vi "MICS Wakeup Calibration Tool.vi"(8 "error in (no error)":errorcluster, 10 "SECONDARY MICS Dongle Address":refnum<visa-resource-name>="COM8", 11 "PRIMARY MICS Dongle Address":refnum<visa-resource-name>="COM8") -> (0 "error out":errorcluster, 2 "Trim Settings":string)   [LabVIEW 2020]
panel:
  in  "Reject Ratio, %":i32=75
  in  "RSSI Gain":enum16{"1", "3", "10", "30"}(ring)
  in  "WakeupMode":bool=TRUE
  in  "DetTrim":bool=TRUE
  in  "Wakeup Signal Transmit":bool
  in  "Samples to Average":u8=5 format="%02d"
  out "Retries":u8 format="%02d"
  out "Loopback Data":u8 format="%02x"
  in  "Loopback Detector":bool
  in  "Update Radio Settings":bool
  in  "Done":bool
  in  "Do RSSI":bool
  out "RSSI Reading":u8(knob) scale=0.0..31.0 scale format="%x"
  in  "Detector Offset Trim":u8(knob)=31 scale=0.0..63.0 scale format="%x"
  in  "Wakeup Signal Power, dBm":dbl(knob)=-32.0 min=-32.25 max=0.0 step=0.25
  in  "RSSI Fine Trim":u8(knob)=16 scale=0.0..31.0 scale format="%x"
  in  "RX Antenna Tune":u8(knob)=7 scale=0.0..15.0 scale format="%x"
  in  "LNA Frequency Trim":u8(knob)=15 scale=0.0..31.0 scale format="%x"
  in  "LNA Gain Trim":u8(knob)=20 scale=0.0..63.0 scale format="%x"
  # "CW RF"
  # "Wakeup Packet"
  # "RF Trim"
  # "Detector Trim"
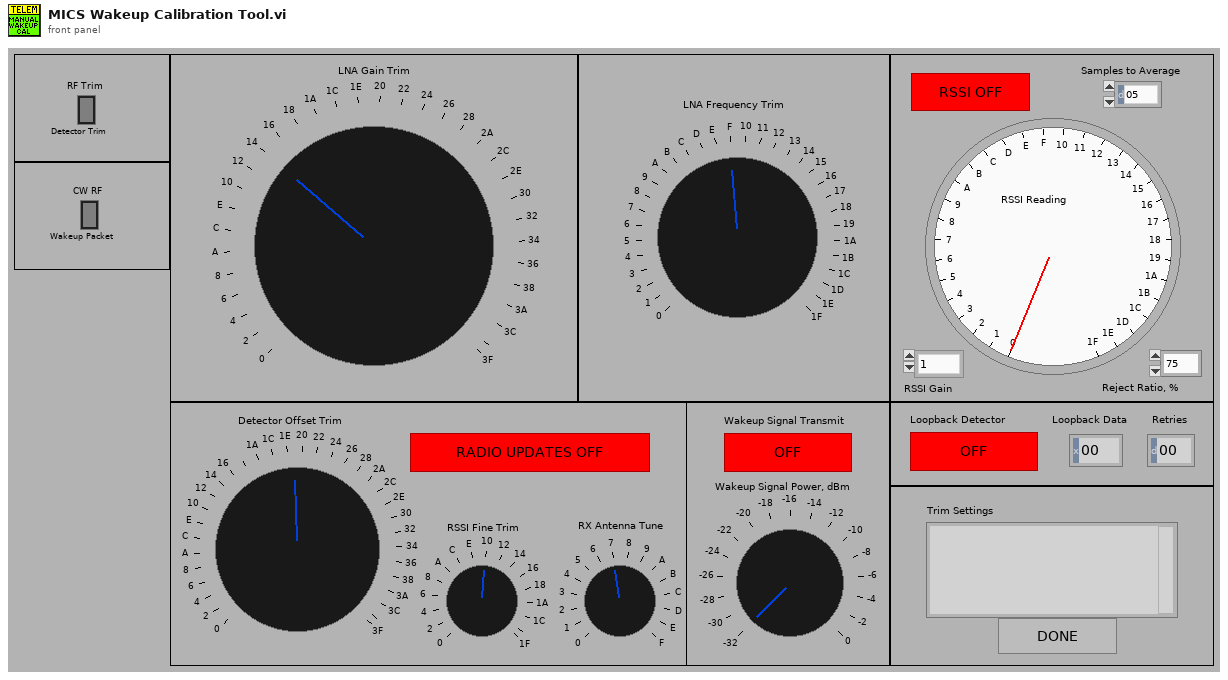
[diagram p1: front panel]
types:
  T1 = cluster{"ConfigFlags":u8, "ImplantID":u32, "CompanyID":u8, "Normal_Comm":cluster{"RF_Channel":u8, "UserData":u8, "TX_Mod":u8, "RX_Mod":u8, "RX_BlockSize":u8, "BlockPerPack":u8, "TX_BlockSize":u8}, "Emerg_Comm":cluster{"RF_Channel":u8, "UserData":u8, "TX_Mod":u8, "RX_Mod":u8, "TX_BlockSize":u8, "BlockPerPack":u8, "RX_BlockSize":u8}, "ImplantRev":u8, "245TX_PowerCal":i8, "245TX_Power":i8, "CCA_RSSI_Thresholds":cluster{"ch0":u16, "ch1":u16, "ch2":u16, "ch3":u16, "ch4":u16, "ch5":u16, "ch6":u16, "ch7":u16, "ch8":u16, "ch9":u16}}
  T2 = enum16{"Start Search", "Continue Search", "End Search"}
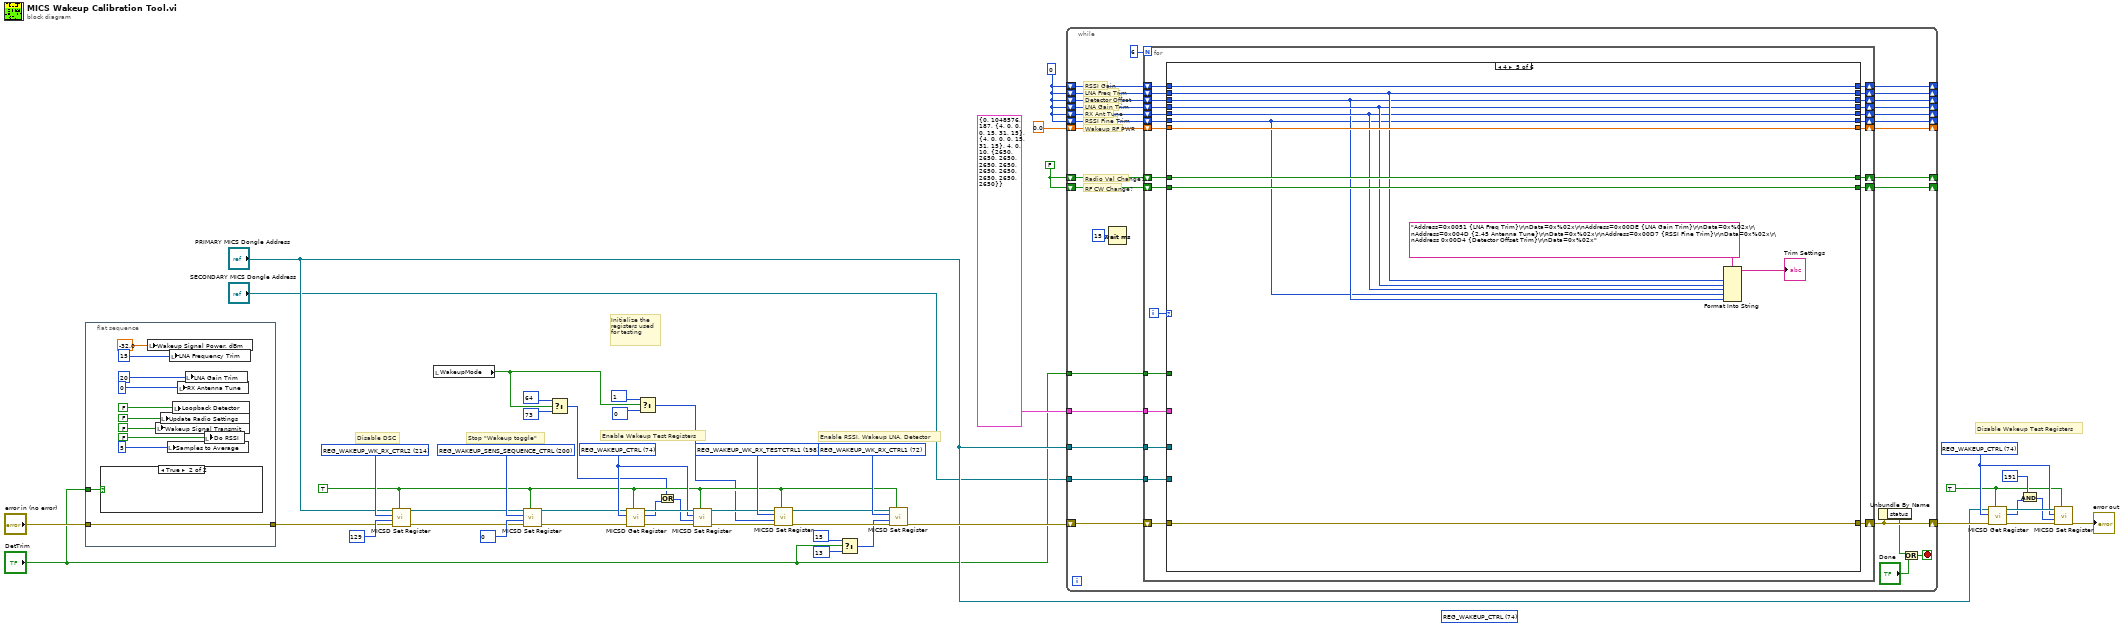
[diagram p0: block diagram]
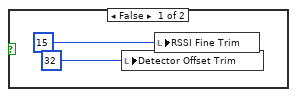
[diagram p2: hidden frame]
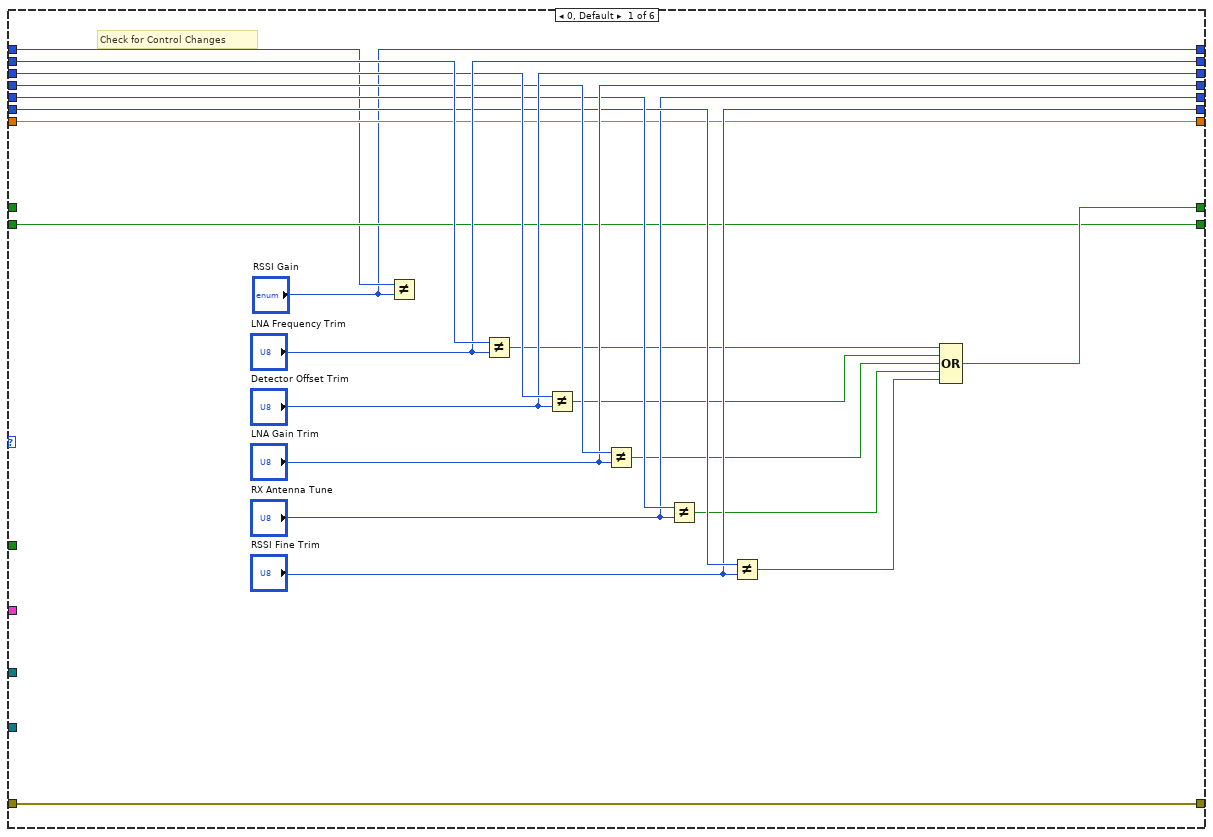
[diagram p3: hidden frame]
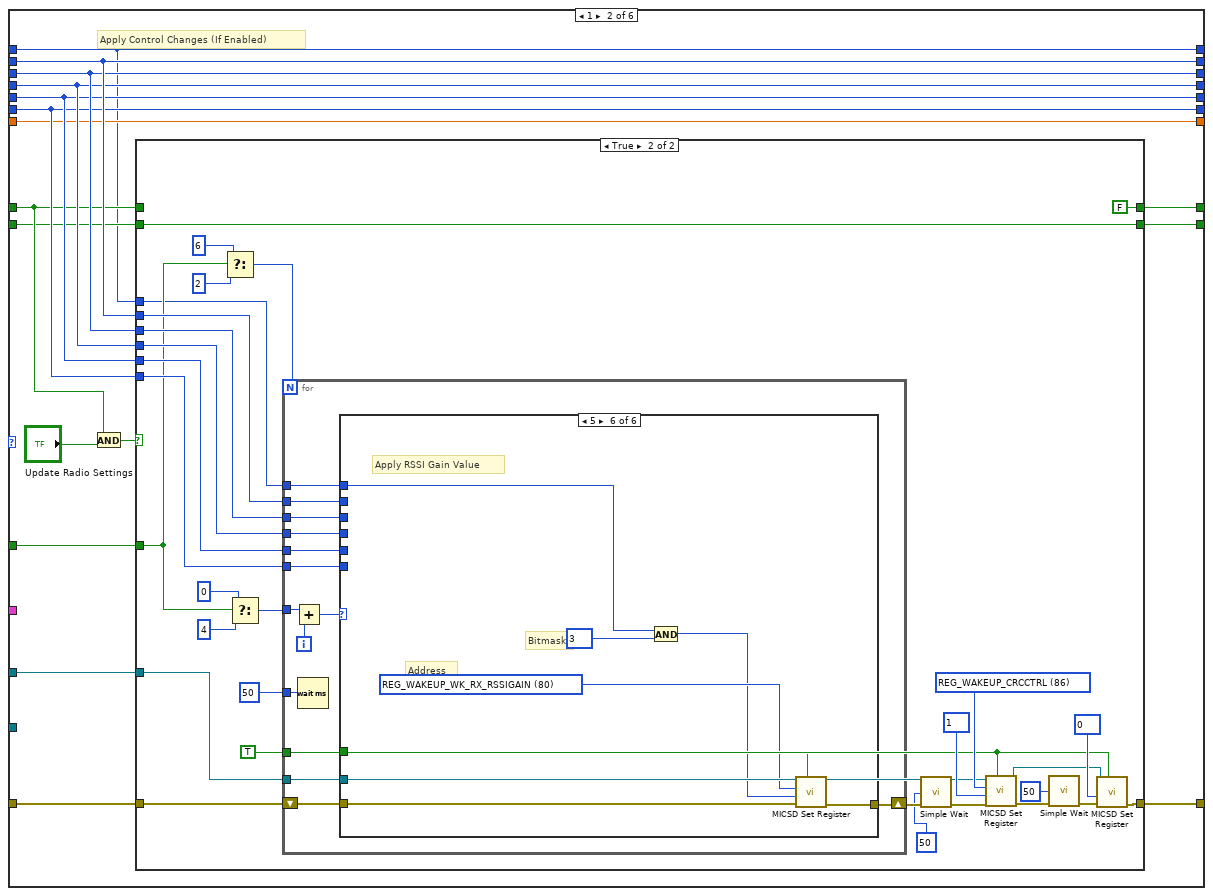
[diagram p4: hidden frame]
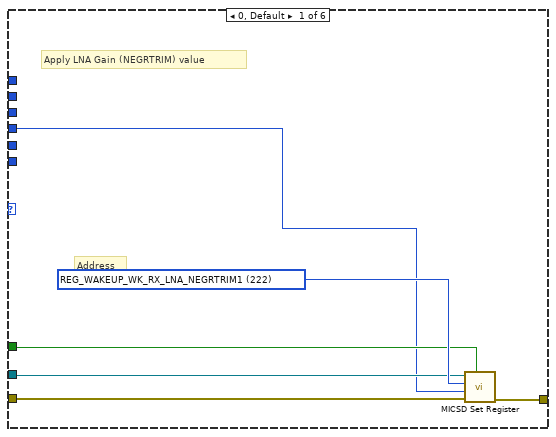
[diagram p6: hidden frame]
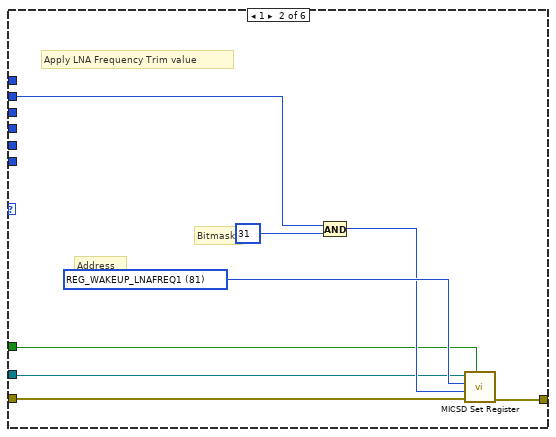
[diagram p7: hidden frame]
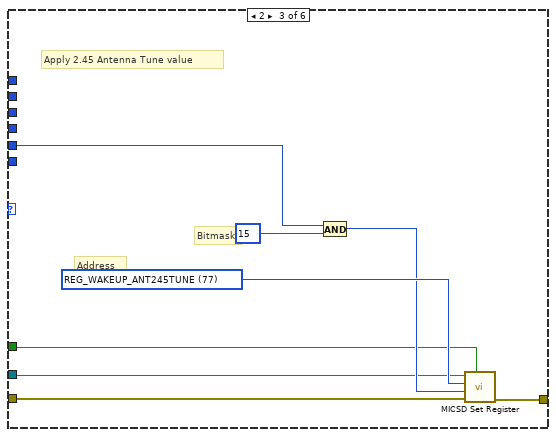
[diagram p8: hidden frame]
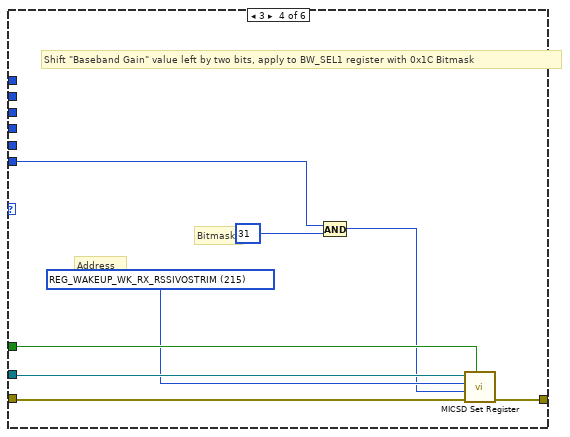
[diagram p9: hidden frame]
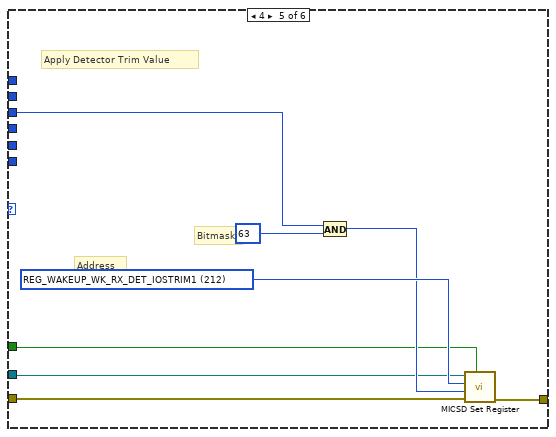
[diagram p10: hidden frame]
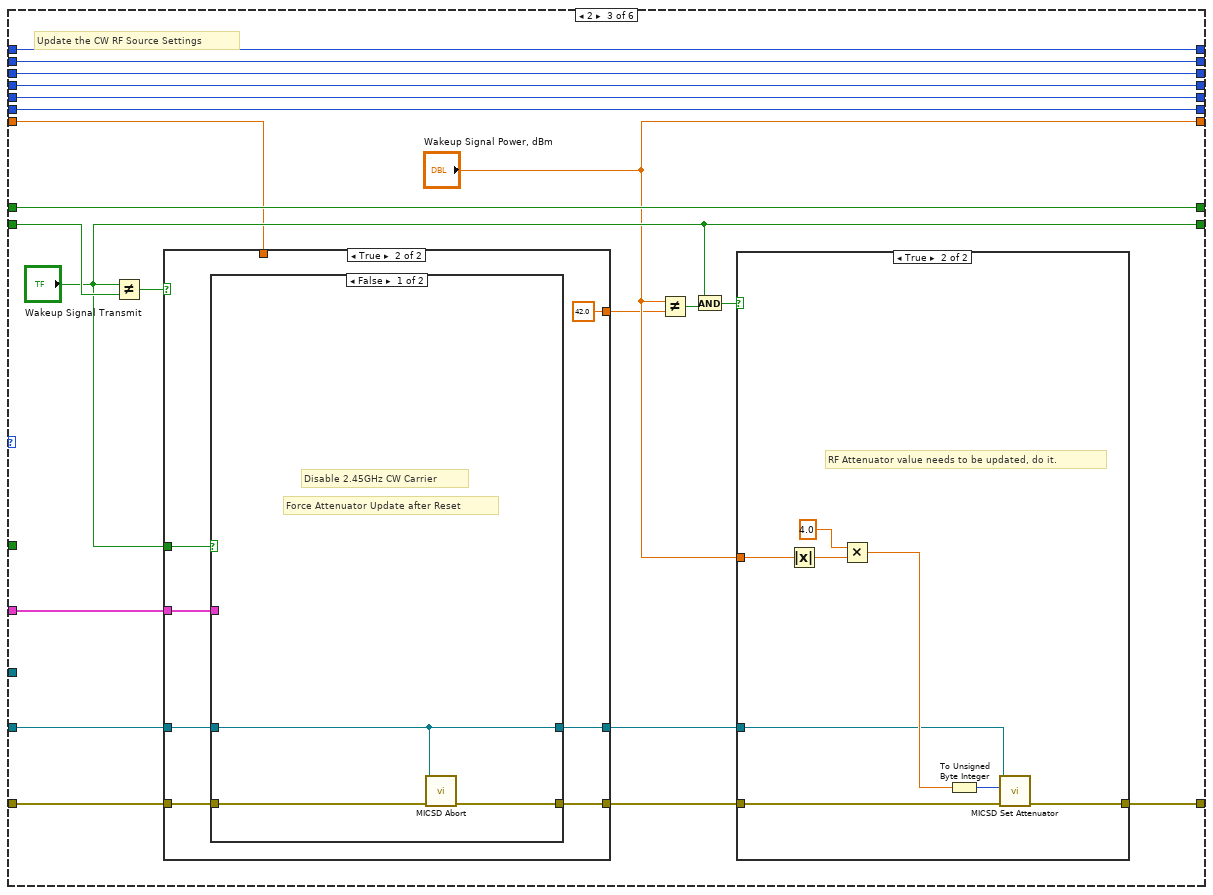
[diagram p11: hidden frame]
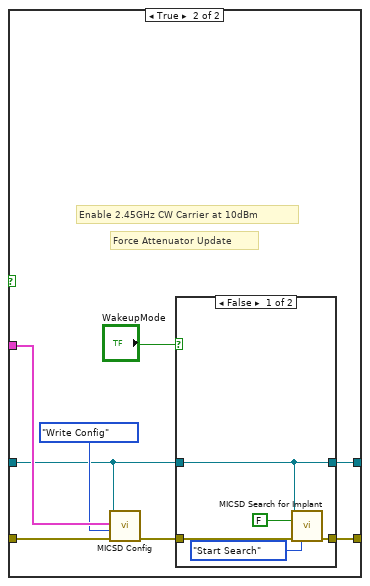
[diagram p14: hidden frame]
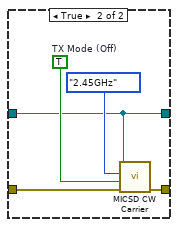
[diagram p15: hidden frame]
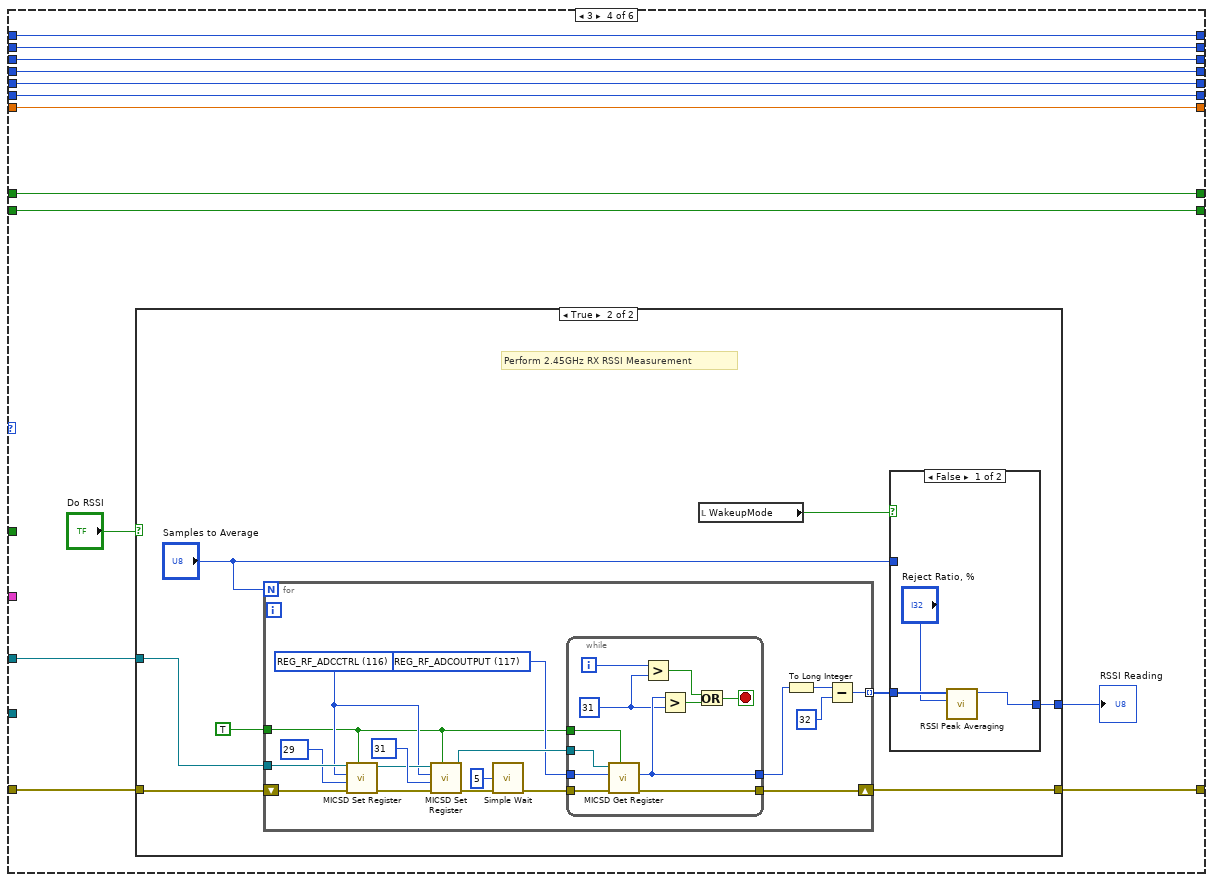
[diagram p16: hidden frame]
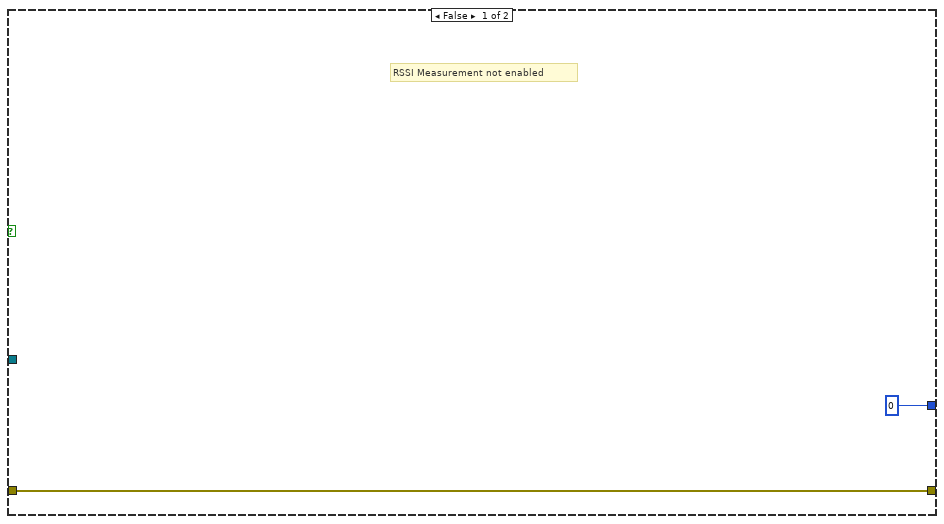
[diagram p17: hidden frame]
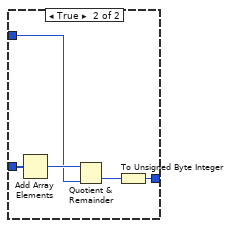
[diagram p18: hidden frame]
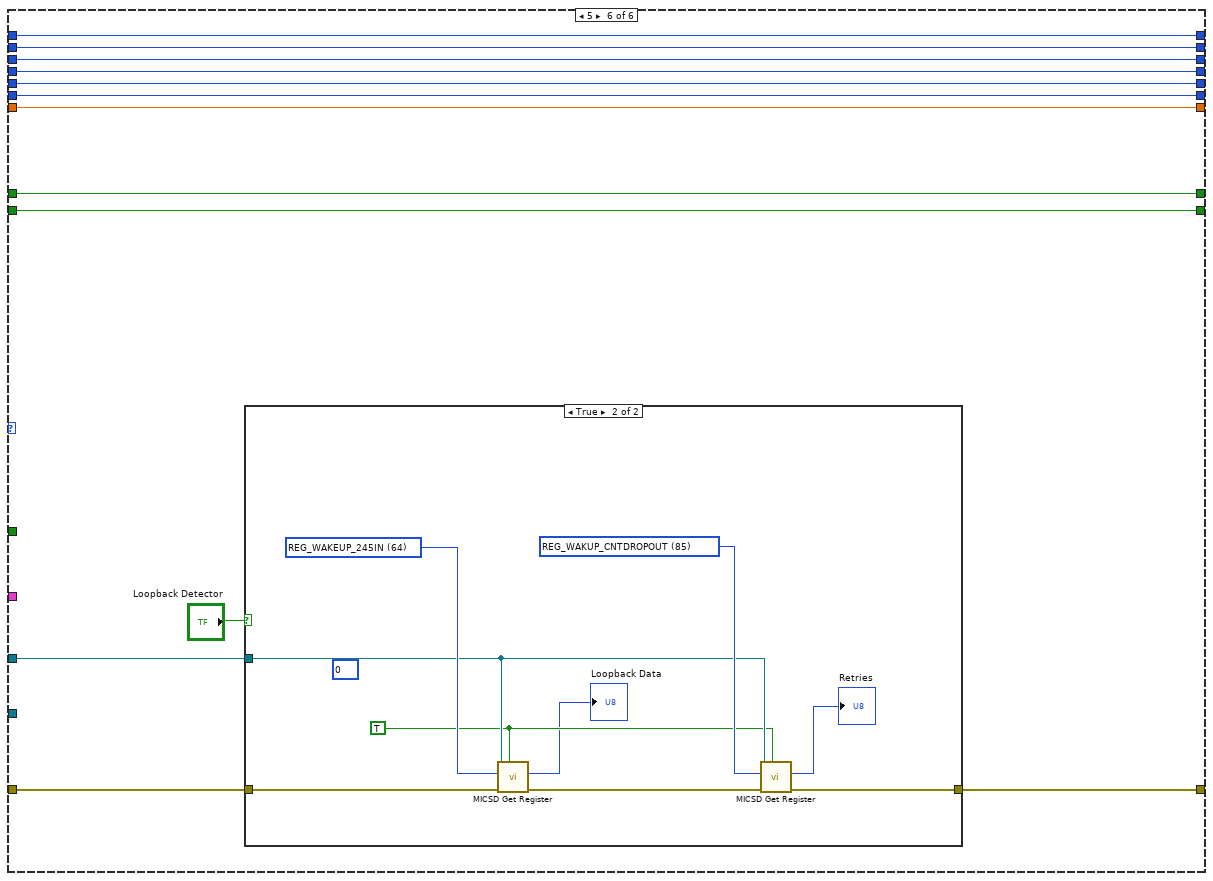
[diagram p19: hidden frame]
diagram:
  (unwired) u16 74 items=["---MANUAL ENTRY---"=1000, "REG_NOREG"=0, "REG_RXBUFF_USED"=1, "REG_RXBUFF_BSIZE"=2, "REG_TXBUFF_USED"=3, "REG_TXBUFF_BSIZE"=4, "REG_TXBUFF_MAXPACKSIZE"=5, "REG_MAC_ERRCLR"=6, "REG_MAC_TRAINNUM"=7, "REG_MAC_SYNCMATCH"=8, "REG_MAC_SYNC1"=9, "REG_MAC_SYNC2"=10, "REG_MAC_SYNC3"=11, "REG_MAC_SYNC4"=12, "REG_MAC_SYNC5"=13, "REG_MAC_MAXBERR"=14, "REG_MAC_ECCORR"=15, "REG_MAC_CRCERR"=16, "REG_MAC_BLKCNT1"=17, "REG_MAC_BLKCNT2"=18, "REG_MAC_IMDTRANSID1"=19, "REG_MAC_IMDTRANSID2"=20, "REG_MAC_IMDTRANSID3"=21, "REG_MAC_COMPANYID"=22, "REG_MAC_MODUSER"=23, "REG_MAC_CHANNEL"=25, "REG_MAC_CLEARWDOG"=26, "REG_MAC_CKCORRTHRESH"=27, "REG_HK_TXADDR"=28, "REG_HK_TXDATA"=29, "REG_HK_TXREPLY"=30, "REG_HK_USERDATA"=31, "REG_HK_USERSTATUS"=32, "REG_HK_LASTADDRESS"=33, "REG_HK_MODE"=34, "REG_MAC_STATUSSEQ"=35, "REG_MAC_MAXRETRIES"=36, "REG_MAC_RESENDTIME"=37, "REG_MAC_POWERSAVETIME"=38, "REG_MAC_HEAD_DET"=39, "REG_MAC_CTRL"=41, "REG_MAC_INITCOM"=42, "REG_INTERFACE_MODE"=43, "REG_TXRXBUFF_BOTH"=44, "REG_TXRXBUFF"=45, "REG_IRQ_RAWSTATUS1"=46, "REG_IRQ_ENABLE1"=47, "REG_IRQ_ENABLESET1"=48, "REG_IRQ_ENABLECLEAR1"=49, "REG_IRQ_RAWSTATUS2"=50, "REG_IRQ_ENABLE2"=51, "REG_IRQ_ENABLESET2"=52, "REG_IRQ_ENABLECLEAR2"=53, "REG_IRQ_STATUS1"=54, "REG_IRQ_STATUS2"=55, "REG_IRQ_AUXSTATUS"=56, "REG_TXBUFF_OVERFLOW"=57, "REG_PO0"=58, "REG_P01"=59, "REG_P02"=60, "REG_P03"=61, "REG_GP0"=62, "REG_GPI"=63, "REG_WAKEUP_245IN"=64, "REG_WAKEUP_COMPANYID"=65, "REG_WAKEUP_IMDTRANSID1"=66, "REG_WAKEUP_IMDTRANSID2"=67, "REG_WAKEUP_IMDTRANSID3"=68, "REG_WAKEUP_CHANNEL"=69, "REG_WAKEUP_MODUSER"=70, "REG_WAKEUP_DEVICEMODE"=71, "REG_WAKEUP_WK_RX_CTRL1"=72, "REG_WAKEUP_STACK_ADDR"=73, "REG_WAKEUP_CTRL"=74, "REG_WAKEUP_STROSCRTRIM"=75, "REG_WAKEUP_BIASTRIM"=76, "REG_WAKEUP_ANT245TUNE"=77, "REG_WAKEUP_WK_RX_RTRIMDET"=78, "REG_WAKEUP_WK_RX_RTRIMDEMOD"=79, "REG_WAKEUP_WK_RX_RSSIGAIN"=80, "REG_WAKEUP_LNAFREQ1"=81, "REG_WAKEUP_STACK"=83, "REG_WAKUP_XOSU"=84, "REG_WAKUP_CNTDROPOUT"=85, "REG_WAKEUP_CRCCTRL"=86, "REG_WAKEUP_CRCWORD1"=87, "REG_WAKEUP_CRCWORD2"=88, "REG_WAKEUP_WK_RX_CTRIM"=89, "REG_WAKEUP_VDDATRIM"=90, "REG_WAKEUP_VDDDTRIM"=91, "REG_WAKEUP_TESTIOBUFEN"=92, "REG_WAKEUP_TESTIOCLAMP"=93, "CORE_RESET_ADDRESS"=94, "CHIP_RESET_ADDRESS"=95, "REG_RF_TXGENCTRL"=96, "REG_RF_TXIFCTRL"=97, "REG_RF_TXRF_SEL_CTRL"=98, "REG_RF_TXRFPWRDEFAULTSET"=99, "REG_RF_RSSITRIM"=100, "REG_RF_TXIFOSCTUNE"=101, "REG_RF_TXIFGAINIMB"=102, "REG_RF_TXIFLOCK"=103, "REG_RF_RXRFLNAGAINTRIM"=104, "REG_RF_RXBIASTR"=105, "REG_RF_RXGENCTRL"=106, "REG_RF_RXIFADCDECLEV"=107, "REG_RF_RXIFDETFILTERTUNE"=108, "REG_RF_RXIFFILTERTUNE"=109, "REG_RF_GENENABLES"=110, "REG_RF_SYNTH_CHANNEL"=111, "REG_TX_RAMP_RTRIM"=112, "REG_TX_RAMP_CTRIM"=113, "REG_RF_XO_TRIM"=114, "REG_RF_SYNTH_SET_TRIM"=115, "REG_RF_ADCCTRL"=116, "REG_RF_ADCOUTPUT"=117, "REG_RF_TXIFAMP"=118, "REG_RF_SYNTH_RTRIM"=119, "REG_RF_SYNTH_CTRIM"=120, "REG_RF_SYNTH_CT"=121, "REG_RF_TXMIXER_IOSTRIM_HIGH_IP"=122, "REG_RF_TXMIXER_IOSTRIM_HIGH_IN"=123, "REG_RF_TXMIXER_IOSTRIM_HIGH_QP"=124, "REG_RF_TXMIXER_IOSTRIM_HIGH_QN"=125, "REG_HX_WUADDR"=126, "REG_REVISION"=127, "REG_NOREG_TEST"=128, "REG_DTEST_RXBUFF"=129, "REG_RXBUFF_NEXT_BLOCK"=130, "REG_RXBUFF_FIRST_IN_PACK"=131, "REG_RXBUFF_FIRST_EMPTY"=132, "REG_MAC_BYPASS"=133, "REG_DTEST_TXBUFF"=134, "REG_TXBUFF_NEXT_BLOCK"=135, "REG_TXBUFF_FIRST_IN_PACK"=136, "REG_TXBUFF_FIRST_EMPTY"=137, "REG_DTEST_SEQ"=138, "REG_DTEST_CKCORR"=139, "REG_MAC_TOPSTATE"=140, "REG_DTEST_INTERFACE"=141, "REG_IFACE_TXRX_BYPASS"=142, "REG_MAC_TXRXWAIT"=143, "REG_MAC_TXRFRAMP"=144, "REG_MAC_TRAINWORD"=145, "REG_MAC_TRAINWORD2"=146, "REG_MAC_SETTINGS"=147, "REG_MAC_CALSELECT1"=148, "REG_MAC_CALSELECT2"=149, "REG_MAC_ANTMATCHSEL"=150, "REG_MAC_ANTTUNESEL1"=151, "REG_MAC_ANTTUNESEL2"=152, "REG_MAC_ANTTUNESEL3"=153, "REG_MAC_ANTTUNESTEP"=154, "REG_MAC_WUMODEBURST"=156, "REG_MAC_WUOFFSHORT"=157, "REG_MAC_WUOFFLONG"=158, "REG_MAC_CLKRECCTRL"=159, "REG_HK_MODE_P2"=162, "REG_MAC_ANTTUNERES1"=164, "REG_MAC_ANTTUNERES2"=165, "REG_INTERFACE_MODE_TEST"=171, "REG_TXRXBUFF_BOTH_P2"=172, "REG_TXRXBUFF_P2"=173, "REG_IRQ_RAWSTATUS1_P2"=174, "REG_MAC_TXIFSTATUS1"=176, "REG_MAC_TXIFSTATUS2"=177, "REG_IRQ_RAWSTATUS2_P2"=178, "REG_MAC_TXIFRAMPDELAY"=179, "REG_MAC_TXIFRAMPSLOPE"=180, "REG_MAX_TXIFRAMP"=181, "REG_IRQ_STATUS1_P2"=182, "REG_IRQ_STATUS2_P2"=183, "REG_IRQ_AUXSTATUS_P2"=184, "REG_MAC_UNLOCK"=188, "REG_MAC_TXIFFREQ"=190, "REG_WAKEUP_TESTCTRL1"=192, "REG_WAKEUP_RX_EN_CNT"=193, "REG_WAKEUP_TESTENABLES"=194, "REG_WAKEUP_DTBI_CTRL"=195, "REG_WAKEUP_DTBO_CTRL"=196, "REG_WAKEUP_TESTIOBUFTEST"=197, "REG_WAKEUP_WK_RX_TESTCTRL1"=198, "REG_WAKEUP_WK_RX_TESTCTRL2"=199, "REG_WAKEUP_SENS_SEQUENCE_CTRL"=200, "REG_WAKEUP_LNABIAS"=201, "REG_WAKEUP_DET_TH_TRIM1"=202, "REG_WAKEUP_LNABIAS_NOM1"=203, "REG_WAKEUP_RX_TSHORT_TRIM1"=204, "REG_WAKEUP_LNABIAS_NOM2"=205, "REG_WAKEUP_RX_TLONG_TRIM1"=206, "REG_WAKEUP_LNA_NEGRTRIM_NOM1"=207, "REG_WAKEUP_RX_TBURST_TRIM1"=208, "REG_WAKEUP_RX_LNA_NEGRTRIM_NOM2"=209, "REG_WAKEUP_RX_BB_G_BW_SEL1"=210, "REG_WAKEUP_WK_RX_DET_IOSTRIM1"=212, "REG_WAKEUP_WK_RX_CTRL2"=214, "REG_WAKEUP_WK_RX_RSSIVOSTRIM"=215, "REG_WAKEUP_LNANEGR_EFF"=216, "REG_WAKEUP_XOSU_FAST"=217, "REG_WAKEUP_STROSCPWIDTH1"=218, "REG_WAKEUP_STROSCPERIOD1"=220, "REG_WAKEUP_STROSCPERIOD2"=221, "REG_WAKEUP_WK_RX_LNA_NEGRTRIM1"=222, "REG_RF_TXTESTENABLE"=224, "REG_RF_TXIFTESTMODE"=225, "REG_RF_RXTESTENABLE"=226, "REG_RF_RXIFTESTCTRL1"=227, "REG_RF_RXIFTESTCTRL2"=228, "REG_RF_RXIFTESTCTRL3"=229, "REG_RF_SYNTH_TESTCTRL1"=230, "REG_RF_SYNTH_TESTCTRL2"=231, "REG_RF_SYNTH_TESTCTRL3"=232, "REG_RF_ADCTEST1"=237, "REG_RF_ADCTEST2"=238, "REG_RF_TXMIXER_IOSTRIM_LOW_IP"=240, "REG_RF_TXMIXER_IOSTRIM_LOW_IN"=241, "REG_RF_TXMIXER_ISOTRIM_LOW_QP"=242, "REG_RF_TXMIXER_IOSTRIM_LOW_QN"=243, "REG_RF_SYNTH_KPD"=244, "REG_RF_SYNTH_LOLEV"=245, "REG_RF_TXRFPWRTUNEANTSET"=246, "REG_RF_TXPD_GAIN_CTRL"=247, "REG_RF_SYNTH_STARTUP"=248, "REG_RF_TXRFANTTUNE_TXMODE"=249, "REG_RF_TXRFANTTUNE_RXMODE"=250, "REG_RF_RXRFANTTUNE_TXMODE"=251, "REG_RF_RXRFANTTUNE_RXMODE"=252, "REG_ANTMATCH1"=253, "REG_ANTMATCH2"=254, "REG_REVISION_P2"=255] ("Register")
  w21 = u16 200 items=["---MANUAL ENTRY---"=1000, "REG_NOREG"=0, "REG_RXBUFF_USED"=1, "REG_RXBUFF_BSIZE"=2, "REG_TXBUFF_USED"=3, "REG_TXBUFF_BSIZE"=4, "REG_TXBUFF_MAXPACKSIZE"=5, "REG_MAC_ERRCLR"=6, "REG_MAC_TRAINNUM"=7, "REG_MAC_SYNCMATCH"=8, "REG_MAC_SYNC1"=9, "REG_MAC_SYNC2"=10, "REG_MAC_SYNC3"=11, "REG_MAC_SYNC4"=12, "REG_MAC_SYNC5"=13, "REG_MAC_MAXBERR"=14, "REG_MAC_ECCORR"=15, "REG_MAC_CRCERR"=16, "REG_MAC_BLKCNT1"=17, "REG_MAC_BLKCNT2"=18, "REG_MAC_IMDTRANSID1"=19, "REG_MAC_IMDTRANSID2"=20, "REG_MAC_IMDTRANSID3"=21, "REG_MAC_COMPANYID"=22, "REG_MAC_MODUSER"=23, "REG_MAC_CHANNEL"=25, "REG_MAC_CLEARWDOG"=26, "REG_MAC_CKCORRTHRESH"=27, "REG_HK_TXADDR"=28, "REG_HK_TXDATA"=29, "REG_HK_TXREPLY"=30, "REG_HK_USERDATA"=31, "REG_HK_USERSTATUS"=32, "REG_HK_LASTADDRESS"=33, "REG_HK_MODE"=34, "REG_MAC_STATUSSEQ"=35, "REG_MAC_MAXRETRIES"=36, "REG_MAC_RESENDTIME"=37, "REG_MAC_POWERSAVETIME"=38, "REG_MAC_HEAD_DET"=39, "REG_MAC_CTRL"=41, "REG_MAC_INITCOM"=42, "REG_INTERFACE_MODE"=43, "REG_TXRXBUFF_BOTH"=44, "REG_TXRXBUFF"=45, "REG_IRQ_RAWSTATUS1"=46, "REG_IRQ_ENABLE1"=47, "REG_IRQ_ENABLESET1"=48, "REG_IRQ_ENABLECLEAR1"=49, "REG_IRQ_RAWSTATUS2"=50, "REG_IRQ_ENABLE2"=51, "REG_IRQ_ENABLESET2"=52, "REG_IRQ_ENABLECLEAR2"=53, "REG_IRQ_STATUS1"=54, "REG_IRQ_STATUS2"=55, "REG_IRQ_AUXSTATUS"=56, "REG_TXBUFF_OVERFLOW"=57, "REG_PO0"=58, "REG_P01"=59, "REG_P02"=60, "REG_P03"=61, "REG_GP0"=62, "REG_GPI"=63, "REG_WAKEUP_245IN"=64, "REG_WAKEUP_COMPANYID"=65, "REG_WAKEUP_IMDTRANSID1"=66, "REG_WAKEUP_IMDTRANSID2"=67, "REG_WAKEUP_IMDTRANSID3"=68, "REG_WAKEUP_CHANNEL"=69, "REG_WAKEUP_MODUSER"=70, "REG_WAKEUP_DEVICEMODE"=71, "REG_WAKEUP_WK_RX_CTRL1"=72, "REG_WAKEUP_STACK_ADDR"=73, "REG_WAKEUP_CTRL"=74, "REG_WAKEUP_STROSCRTRIM"=75, "REG_WAKEUP_BIASTRIM"=76, "REG_WAKEUP_ANT245TUNE"=77, "REG_WAKEUP_WK_RX_RTRIMDET"=78, "REG_WAKEUP_WK_RX_RTRIMDEMOD"=79, "REG_WAKEUP_WK_RX_RSSIGAIN"=80, "REG_WAKEUP_LNAFREQ1"=81, "REG_WAKEUP_STACK"=83, "REG_WAKUP_XOSU"=84, "REG_WAKUP_CNTDROPOUT"=85, "REG_WAKEUP_CRCCTRL"=86, "REG_WAKEUP_CRCWORD1"=87, "REG_WAKEUP_CRCWORD2"=88, "REG_WAKEUP_WK_RX_CTRIM"=89, "REG_WAKEUP_VDDATRIM"=90, "REG_WAKEUP_VDDDTRIM"=91, "REG_WAKEUP_TESTIOBUFEN"=92, "REG_WAKEUP_TESTIOCLAMP"=93, "CORE_RESET_ADDRESS"=94, "CHIP_RESET_ADDRESS"=95, "REG_RF_TXGENCTRL"=96, "REG_RF_TXIFCTRL"=97, "REG_RF_TXRF_SEL_CTRL"=98, "REG_RF_TXRFPWRDEFAULTSET"=99, "REG_RF_RSSITRIM"=100, "REG_RF_TXIFOSCTUNE"=101, "REG_RF_TXIFGAINIMB"=102, "REG_RF_TXIFLOCK"=103, "REG_RF_RXRFLNAGAINTRIM"=104, "REG_RF_RXBIASTR"=105, "REG_RF_RXGENCTRL"=106, "REG_RF_RXIFADCDECLEV"=107, "REG_RF_RXIFDETFILTERTUNE"=108, "REG_RF_RXIFFILTERTUNE"=109, "REG_RF_GENENABLES"=110, "REG_RF_SYNTH_CHANNEL"=111, "REG_TX_RAMP_RTRIM"=112, "REG_TX_RAMP_CTRIM"=113, "REG_RF_XO_TRIM"=114, "REG_RF_SYNTH_SET_TRIM"=115, "REG_RF_ADCCTRL"=116, "REG_RF_ADCOUTPUT"=117, "REG_RF_TXIFAMP"=118, "REG_RF_SYNTH_RTRIM"=119, "REG_RF_SYNTH_CTRIM"=120, "REG_RF_SYNTH_CT"=121, "REG_RF_TXMIXER_IOSTRIM_HIGH_IP"=122, "REG_RF_TXMIXER_IOSTRIM_HIGH_IN"=123, "REG_RF_TXMIXER_IOSTRIM_HIGH_QP"=124, "REG_RF_TXMIXER_IOSTRIM_HIGH_QN"=125, "REG_HX_WUADDR"=126, "REG_REVISION"=127, "REG_NOREG_TEST"=128, "REG_DTEST_RXBUFF"=129, "REG_RXBUFF_NEXT_BLOCK"=130, "REG_RXBUFF_FIRST_IN_PACK"=131, "REG_RXBUFF_FIRST_EMPTY"=132, "REG_MAC_BYPASS"=133, "REG_DTEST_TXBUFF"=134, "REG_TXBUFF_NEXT_BLOCK"=135, "REG_TXBUFF_FIRST_IN_PACK"=136, "REG_TXBUFF_FIRST_EMPTY"=137, "REG_DTEST_SEQ"=138, "REG_DTEST_CKCORR"=139, "REG_MAC_TOPSTATE"=140, "REG_DTEST_INTERFACE"=141, "REG_IFACE_TXRX_BYPASS"=142, "REG_MAC_TXRXWAIT"=143, "REG_MAC_TXRFRAMP"=144, "REG_MAC_TRAINWORD"=145, "REG_MAC_TRAINWORD2"=146, "REG_MAC_SETTINGS"=147, "REG_MAC_CALSELECT1"=148, "REG_MAC_CALSELECT2"=149, "REG_MAC_ANTMATCHSEL"=150, "REG_MAC_ANTTUNESEL1"=151, "REG_MAC_ANTTUNESEL2"=152, "REG_MAC_ANTTUNESEL3"=153, "REG_MAC_ANTTUNESTEP"=154, "REG_MAC_WUMODEBURST"=156, "REG_MAC_WUOFFSHORT"=157, "REG_MAC_WUOFFLONG"=158, "REG_MAC_CLKRECCTRL"=159, "REG_HK_MODE_P2"=162, "REG_MAC_ANTTUNERES1"=164, "REG_MAC_ANTTUNERES2"=165, "REG_INTERFACE_MODE_TEST"=171, "REG_TXRXBUFF_BOTH_P2"=172, "REG_TXRXBUFF_P2"=173, "REG_IRQ_RAWSTATUS1_P2"=174, "REG_MAC_TXIFSTATUS1"=176, "REG_MAC_TXIFSTATUS2"=177, "REG_IRQ_RAWSTATUS2_P2"=178, "REG_MAC_TXIFRAMPDELAY"=179, "REG_MAC_TXIFRAMPSLOPE"=180, "REG_MAX_TXIFRAMP"=181, "REG_IRQ_STATUS1_P2"=182, "REG_IRQ_STATUS2_P2"=183, "REG_IRQ_AUXSTATUS_P2"=184, "REG_MAC_UNLOCK"=188, "REG_MAC_TXIFFREQ"=190, "REG_WAKEUP_TESTCTRL1"=192, "REG_WAKEUP_RX_EN_CNT"=193, "REG_WAKEUP_TESTENABLES"=194, "REG_WAKEUP_DTBI_CTRL"=195, "REG_WAKEUP_DTBO_CTRL"=196, "REG_WAKEUP_TESTIOBUFTEST"=197, "REG_WAKEUP_WK_RX_TESTCTRL1"=198, "REG_WAKEUP_WK_RX_TESTCTRL2"=199, "REG_WAKEUP_SENS_SEQUENCE_CTRL"=200, "REG_WAKEUP_LNABIAS"=201, "REG_WAKEUP_DET_TH_TRIM1"=202, "REG_WAKEUP_LNABIAS_NOM1"=203, "REG_WAKEUP_RX_TSHORT_TRIM1"=204, "REG_WAKEUP_LNABIAS_NOM2"=205, "REG_WAKEUP_RX_TLONG_TRIM1"=206, "REG_WAKEUP_LNA_NEGRTRIM_NOM1"=207, "REG_WAKEUP_RX_TBURST_TRIM1"=208, "REG_WAKEUP_RX_LNA_NEGRTRIM_NOM2"=209, "REG_WAKEUP_RX_BB_G_BW_SEL1"=210, "REG_WAKEUP_WK_RX_DET_IOSTRIM1"=212, "REG_WAKEUP_WK_RX_CTRL2"=214, "REG_WAKEUP_WK_RX_RSSIVOSTRIM"=215, "REG_WAKEUP_LNANEGR_EFF"=216, "REG_WAKEUP_XOSU_FAST"=217, "REG_WAKEUP_STROSCPWIDTH1"=218, "REG_WAKEUP_STROSCPERIOD1"=220, "REG_WAKEUP_STROSCPERIOD2"=221, "REG_WAKEUP_WK_RX_LNA_NEGRTRIM1"=222, "REG_RF_TXTESTENABLE"=224, "REG_RF_TXIFTESTMODE"=225, "REG_RF_RXTESTENABLE"=226, "REG_RF_RXIFTESTCTRL1"=227, "REG_RF_RXIFTESTCTRL2"=228, "REG_RF_RXIFTESTCTRL3"=229, "REG_RF_SYNTH_TESTCTRL1"=230, "REG_RF_SYNTH_TESTCTRL2"=231, "REG_RF_SYNTH_TESTCTRL3"=232, "REG_RF_ADCTEST1"=237, "REG_RF_ADCTEST2"=238, "REG_RF_TXMIXER_IOSTRIM_LOW_IP"=240, "REG_RF_TXMIXER_IOSTRIM_LOW_IN"=241, "REG_RF_TXMIXER_ISOTRIM_LOW_QP"=242, "REG_RF_TXMIXER_IOSTRIM_LOW_QN"=243, "REG_RF_SYNTH_KPD"=244, "REG_RF_SYNTH_LOLEV"=245, "REG_RF_TXRFPWRTUNEANTSET"=246, "REG_RF_TXPD_GAIN_CTRL"=247, "REG_RF_SYNTH_STARTUP"=248, "REG_RF_TXRFANTTUNE_TXMODE"=249, "REG_RF_TXRFANTTUNE_RXMODE"=250, "REG_RF_RXRFANTTUNE_TXMODE"=251, "REG_RF_RXRFANTTUNE_RXMODE"=252, "REG_ANTMATCH1"=253, "REG_ANTMATCH2"=254, "REG_REVISION_P2"=255] ("Register")
  w25 = u16 214 items=["---MANUAL ENTRY---"=1000, "REG_NOREG"=0, "REG_RXBUFF_USED"=1, "REG_RXBUFF_BSIZE"=2, "REG_TXBUFF_USED"=3, "REG_TXBUFF_BSIZE"=4, "REG_TXBUFF_MAXPACKSIZE"=5, "REG_MAC_ERRCLR"=6, "REG_MAC_TRAINNUM"=7, "REG_MAC_SYNCMATCH"=8, "REG_MAC_SYNC1"=9, "REG_MAC_SYNC2"=10, "REG_MAC_SYNC3"=11, "REG_MAC_SYNC4"=12, "REG_MAC_SYNC5"=13, "REG_MAC_MAXBERR"=14, "REG_MAC_ECCORR"=15, "REG_MAC_CRCERR"=16, "REG_MAC_BLKCNT1"=17, "REG_MAC_BLKCNT2"=18, "REG_MAC_IMDTRANSID1"=19, "REG_MAC_IMDTRANSID2"=20, "REG_MAC_IMDTRANSID3"=21, "REG_MAC_COMPANYID"=22, "REG_MAC_MODUSER"=23, "REG_MAC_CHANNEL"=25, "REG_MAC_CLEARWDOG"=26, "REG_MAC_CKCORRTHRESH"=27, "REG_HK_TXADDR"=28, "REG_HK_TXDATA"=29, "REG_HK_TXREPLY"=30, "REG_HK_USERDATA"=31, "REG_HK_USERSTATUS"=32, "REG_HK_LASTADDRESS"=33, "REG_HK_MODE"=34, "REG_MAC_STATUSSEQ"=35, "REG_MAC_MAXRETRIES"=36, "REG_MAC_RESENDTIME"=37, "REG_MAC_POWERSAVETIME"=38, "REG_MAC_HEAD_DET"=39, "REG_MAC_CTRL"=41, "REG_MAC_INITCOM"=42, "REG_INTERFACE_MODE"=43, "REG_TXRXBUFF_BOTH"=44, "REG_TXRXBUFF"=45, "REG_IRQ_RAWSTATUS1"=46, "REG_IRQ_ENABLE1"=47, "REG_IRQ_ENABLESET1"=48, "REG_IRQ_ENABLECLEAR1"=49, "REG_IRQ_RAWSTATUS2"=50, "REG_IRQ_ENABLE2"=51, "REG_IRQ_ENABLESET2"=52, "REG_IRQ_ENABLECLEAR2"=53, "REG_IRQ_STATUS1"=54, "REG_IRQ_STATUS2"=55, "REG_IRQ_AUXSTATUS"=56, "REG_TXBUFF_OVERFLOW"=57, "REG_PO0"=58, "REG_P01"=59, "REG_P02"=60, "REG_P03"=61, "REG_GP0"=62, "REG_GPI"=63, "REG_WAKEUP_245IN"=64, "REG_WAKEUP_COMPANYID"=65, "REG_WAKEUP_IMDTRANSID1"=66, "REG_WAKEUP_IMDTRANSID2"=67, "REG_WAKEUP_IMDTRANSID3"=68, "REG_WAKEUP_CHANNEL"=69, "REG_WAKEUP_MODUSER"=70, "REG_WAKEUP_DEVICEMODE"=71, "REG_WAKEUP_WK_RX_CTRL1"=72, "REG_WAKEUP_STACK_ADDR"=73, "REG_WAKEUP_CTRL"=74, "REG_WAKEUP_STROSCRTRIM"=75, "REG_WAKEUP_BIASTRIM"=76, "REG_WAKEUP_ANT245TUNE"=77, "REG_WAKEUP_WK_RX_RTRIMDET"=78, "REG_WAKEUP_WK_RX_RTRIMDEMOD"=79, "REG_WAKEUP_WK_RX_RSSIGAIN"=80, "REG_WAKEUP_LNAFREQ1"=81, "REG_WAKEUP_STACK"=83, "REG_WAKUP_XOSU"=84, "REG_WAKUP_CNTDROPOUT"=85, "REG_WAKEUP_CRCCTRL"=86, "REG_WAKEUP_CRCWORD1"=87, "REG_WAKEUP_CRCWORD2"=88, "REG_WAKEUP_WK_RX_CTRIM"=89, "REG_WAKEUP_VDDATRIM"=90, "REG_WAKEUP_VDDDTRIM"=91, "REG_WAKEUP_TESTIOBUFEN"=92, "REG_WAKEUP_TESTIOCLAMP"=93, "CORE_RESET_ADDRESS"=94, "CHIP_RESET_ADDRESS"=95, "REG_RF_TXGENCTRL"=96, "REG_RF_TXIFCTRL"=97, "REG_RF_TXRF_SEL_CTRL"=98, "REG_RF_TXRFPWRDEFAULTSET"=99, "REG_RF_RSSITRIM"=100, "REG_RF_TXIFOSCTUNE"=101, "REG_RF_TXIFGAINIMB"=102, "REG_RF_TXIFLOCK"=103, "REG_RF_RXRFLNAGAINTRIM"=104, "REG_RF_RXBIASTR"=105, "REG_RF_RXGENCTRL"=106, "REG_RF_RXIFADCDECLEV"=107, "REG_RF_RXIFDETFILTERTUNE"=108, "REG_RF_RXIFFILTERTUNE"=109, "REG_RF_GENENABLES"=110, "REG_RF_SYNTH_CHANNEL"=111, "REG_TX_RAMP_RTRIM"=112, "REG_TX_RAMP_CTRIM"=113, "REG_RF_XO_TRIM"=114, "REG_RF_SYNTH_SET_TRIM"=115, "REG_RF_ADCCTRL"=116, "REG_RF_ADCOUTPUT"=117, "REG_RF_TXIFAMP"=118, "REG_RF_SYNTH_RTRIM"=119, "REG_RF_SYNTH_CTRIM"=120, "REG_RF_SYNTH_CT"=121, "REG_RF_TXMIXER_IOSTRIM_HIGH_IP"=122, "REG_RF_TXMIXER_IOSTRIM_HIGH_IN"=123, "REG_RF_TXMIXER_IOSTRIM_HIGH_QP"=124, "REG_RF_TXMIXER_IOSTRIM_HIGH_QN"=125, "REG_HX_WUADDR"=126, "REG_REVISION"=127, "REG_NOREG_TEST"=128, "REG_DTEST_RXBUFF"=129, "REG_RXBUFF_NEXT_BLOCK"=130, "REG_RXBUFF_FIRST_IN_PACK"=131, "REG_RXBUFF_FIRST_EMPTY"=132, "REG_MAC_BYPASS"=133, "REG_DTEST_TXBUFF"=134, "REG_TXBUFF_NEXT_BLOCK"=135, "REG_TXBUFF_FIRST_IN_PACK"=136, "REG_TXBUFF_FIRST_EMPTY"=137, "REG_DTEST_SEQ"=138, "REG_DTEST_CKCORR"=139, "REG_MAC_TOPSTATE"=140, "REG_DTEST_INTERFACE"=141, "REG_IFACE_TXRX_BYPASS"=142, "REG_MAC_TXRXWAIT"=143, "REG_MAC_TXRFRAMP"=144, "REG_MAC_TRAINWORD"=145, "REG_MAC_TRAINWORD2"=146, "REG_MAC_SETTINGS"=147, "REG_MAC_CALSELECT1"=148, "REG_MAC_CALSELECT2"=149, "REG_MAC_ANTMATCHSEL"=150, "REG_MAC_ANTTUNESEL1"=151, "REG_MAC_ANTTUNESEL2"=152, "REG_MAC_ANTTUNESEL3"=153, "REG_MAC_ANTTUNESTEP"=154, "REG_MAC_WUMODEBURST"=156, "REG_MAC_WUOFFSHORT"=157, "REG_MAC_WUOFFLONG"=158, "REG_MAC_CLKRECCTRL"=159, "REG_HK_MODE_P2"=162, "REG_MAC_ANTTUNERES1"=164, "REG_MAC_ANTTUNERES2"=165, "REG_INTERFACE_MODE_TEST"=171, "REG_TXRXBUFF_BOTH_P2"=172, "REG_TXRXBUFF_P2"=173, "REG_IRQ_RAWSTATUS1_P2"=174, "REG_MAC_TXIFSTATUS1"=176, "REG_MAC_TXIFSTATUS2"=177, "REG_IRQ_RAWSTATUS2_P2"=178, "REG_MAC_TXIFRAMPDELAY"=179, "REG_MAC_TXIFRAMPSLOPE"=180, "REG_MAX_TXIFRAMP"=181, "REG_IRQ_STATUS1_P2"=182, "REG_IRQ_STATUS2_P2"=183, "REG_IRQ_AUXSTATUS_P2"=184, "REG_MAC_UNLOCK"=188, "REG_MAC_TXIFFREQ"=190, "REG_WAKEUP_TESTCTRL1"=192, "REG_WAKEUP_RX_EN_CNT"=193, "REG_WAKEUP_TESTENABLES"=194, "REG_WAKEUP_DTBI_CTRL"=195, "REG_WAKEUP_DTBO_CTRL"=196, "REG_WAKEUP_TESTIOBUFTEST"=197, "REG_WAKEUP_WK_RX_TESTCTRL1"=198, "REG_WAKEUP_WK_RX_TESTCTRL2"=199, "REG_WAKEUP_SENS_SEQUENCE_CTRL"=200, "REG_WAKEUP_LNABIAS"=201, "REG_WAKEUP_DET_TH_TRIM1"=202, "REG_WAKEUP_LNABIAS_NOM1"=203, "REG_WAKEUP_RX_TSHORT_TRIM1"=204, "REG_WAKEUP_LNABIAS_NOM2"=205, "REG_WAKEUP_RX_TLONG_TRIM1"=206, "REG_WAKEUP_LNA_NEGRTRIM_NOM1"=207, "REG_WAKEUP_RX_TBURST_TRIM1"=208, "REG_WAKEUP_RX_LNA_NEGRTRIM_NOM2"=209, "REG_WAKEUP_RX_BB_G_BW_SEL1"=210, "REG_WAKEUP_WK_RX_DET_IOSTRIM1"=212, "REG_WAKEUP_WK_RX_CTRL2"=214, "REG_WAKEUP_WK_RX_RSSIVOSTRIM"=215, "REG_WAKEUP_LNANEGR_EFF"=216, "REG_WAKEUP_XOSU_FAST"=217, "REG_WAKEUP_STROSCPWIDTH1"=218, "REG_WAKEUP_STROSCPERIOD1"=220, "REG_WAKEUP_STROSCPERIOD2"=221, "REG_WAKEUP_WK_RX_LNA_NEGRTRIM1"=222, "REG_RF_TXTESTENABLE"=224, "REG_RF_TXIFTESTMODE"=225, "REG_RF_RXTESTENABLE"=226, "REG_RF_RXIFTESTCTRL1"=227, "REG_RF_RXIFTESTCTRL2"=228, "REG_RF_RXIFTESTCTRL3"=229, "REG_RF_SYNTH_TESTCTRL1"=230, "REG_RF_SYNTH_TESTCTRL2"=231, "REG_RF_SYNTH_TESTCTRL3"=232, "REG_RF_ADCTEST1"=237, "REG_RF_ADCTEST2"=238, "REG_RF_TXMIXER_IOSTRIM_LOW_IP"=240, "REG_RF_TXMIXER_IOSTRIM_LOW_IN"=241, "REG_RF_TXMIXER_ISOTRIM_LOW_QP"=242, "REG_RF_TXMIXER_IOSTRIM_LOW_QN"=243, "REG_RF_SYNTH_KPD"=244, "REG_RF_SYNTH_LOLEV"=245, "REG_RF_TXRFPWRTUNEANTSET"=246, "REG_RF_TXPD_GAIN_CTRL"=247, "REG_RF_SYNTH_STARTUP"=248, "REG_RF_TXRFANTTUNE_TXMODE"=249, "REG_RF_TXRFANTTUNE_RXMODE"=250, "REG_RF_RXRFANTTUNE_TXMODE"=251, "REG_RF_RXRFANTTUNE_RXMODE"=252, "REG_ANTMATCH1"=253, "REG_ANTMATCH2"=254, "REG_REVISION_P2"=255] ("Register")
  w27 = TRUE
  w29 = u16 74 items=["---MANUAL ENTRY---"=1000, "REG_NOREG"=0, "REG_RXBUFF_USED"=1, "REG_RXBUFF_BSIZE"=2, "REG_TXBUFF_USED"=3, "REG_TXBUFF_BSIZE"=4, "REG_TXBUFF_MAXPACKSIZE"=5, "REG_MAC_ERRCLR"=6, "REG_MAC_TRAINNUM"=7, "REG_MAC_SYNCMATCH"=8, "REG_MAC_SYNC1"=9, "REG_MAC_SYNC2"=10, "REG_MAC_SYNC3"=11, "REG_MAC_SYNC4"=12, "REG_MAC_SYNC5"=13, "REG_MAC_MAXBERR"=14, "REG_MAC_ECCORR"=15, "REG_MAC_CRCERR"=16, "REG_MAC_BLKCNT1"=17, "REG_MAC_BLKCNT2"=18, "REG_MAC_IMDTRANSID1"=19, "REG_MAC_IMDTRANSID2"=20, "REG_MAC_IMDTRANSID3"=21, "REG_MAC_COMPANYID"=22, "REG_MAC_MODUSER"=23, "REG_MAC_CHANNEL"=25, "REG_MAC_CLEARWDOG"=26, "REG_MAC_CKCORRTHRESH"=27, "REG_HK_TXADDR"=28, "REG_HK_TXDATA"=29, "REG_HK_TXREPLY"=30, "REG_HK_USERDATA"=31, "REG_HK_USERSTATUS"=32, "REG_HK_LASTADDRESS"=33, "REG_HK_MODE"=34, "REG_MAC_STATUSSEQ"=35, "REG_MAC_MAXRETRIES"=36, "REG_MAC_RESENDTIME"=37, "REG_MAC_POWERSAVETIME"=38, "REG_MAC_HEAD_DET"=39, "REG_MAC_CTRL"=41, "REG_MAC_INITCOM"=42, "REG_INTERFACE_MODE"=43, "REG_TXRXBUFF_BOTH"=44, "REG_TXRXBUFF"=45, "REG_IRQ_RAWSTATUS1"=46, "REG_IRQ_ENABLE1"=47, "REG_IRQ_ENABLESET1"=48, "REG_IRQ_ENABLECLEAR1"=49, "REG_IRQ_RAWSTATUS2"=50, "REG_IRQ_ENABLE2"=51, "REG_IRQ_ENABLESET2"=52, "REG_IRQ_ENABLECLEAR2"=53, "REG_IRQ_STATUS1"=54, "REG_IRQ_STATUS2"=55, "REG_IRQ_AUXSTATUS"=56, "REG_TXBUFF_OVERFLOW"=57, "REG_PO0"=58, "REG_P01"=59, "REG_P02"=60, "REG_P03"=61, "REG_GP0"=62, "REG_GPI"=63, "REG_WAKEUP_245IN"=64, "REG_WAKEUP_COMPANYID"=65, "REG_WAKEUP_IMDTRANSID1"=66, "REG_WAKEUP_IMDTRANSID2"=67, "REG_WAKEUP_IMDTRANSID3"=68, "REG_WAKEUP_CHANNEL"=69, "REG_WAKEUP_MODUSER"=70, "REG_WAKEUP_DEVICEMODE"=71, "REG_WAKEUP_WK_RX_CTRL1"=72, "REG_WAKEUP_STACK_ADDR"=73, "REG_WAKEUP_CTRL"=74, "REG_WAKEUP_STROSCRTRIM"=75, "REG_WAKEUP_BIASTRIM"=76, "REG_WAKEUP_ANT245TUNE"=77, "REG_WAKEUP_WK_RX_RTRIMDET"=78, "REG_WAKEUP_WK_RX_RTRIMDEMOD"=79, "REG_WAKEUP_WK_RX_RSSIGAIN"=80, "REG_WAKEUP_LNAFREQ1"=81, "REG_WAKEUP_STACK"=83, "REG_WAKUP_XOSU"=84, "REG_WAKUP_CNTDROPOUT"=85, "REG_WAKEUP_CRCCTRL"=86, "REG_WAKEUP_CRCWORD1"=87, "REG_WAKEUP_CRCWORD2"=88, "REG_WAKEUP_WK_RX_CTRIM"=89, "REG_WAKEUP_VDDATRIM"=90, "REG_WAKEUP_VDDDTRIM"=91, "REG_WAKEUP_TESTIOBUFEN"=92, "REG_WAKEUP_TESTIOCLAMP"=93, "CORE_RESET_ADDRESS"=94, "CHIP_RESET_ADDRESS"=95, "REG_RF_TXGENCTRL"=96, "REG_RF_TXIFCTRL"=97, "REG_RF_TXRF_SEL_CTRL"=98, "REG_RF_TXRFPWRDEFAULTSET"=99, "REG_RF_RSSITRIM"=100, "REG_RF_TXIFOSCTUNE"=101, "REG_RF_TXIFGAINIMB"=102, "REG_RF_TXIFLOCK"=103, "REG_RF_RXRFLNAGAINTRIM"=104, "REG_RF_RXBIASTR"=105, "REG_RF_RXGENCTRL"=106, "REG_RF_RXIFADCDECLEV"=107, "REG_RF_RXIFDETFILTERTUNE"=108, "REG_RF_RXIFFILTERTUNE"=109, "REG_RF_GENENABLES"=110, "REG_RF_SYNTH_CHANNEL"=111, "REG_TX_RAMP_RTRIM"=112, "REG_TX_RAMP_CTRIM"=113, "REG_RF_XO_TRIM"=114, "REG_RF_SYNTH_SET_TRIM"=115, "REG_RF_ADCCTRL"=116, "REG_RF_ADCOUTPUT"=117, "REG_RF_TXIFAMP"=118, "REG_RF_SYNTH_RTRIM"=119, "REG_RF_SYNTH_CTRIM"=120, "REG_RF_SYNTH_CT"=121, "REG_RF_TXMIXER_IOSTRIM_HIGH_IP"=122, "REG_RF_TXMIXER_IOSTRIM_HIGH_IN"=123, "REG_RF_TXMIXER_IOSTRIM_HIGH_QP"=124, "REG_RF_TXMIXER_IOSTRIM_HIGH_QN"=125, "REG_HX_WUADDR"=126, "REG_REVISION"=127, "REG_NOREG_TEST"=128, "REG_DTEST_RXBUFF"=129, "REG_RXBUFF_NEXT_BLOCK"=130, "REG_RXBUFF_FIRST_IN_PACK"=131, "REG_RXBUFF_FIRST_EMPTY"=132, "REG_MAC_BYPASS"=133, "REG_DTEST_TXBUFF"=134, "REG_TXBUFF_NEXT_BLOCK"=135, "REG_TXBUFF_FIRST_IN_PACK"=136, "REG_TXBUFF_FIRST_EMPTY"=137, "REG_DTEST_SEQ"=138, "REG_DTEST_CKCORR"=139, "REG_MAC_TOPSTATE"=140, "REG_DTEST_INTERFACE"=141, "REG_IFACE_TXRX_BYPASS"=142, "REG_MAC_TXRXWAIT"=143, "REG_MAC_TXRFRAMP"=144, "REG_MAC_TRAINWORD"=145, "REG_MAC_TRAINWORD2"=146, "REG_MAC_SETTINGS"=147, "REG_MAC_CALSELECT1"=148, "REG_MAC_CALSELECT2"=149, "REG_MAC_ANTMATCHSEL"=150, "REG_MAC_ANTTUNESEL1"=151, "REG_MAC_ANTTUNESEL2"=152, "REG_MAC_ANTTUNESEL3"=153, "REG_MAC_ANTTUNESTEP"=154, "REG_MAC_WUMODEBURST"=156, "REG_MAC_WUOFFSHORT"=157, "REG_MAC_WUOFFLONG"=158, "REG_MAC_CLKRECCTRL"=159, "REG_HK_MODE_P2"=162, "REG_MAC_ANTTUNERES1"=164, "REG_MAC_ANTTUNERES2"=165, "REG_INTERFACE_MODE_TEST"=171, "REG_TXRXBUFF_BOTH_P2"=172, "REG_TXRXBUFF_P2"=173, "REG_IRQ_RAWSTATUS1_P2"=174, "REG_MAC_TXIFSTATUS1"=176, "REG_MAC_TXIFSTATUS2"=177, "REG_IRQ_RAWSTATUS2_P2"=178, "REG_MAC_TXIFRAMPDELAY"=179, "REG_MAC_TXIFRAMPSLOPE"=180, "REG_MAX_TXIFRAMP"=181, "REG_IRQ_STATUS1_P2"=182, "REG_IRQ_STATUS2_P2"=183, "REG_IRQ_AUXSTATUS_P2"=184, "REG_MAC_UNLOCK"=188, "REG_MAC_TXIFFREQ"=190, "REG_WAKEUP_TESTCTRL1"=192, "REG_WAKEUP_RX_EN_CNT"=193, "REG_WAKEUP_TESTENABLES"=194, "REG_WAKEUP_DTBI_CTRL"=195, "REG_WAKEUP_DTBO_CTRL"=196, "REG_WAKEUP_TESTIOBUFTEST"=197, "REG_WAKEUP_WK_RX_TESTCTRL1"=198, "REG_WAKEUP_WK_RX_TESTCTRL2"=199, "REG_WAKEUP_SENS_SEQUENCE_CTRL"=200, "REG_WAKEUP_LNABIAS"=201, "REG_WAKEUP_DET_TH_TRIM1"=202, "REG_WAKEUP_LNABIAS_NOM1"=203, "REG_WAKEUP_RX_TSHORT_TRIM1"=204, "REG_WAKEUP_LNABIAS_NOM2"=205, "REG_WAKEUP_RX_TLONG_TRIM1"=206, "REG_WAKEUP_LNA_NEGRTRIM_NOM1"=207, "REG_WAKEUP_RX_TBURST_TRIM1"=208, "REG_WAKEUP_RX_LNA_NEGRTRIM_NOM2"=209, "REG_WAKEUP_RX_BB_G_BW_SEL1"=210, "REG_WAKEUP_WK_RX_DET_IOSTRIM1"=212, "REG_WAKEUP_WK_RX_CTRL2"=214, "REG_WAKEUP_WK_RX_RSSIVOSTRIM"=215, "REG_WAKEUP_LNANEGR_EFF"=216, "REG_WAKEUP_XOSU_FAST"=217, "REG_WAKEUP_STROSCPWIDTH1"=218, "REG_WAKEUP_STROSCPERIOD1"=220, "REG_WAKEUP_STROSCPERIOD2"=221, "REG_WAKEUP_WK_RX_LNA_NEGRTRIM1"=222, "REG_RF_TXTESTENABLE"=224, "REG_RF_TXIFTESTMODE"=225, "REG_RF_RXTESTENABLE"=226, "REG_RF_RXIFTESTCTRL1"=227, "REG_RF_RXIFTESTCTRL2"=228, "REG_RF_RXIFTESTCTRL3"=229, "REG_RF_SYNTH_TESTCTRL1"=230, "REG_RF_SYNTH_TESTCTRL2"=231, "REG_RF_SYNTH_TESTCTRL3"=232, "REG_RF_ADCTEST1"=237, "REG_RF_ADCTEST2"=238, "REG_RF_TXMIXER_IOSTRIM_LOW_IP"=240, "REG_RF_TXMIXER_IOSTRIM_LOW_IN"=241, "REG_RF_TXMIXER_ISOTRIM_LOW_QP"=242, "REG_RF_TXMIXER_IOSTRIM_LOW_QN"=243, "REG_RF_SYNTH_KPD"=244, "REG_RF_SYNTH_LOLEV"=245, "REG_RF_TXRFPWRTUNEANTSET"=246, "REG_RF_TXPD_GAIN_CTRL"=247, "REG_RF_SYNTH_STARTUP"=248, "REG_RF_TXRFANTTUNE_TXMODE"=249, "REG_RF_TXRFANTTUNE_RXMODE"=250, "REG_RF_RXRFANTTUNE_TXMODE"=251, "REG_RF_RXRFANTTUNE_RXMODE"=252, "REG_ANTMATCH1"=253, "REG_ANTMATCH2"=254, "REG_REVISION_P2"=255] ("Register")
  w19 = TRUE
  w38 = u16 74 items=["---MANUAL ENTRY---"=1000, "REG_NOREG"=0, "REG_RXBUFF_USED"=1, "REG_RXBUFF_BSIZE"=2, "REG_TXBUFF_USED"=3, "REG_TXBUFF_BSIZE"=4, "REG_TXBUFF_MAXPACKSIZE"=5, "REG_MAC_ERRCLR"=6, "REG_MAC_TRAINNUM"=7, "REG_MAC_SYNCMATCH"=8, "REG_MAC_SYNC1"=9, "REG_MAC_SYNC2"=10, "REG_MAC_SYNC3"=11, "REG_MAC_SYNC4"=12, "REG_MAC_SYNC5"=13, "REG_MAC_MAXBERR"=14, "REG_MAC_ECCORR"=15, "REG_MAC_CRCERR"=16, "REG_MAC_BLKCNT1"=17, "REG_MAC_BLKCNT2"=18, "REG_MAC_IMDTRANSID1"=19, "REG_MAC_IMDTRANSID2"=20, "REG_MAC_IMDTRANSID3"=21, "REG_MAC_COMPANYID"=22, "REG_MAC_MODUSER"=23, "REG_MAC_CHANNEL"=25, "REG_MAC_CLEARWDOG"=26, "REG_MAC_CKCORRTHRESH"=27, "REG_HK_TXADDR"=28, "REG_HK_TXDATA"=29, "REG_HK_TXREPLY"=30, "REG_HK_USERDATA"=31, "REG_HK_USERSTATUS"=32, "REG_HK_LASTADDRESS"=33, "REG_HK_MODE"=34, "REG_MAC_STATUSSEQ"=35, "REG_MAC_MAXRETRIES"=36, "REG_MAC_RESENDTIME"=37, "REG_MAC_POWERSAVETIME"=38, "REG_MAC_HEAD_DET"=39, "REG_MAC_CTRL"=41, "REG_MAC_INITCOM"=42, "REG_INTERFACE_MODE"=43, "REG_TXRXBUFF_BOTH"=44, "REG_TXRXBUFF"=45, "REG_IRQ_RAWSTATUS1"=46, "REG_IRQ_ENABLE1"=47, "REG_IRQ_ENABLESET1"=48, "REG_IRQ_ENABLECLEAR1"=49, "REG_IRQ_RAWSTATUS2"=50, "REG_IRQ_ENABLE2"=51, "REG_IRQ_ENABLESET2"=52, "REG_IRQ_ENABLECLEAR2"=53, "REG_IRQ_STATUS1"=54, "REG_IRQ_STATUS2"=55, "REG_IRQ_AUXSTATUS"=56, "REG_TXBUFF_OVERFLOW"=57, "REG_PO0"=58, "REG_P01"=59, "REG_P02"=60, "REG_P03"=61, "REG_GP0"=62, "REG_GPI"=63, "REG_WAKEUP_245IN"=64, "REG_WAKEUP_COMPANYID"=65, "REG_WAKEUP_IMDTRANSID1"=66, "REG_WAKEUP_IMDTRANSID2"=67, "REG_WAKEUP_IMDTRANSID3"=68, "REG_WAKEUP_CHANNEL"=69, "REG_WAKEUP_MODUSER"=70, "REG_WAKEUP_DEVICEMODE"=71, "REG_WAKEUP_WK_RX_CTRL1"=72, "REG_WAKEUP_STACK_ADDR"=73, "REG_WAKEUP_CTRL"=74, "REG_WAKEUP_STROSCRTRIM"=75, "REG_WAKEUP_BIASTRIM"=76, "REG_WAKEUP_ANT245TUNE"=77, "REG_WAKEUP_WK_RX_RTRIMDET"=78, "REG_WAKEUP_WK_RX_RTRIMDEMOD"=79, "REG_WAKEUP_WK_RX_RSSIGAIN"=80, "REG_WAKEUP_LNAFREQ1"=81, "REG_WAKEUP_STACK"=83, "REG_WAKUP_XOSU"=84, "REG_WAKUP_CNTDROPOUT"=85, "REG_WAKEUP_CRCCTRL"=86, "REG_WAKEUP_CRCWORD1"=87, "REG_WAKEUP_CRCWORD2"=88, "REG_WAKEUP_WK_RX_CTRIM"=89, "REG_WAKEUP_VDDATRIM"=90, "REG_WAKEUP_VDDDTRIM"=91, "REG_WAKEUP_TESTIOBUFEN"=92, "REG_WAKEUP_TESTIOCLAMP"=93, "CORE_RESET_ADDRESS"=94, "CHIP_RESET_ADDRESS"=95, "REG_RF_TXGENCTRL"=96, "REG_RF_TXIFCTRL"=97, "REG_RF_TXRF_SEL_CTRL"=98, "REG_RF_TXRFPWRDEFAULTSET"=99, "REG_RF_RSSITRIM"=100, "REG_RF_TXIFOSCTUNE"=101, "REG_RF_TXIFGAINIMB"=102, "REG_RF_TXIFLOCK"=103, "REG_RF_RXRFLNAGAINTRIM"=104, "REG_RF_RXBIASTR"=105, "REG_RF_RXGENCTRL"=106, "REG_RF_RXIFADCDECLEV"=107, "REG_RF_RXIFDETFILTERTUNE"=108, "REG_RF_RXIFFILTERTUNE"=109, "REG_RF_GENENABLES"=110, "REG_RF_SYNTH_CHANNEL"=111, "REG_TX_RAMP_RTRIM"=112, "REG_TX_RAMP_CTRIM"=113, "REG_RF_XO_TRIM"=114, "REG_RF_SYNTH_SET_TRIM"=115, "REG_RF_ADCCTRL"=116, "REG_RF_ADCOUTPUT"=117, "REG_RF_TXIFAMP"=118, "REG_RF_SYNTH_RTRIM"=119, "REG_RF_SYNTH_CTRIM"=120, "REG_RF_SYNTH_CT"=121, "REG_RF_TXMIXER_IOSTRIM_HIGH_IP"=122, "REG_RF_TXMIXER_IOSTRIM_HIGH_IN"=123, "REG_RF_TXMIXER_IOSTRIM_HIGH_QP"=124, "REG_RF_TXMIXER_IOSTRIM_HIGH_QN"=125, "REG_HX_WUADDR"=126, "REG_REVISION"=127, "REG_NOREG_TEST"=128, "REG_DTEST_RXBUFF"=129, "REG_RXBUFF_NEXT_BLOCK"=130, "REG_RXBUFF_FIRST_IN_PACK"=131, "REG_RXBUFF_FIRST_EMPTY"=132, "REG_MAC_BYPASS"=133, "REG_DTEST_TXBUFF"=134, "REG_TXBUFF_NEXT_BLOCK"=135, "REG_TXBUFF_FIRST_IN_PACK"=136, "REG_TXBUFF_FIRST_EMPTY"=137, "REG_DTEST_SEQ"=138, "REG_DTEST_CKCORR"=139, "REG_MAC_TOPSTATE"=140, "REG_DTEST_INTERFACE"=141, "REG_IFACE_TXRX_BYPASS"=142, "REG_MAC_TXRXWAIT"=143, "REG_MAC_TXRFRAMP"=144, "REG_MAC_TRAINWORD"=145, "REG_MAC_TRAINWORD2"=146, "REG_MAC_SETTINGS"=147, "REG_MAC_CALSELECT1"=148, "REG_MAC_CALSELECT2"=149, "REG_MAC_ANTMATCHSEL"=150, "REG_MAC_ANTTUNESEL1"=151, "REG_MAC_ANTTUNESEL2"=152, "REG_MAC_ANTTUNESEL3"=153, "REG_MAC_ANTTUNESTEP"=154, "REG_MAC_WUMODEBURST"=156, "REG_MAC_WUOFFSHORT"=157, "REG_MAC_WUOFFLONG"=158, "REG_MAC_CLKRECCTRL"=159, "REG_HK_MODE_P2"=162, "REG_MAC_ANTTUNERES1"=164, "REG_MAC_ANTTUNERES2"=165, "REG_INTERFACE_MODE_TEST"=171, "REG_TXRXBUFF_BOTH_P2"=172, "REG_TXRXBUFF_P2"=173, "REG_IRQ_RAWSTATUS1_P2"=174, "REG_MAC_TXIFSTATUS1"=176, "REG_MAC_TXIFSTATUS2"=177, "REG_IRQ_RAWSTATUS2_P2"=178, "REG_MAC_TXIFRAMPDELAY"=179, "REG_MAC_TXIFRAMPSLOPE"=180, "REG_MAX_TXIFRAMP"=181, "REG_IRQ_STATUS1_P2"=182, "REG_IRQ_STATUS2_P2"=183, "REG_IRQ_AUXSTATUS_P2"=184, "REG_MAC_UNLOCK"=188, "REG_MAC_TXIFFREQ"=190, "REG_WAKEUP_TESTCTRL1"=192, "REG_WAKEUP_RX_EN_CNT"=193, "REG_WAKEUP_TESTENABLES"=194, "REG_WAKEUP_DTBI_CTRL"=195, "REG_WAKEUP_DTBO_CTRL"=196, "REG_WAKEUP_TESTIOBUFTEST"=197, "REG_WAKEUP_WK_RX_TESTCTRL1"=198, "REG_WAKEUP_WK_RX_TESTCTRL2"=199, "REG_WAKEUP_SENS_SEQUENCE_CTRL"=200, "REG_WAKEUP_LNABIAS"=201, "REG_WAKEUP_DET_TH_TRIM1"=202, "REG_WAKEUP_LNABIAS_NOM1"=203, "REG_WAKEUP_RX_TSHORT_TRIM1"=204, "REG_WAKEUP_LNABIAS_NOM2"=205, "REG_WAKEUP_RX_TLONG_TRIM1"=206, "REG_WAKEUP_LNA_NEGRTRIM_NOM1"=207, "REG_WAKEUP_RX_TBURST_TRIM1"=208, "REG_WAKEUP_RX_LNA_NEGRTRIM_NOM2"=209, "REG_WAKEUP_RX_BB_G_BW_SEL1"=210, "REG_WAKEUP_WK_RX_DET_IOSTRIM1"=212, "REG_WAKEUP_WK_RX_CTRL2"=214, "REG_WAKEUP_WK_RX_RSSIVOSTRIM"=215, "REG_WAKEUP_LNANEGR_EFF"=216, "REG_WAKEUP_XOSU_FAST"=217, "REG_WAKEUP_STROSCPWIDTH1"=218, "REG_WAKEUP_STROSCPERIOD1"=220, "REG_WAKEUP_STROSCPERIOD2"=221, "REG_WAKEUP_WK_RX_LNA_NEGRTRIM1"=222, "REG_RF_TXTESTENABLE"=224, "REG_RF_TXIFTESTMODE"=225, "REG_RF_RXTESTENABLE"=226, "REG_RF_RXIFTESTCTRL1"=227, "REG_RF_RXIFTESTCTRL2"=228, "REG_RF_RXIFTESTCTRL3"=229, "REG_RF_SYNTH_TESTCTRL1"=230, "REG_RF_SYNTH_TESTCTRL2"=231, "REG_RF_SYNTH_TESTCTRL3"=232, "REG_RF_ADCTEST1"=237, "REG_RF_ADCTEST2"=238, "REG_RF_TXMIXER_IOSTRIM_LOW_IP"=240, "REG_RF_TXMIXER_IOSTRIM_LOW_IN"=241, "REG_RF_TXMIXER_ISOTRIM_LOW_QP"=242, "REG_RF_TXMIXER_IOSTRIM_LOW_QN"=243, "REG_RF_SYNTH_KPD"=244, "REG_RF_SYNTH_LOLEV"=245, "REG_RF_TXRFPWRTUNEANTSET"=246, "REG_RF_TXPD_GAIN_CTRL"=247, "REG_RF_SYNTH_STARTUP"=248, "REG_RF_TXRFANTTUNE_TXMODE"=249, "REG_RF_TXRFANTTUNE_RXMODE"=250, "REG_RF_RXRFANTTUNE_TXMODE"=251, "REG_RF_RXRFANTTUNE_RXMODE"=252, "REG_ANTMATCH1"=253, "REG_ANTMATCH2"=254, "REG_REVISION_P2"=255] ("Register")
  w47 = u16 72 items=["---MANUAL ENTRY---"=1000, "REG_NOREG"=0, "REG_RXBUFF_USED"=1, "REG_RXBUFF_BSIZE"=2, "REG_TXBUFF_USED"=3, "REG_TXBUFF_BSIZE"=4, "REG_TXBUFF_MAXPACKSIZE"=5, "REG_MAC_ERRCLR"=6, "REG_MAC_TRAINNUM"=7, "REG_MAC_SYNCMATCH"=8, "REG_MAC_SYNC1"=9, "REG_MAC_SYNC2"=10, "REG_MAC_SYNC3"=11, "REG_MAC_SYNC4"=12, "REG_MAC_SYNC5"=13, "REG_MAC_MAXBERR"=14, "REG_MAC_ECCORR"=15, "REG_MAC_CRCERR"=16, "REG_MAC_BLKCNT1"=17, "REG_MAC_BLKCNT2"=18, "REG_MAC_IMDTRANSID1"=19, "REG_MAC_IMDTRANSID2"=20, "REG_MAC_IMDTRANSID3"=21, "REG_MAC_COMPANYID"=22, "REG_MAC_MODUSER"=23, "REG_MAC_CHANNEL"=25, "REG_MAC_CLEARWDOG"=26, "REG_MAC_CKCORRTHRESH"=27, "REG_HK_TXADDR"=28, "REG_HK_TXDATA"=29, "REG_HK_TXREPLY"=30, "REG_HK_USERDATA"=31, "REG_HK_USERSTATUS"=32, "REG_HK_LASTADDRESS"=33, "REG_HK_MODE"=34, "REG_MAC_STATUSSEQ"=35, "REG_MAC_MAXRETRIES"=36, "REG_MAC_RESENDTIME"=37, "REG_MAC_POWERSAVETIME"=38, "REG_MAC_HEAD_DET"=39, "REG_MAC_CTRL"=41, "REG_MAC_INITCOM"=42, "REG_INTERFACE_MODE"=43, "REG_TXRXBUFF_BOTH"=44, "REG_TXRXBUFF"=45, "REG_IRQ_RAWSTATUS1"=46, "REG_IRQ_ENABLE1"=47, "REG_IRQ_ENABLESET1"=48, "REG_IRQ_ENABLECLEAR1"=49, "REG_IRQ_RAWSTATUS2"=50, "REG_IRQ_ENABLE2"=51, "REG_IRQ_ENABLESET2"=52, "REG_IRQ_ENABLECLEAR2"=53, "REG_IRQ_STATUS1"=54, "REG_IRQ_STATUS2"=55, "REG_IRQ_AUXSTATUS"=56, "REG_TXBUFF_OVERFLOW"=57, "REG_PO0"=58, "REG_P01"=59, "REG_P02"=60, "REG_P03"=61, "REG_GP0"=62, "REG_GPI"=63, "REG_WAKEUP_245IN"=64, "REG_WAKEUP_COMPANYID"=65, "REG_WAKEUP_IMDTRANSID1"=66, "REG_WAKEUP_IMDTRANSID2"=67, "REG_WAKEUP_IMDTRANSID3"=68, "REG_WAKEUP_CHANNEL"=69, "REG_WAKEUP_MODUSER"=70, "REG_WAKEUP_DEVICEMODE"=71, "REG_WAKEUP_WK_RX_CTRL1"=72, "REG_WAKEUP_STACK_ADDR"=73, "REG_WAKEUP_CTRL"=74, "REG_WAKEUP_STROSCRTRIM"=75, "REG_WAKEUP_BIASTRIM"=76, "REG_WAKEUP_ANT245TUNE"=77, "REG_WAKEUP_WK_RX_RTRIMDET"=78, "REG_WAKEUP_WK_RX_RTRIMDEMOD"=79, "REG_WAKEUP_WK_RX_RSSIGAIN"=80, "REG_WAKEUP_LNAFREQ1"=81, "REG_WAKEUP_STACK"=83, "REG_WAKUP_XOSU"=84, "REG_WAKUP_CNTDROPOUT"=85, "REG_WAKEUP_CRCCTRL"=86, "REG_WAKEUP_CRCWORD1"=87, "REG_WAKEUP_CRCWORD2"=88, "REG_WAKEUP_WK_RX_CTRIM"=89, "REG_WAKEUP_VDDATRIM"=90, "REG_WAKEUP_VDDDTRIM"=91, "REG_WAKEUP_TESTIOBUFEN"=92, "REG_WAKEUP_TESTIOCLAMP"=93, "CORE_RESET_ADDRESS"=94, "CHIP_RESET_ADDRESS"=95, "REG_RF_TXGENCTRL"=96, "REG_RF_TXIFCTRL"=97, "REG_RF_TXRF_SEL_CTRL"=98, "REG_RF_TXRFPWRDEFAULTSET"=99, "REG_RF_RSSITRIM"=100, "REG_RF_TXIFOSCTUNE"=101, "REG_RF_TXIFGAINIMB"=102, "REG_RF_TXIFLOCK"=103, "REG_RF_RXRFLNAGAINTRIM"=104, "REG_RF_RXBIASTR"=105, "REG_RF_RXGENCTRL"=106, "REG_RF_RXIFADCDECLEV"=107, "REG_RF_RXIFDETFILTERTUNE"=108, "REG_RF_RXIFFILTERTUNE"=109, "REG_RF_GENENABLES"=110, "REG_RF_SYNTH_CHANNEL"=111, "REG_TX_RAMP_RTRIM"=112, "REG_TX_RAMP_CTRIM"=113, "REG_RF_XO_TRIM"=114, "REG_RF_SYNTH_SET_TRIM"=115, "REG_RF_ADCCTRL"=116, "REG_RF_ADCOUTPUT"=117, "REG_RF_TXIFAMP"=118, "REG_RF_SYNTH_RTRIM"=119, "REG_RF_SYNTH_CTRIM"=120, "REG_RF_SYNTH_CT"=121, "REG_RF_TXMIXER_IOSTRIM_HIGH_IP"=122, "REG_RF_TXMIXER_IOSTRIM_HIGH_IN"=123, "REG_RF_TXMIXER_IOSTRIM_HIGH_QP"=124, "REG_RF_TXMIXER_IOSTRIM_HIGH_QN"=125, "REG_HX_WUADDR"=126, "REG_REVISION"=127, "REG_NOREG_TEST"=128, "REG_DTEST_RXBUFF"=129, "REG_RXBUFF_NEXT_BLOCK"=130, "REG_RXBUFF_FIRST_IN_PACK"=131, "REG_RXBUFF_FIRST_EMPTY"=132, "REG_MAC_BYPASS"=133, "REG_DTEST_TXBUFF"=134, "REG_TXBUFF_NEXT_BLOCK"=135, "REG_TXBUFF_FIRST_IN_PACK"=136, "REG_TXBUFF_FIRST_EMPTY"=137, "REG_DTEST_SEQ"=138, "REG_DTEST_CKCORR"=139, "REG_MAC_TOPSTATE"=140, "REG_DTEST_INTERFACE"=141, "REG_IFACE_TXRX_BYPASS"=142, "REG_MAC_TXRXWAIT"=143, "REG_MAC_TXRFRAMP"=144, "REG_MAC_TRAINWORD"=145, "REG_MAC_TRAINWORD2"=146, "REG_MAC_SETTINGS"=147, "REG_MAC_CALSELECT1"=148, "REG_MAC_CALSELECT2"=149, "REG_MAC_ANTMATCHSEL"=150, "REG_MAC_ANTTUNESEL1"=151, "REG_MAC_ANTTUNESEL2"=152, "REG_MAC_ANTTUNESEL3"=153, "REG_MAC_ANTTUNESTEP"=154, "REG_MAC_WUMODEBURST"=156, "REG_MAC_WUOFFSHORT"=157, "REG_MAC_WUOFFLONG"=158, "REG_MAC_CLKRECCTRL"=159, "REG_HK_MODE_P2"=162, "REG_MAC_ANTTUNERES1"=164, "REG_MAC_ANTTUNERES2"=165, "REG_INTERFACE_MODE_TEST"=171, "REG_TXRXBUFF_BOTH_P2"=172, "REG_TXRXBUFF_P2"=173, "REG_IRQ_RAWSTATUS1_P2"=174, "REG_MAC_TXIFSTATUS1"=176, "REG_MAC_TXIFSTATUS2"=177, "REG_IRQ_RAWSTATUS2_P2"=178, "REG_MAC_TXIFRAMPDELAY"=179, "REG_MAC_TXIFRAMPSLOPE"=180, "REG_MAX_TXIFRAMP"=181, "REG_IRQ_STATUS1_P2"=182, "REG_IRQ_STATUS2_P2"=183, "REG_IRQ_AUXSTATUS_P2"=184, "REG_MAC_UNLOCK"=188, "REG_MAC_TXIFFREQ"=190, "REG_WAKEUP_TESTCTRL1"=192, "REG_WAKEUP_RX_EN_CNT"=193, "REG_WAKEUP_TESTENABLES"=194, "REG_WAKEUP_DTBI_CTRL"=195, "REG_WAKEUP_DTBO_CTRL"=196, "REG_WAKEUP_TESTIOBUFTEST"=197, "REG_WAKEUP_WK_RX_TESTCTRL1"=198, "REG_WAKEUP_WK_RX_TESTCTRL2"=199, "REG_WAKEUP_SENS_SEQUENCE_CTRL"=200, "REG_WAKEUP_LNABIAS"=201, "REG_WAKEUP_DET_TH_TRIM1"=202, "REG_WAKEUP_LNABIAS_NOM1"=203, "REG_WAKEUP_RX_TSHORT_TRIM1"=204, "REG_WAKEUP_LNABIAS_NOM2"=205, "REG_WAKEUP_RX_TLONG_TRIM1"=206, "REG_WAKEUP_LNA_NEGRTRIM_NOM1"=207, "REG_WAKEUP_RX_TBURST_TRIM1"=208, "REG_WAKEUP_RX_LNA_NEGRTRIM_NOM2"=209, "REG_WAKEUP_RX_BB_G_BW_SEL1"=210, "REG_WAKEUP_WK_RX_DET_IOSTRIM1"=212, "REG_WAKEUP_WK_RX_CTRL2"=214, "REG_WAKEUP_WK_RX_RSSIVOSTRIM"=215, "REG_WAKEUP_LNANEGR_EFF"=216, "REG_WAKEUP_XOSU_FAST"=217, "REG_WAKEUP_STROSCPWIDTH1"=218, "REG_WAKEUP_STROSCPERIOD1"=220, "REG_WAKEUP_STROSCPERIOD2"=221, "REG_WAKEUP_WK_RX_LNA_NEGRTRIM1"=222, "REG_RF_TXTESTENABLE"=224, "REG_RF_TXIFTESTMODE"=225, "REG_RF_RXTESTENABLE"=226, "REG_RF_RXIFTESTCTRL1"=227, "REG_RF_RXIFTESTCTRL2"=228, "REG_RF_RXIFTESTCTRL3"=229, "REG_RF_SYNTH_TESTCTRL1"=230, "REG_RF_SYNTH_TESTCTRL2"=231, "REG_RF_SYNTH_TESTCTRL3"=232, "REG_RF_ADCTEST1"=237, "REG_RF_ADCTEST2"=238, "REG_RF_TXMIXER_IOSTRIM_LOW_IP"=240, "REG_RF_TXMIXER_IOSTRIM_LOW_IN"=241, "REG_RF_TXMIXER_ISOTRIM_LOW_QP"=242, "REG_RF_TXMIXER_IOSTRIM_LOW_QN"=243, "REG_RF_SYNTH_KPD"=244, "REG_RF_SYNTH_LOLEV"=245, "REG_RF_TXRFPWRTUNEANTSET"=246, "REG_RF_TXPD_GAIN_CTRL"=247, "REG_RF_SYNTH_STARTUP"=248, "REG_RF_TXRFANTTUNE_TXMODE"=249, "REG_RF_TXRFANTTUNE_RXMODE"=250, "REG_RF_RXRFANTTUNE_TXMODE"=251, "REG_RF_RXRFANTTUNE_RXMODE"=252, "REG_ANTMATCH1"=253, "REG_ANTMATCH2"=254, "REG_REVISION_P2"=255] ("Register")
  w48 = u16 198 items=["---MANUAL ENTRY---"=1000, "REG_NOREG"=0, "REG_RXBUFF_USED"=1, "REG_RXBUFF_BSIZE"=2, "REG_TXBUFF_USED"=3, "REG_TXBUFF_BSIZE"=4, "REG_TXBUFF_MAXPACKSIZE"=5, "REG_MAC_ERRCLR"=6, "REG_MAC_TRAINNUM"=7, "REG_MAC_SYNCMATCH"=8, "REG_MAC_SYNC1"=9, "REG_MAC_SYNC2"=10, "REG_MAC_SYNC3"=11, "REG_MAC_SYNC4"=12, "REG_MAC_SYNC5"=13, "REG_MAC_MAXBERR"=14, "REG_MAC_ECCORR"=15, "REG_MAC_CRCERR"=16, "REG_MAC_BLKCNT1"=17, "REG_MAC_BLKCNT2"=18, "REG_MAC_IMDTRANSID1"=19, "REG_MAC_IMDTRANSID2"=20, "REG_MAC_IMDTRANSID3"=21, "REG_MAC_COMPANYID"=22, "REG_MAC_MODUSER"=23, "REG_MAC_CHANNEL"=25, "REG_MAC_CLEARWDOG"=26, "REG_MAC_CKCORRTHRESH"=27, "REG_HK_TXADDR"=28, "REG_HK_TXDATA"=29, "REG_HK_TXREPLY"=30, "REG_HK_USERDATA"=31, "REG_HK_USERSTATUS"=32, "REG_HK_LASTADDRESS"=33, "REG_HK_MODE"=34, "REG_MAC_STATUSSEQ"=35, "REG_MAC_MAXRETRIES"=36, "REG_MAC_RESENDTIME"=37, "REG_MAC_POWERSAVETIME"=38, "REG_MAC_HEAD_DET"=39, "REG_MAC_CTRL"=41, "REG_MAC_INITCOM"=42, "REG_INTERFACE_MODE"=43, "REG_TXRXBUFF_BOTH"=44, "REG_TXRXBUFF"=45, "REG_IRQ_RAWSTATUS1"=46, "REG_IRQ_ENABLE1"=47, "REG_IRQ_ENABLESET1"=48, "REG_IRQ_ENABLECLEAR1"=49, "REG_IRQ_RAWSTATUS2"=50, "REG_IRQ_ENABLE2"=51, "REG_IRQ_ENABLESET2"=52, "REG_IRQ_ENABLECLEAR2"=53, "REG_IRQ_STATUS1"=54, "REG_IRQ_STATUS2"=55, "REG_IRQ_AUXSTATUS"=56, "REG_TXBUFF_OVERFLOW"=57, "REG_PO0"=58, "REG_P01"=59, "REG_P02"=60, "REG_P03"=61, "REG_GP0"=62, "REG_GPI"=63, "REG_WAKEUP_245IN"=64, "REG_WAKEUP_COMPANYID"=65, "REG_WAKEUP_IMDTRANSID1"=66, "REG_WAKEUP_IMDTRANSID2"=67, "REG_WAKEUP_IMDTRANSID3"=68, "REG_WAKEUP_CHANNEL"=69, "REG_WAKEUP_MODUSER"=70, "REG_WAKEUP_DEVICEMODE"=71, "REG_WAKEUP_WK_RX_CTRL1"=72, "REG_WAKEUP_STACK_ADDR"=73, "REG_WAKEUP_CTRL"=74, "REG_WAKEUP_STROSCRTRIM"=75, "REG_WAKEUP_BIASTRIM"=76, "REG_WAKEUP_ANT245TUNE"=77, "REG_WAKEUP_WK_RX_RTRIMDET"=78, "REG_WAKEUP_WK_RX_RTRIMDEMOD"=79, "REG_WAKEUP_WK_RX_RSSIGAIN"=80, "REG_WAKEUP_LNAFREQ1"=81, "REG_WAKEUP_STACK"=83, "REG_WAKUP_XOSU"=84, "REG_WAKUP_CNTDROPOUT"=85, "REG_WAKEUP_CRCCTRL"=86, "REG_WAKEUP_CRCWORD1"=87, "REG_WAKEUP_CRCWORD2"=88, "REG_WAKEUP_WK_RX_CTRIM"=89, "REG_WAKEUP_VDDATRIM"=90, "REG_WAKEUP_VDDDTRIM"=91, "REG_WAKEUP_TESTIOBUFEN"=92, "REG_WAKEUP_TESTIOCLAMP"=93, "CORE_RESET_ADDRESS"=94, "CHIP_RESET_ADDRESS"=95, "REG_RF_TXGENCTRL"=96, "REG_RF_TXIFCTRL"=97, "REG_RF_TXRF_SEL_CTRL"=98, "REG_RF_TXRFPWRDEFAULTSET"=99, "REG_RF_RSSITRIM"=100, "REG_RF_TXIFOSCTUNE"=101, "REG_RF_TXIFGAINIMB"=102, "REG_RF_TXIFLOCK"=103, "REG_RF_RXRFLNAGAINTRIM"=104, "REG_RF_RXBIASTR"=105, "REG_RF_RXGENCTRL"=106, "REG_RF_RXIFADCDECLEV"=107, "REG_RF_RXIFDETFILTERTUNE"=108, "REG_RF_RXIFFILTERTUNE"=109, "REG_RF_GENENABLES"=110, "REG_RF_SYNTH_CHANNEL"=111, "REG_TX_RAMP_RTRIM"=112, "REG_TX_RAMP_CTRIM"=113, "REG_RF_XO_TRIM"=114, "REG_RF_SYNTH_SET_TRIM"=115, "REG_RF_ADCCTRL"=116, "REG_RF_ADCOUTPUT"=117, "REG_RF_TXIFAMP"=118, "REG_RF_SYNTH_RTRIM"=119, "REG_RF_SYNTH_CTRIM"=120, "REG_RF_SYNTH_CT"=121, "REG_RF_TXMIXER_IOSTRIM_HIGH_IP"=122, "REG_RF_TXMIXER_IOSTRIM_HIGH_IN"=123, "REG_RF_TXMIXER_IOSTRIM_HIGH_QP"=124, "REG_RF_TXMIXER_IOSTRIM_HIGH_QN"=125, "REG_HX_WUADDR"=126, "REG_REVISION"=127, "REG_NOREG_TEST"=128, "REG_DTEST_RXBUFF"=129, "REG_RXBUFF_NEXT_BLOCK"=130, "REG_RXBUFF_FIRST_IN_PACK"=131, "REG_RXBUFF_FIRST_EMPTY"=132, "REG_MAC_BYPASS"=133, "REG_DTEST_TXBUFF"=134, "REG_TXBUFF_NEXT_BLOCK"=135, "REG_TXBUFF_FIRST_IN_PACK"=136, "REG_TXBUFF_FIRST_EMPTY"=137, "REG_DTEST_SEQ"=138, "REG_DTEST_CKCORR"=139, "REG_MAC_TOPSTATE"=140, "REG_DTEST_INTERFACE"=141, "REG_IFACE_TXRX_BYPASS"=142, "REG_MAC_TXRXWAIT"=143, "REG_MAC_TXRFRAMP"=144, "REG_MAC_TRAINWORD"=145, "REG_MAC_TRAINWORD2"=146, "REG_MAC_SETTINGS"=147, "REG_MAC_CALSELECT1"=148, "REG_MAC_CALSELECT2"=149, "REG_MAC_ANTMATCHSEL"=150, "REG_MAC_ANTTUNESEL1"=151, "REG_MAC_ANTTUNESEL2"=152, "REG_MAC_ANTTUNESEL3"=153, "REG_MAC_ANTTUNESTEP"=154, "REG_MAC_WUMODEBURST"=156, "REG_MAC_WUOFFSHORT"=157, "REG_MAC_WUOFFLONG"=158, "REG_MAC_CLKRECCTRL"=159, "REG_HK_MODE_P2"=162, "REG_MAC_ANTTUNERES1"=164, "REG_MAC_ANTTUNERES2"=165, "REG_INTERFACE_MODE_TEST"=171, "REG_TXRXBUFF_BOTH_P2"=172, "REG_TXRXBUFF_P2"=173, "REG_IRQ_RAWSTATUS1_P2"=174, "REG_MAC_TXIFSTATUS1"=176, "REG_MAC_TXIFSTATUS2"=177, "REG_IRQ_RAWSTATUS2_P2"=178, "REG_MAC_TXIFRAMPDELAY"=179, "REG_MAC_TXIFRAMPSLOPE"=180, "REG_MAX_TXIFRAMP"=181, "REG_IRQ_STATUS1_P2"=182, "REG_IRQ_STATUS2_P2"=183, "REG_IRQ_AUXSTATUS_P2"=184, "REG_MAC_UNLOCK"=188, "REG_MAC_TXIFFREQ"=190, "REG_WAKEUP_TESTCTRL1"=192, "REG_WAKEUP_RX_EN_CNT"=193, "REG_WAKEUP_TESTENABLES"=194, "REG_WAKEUP_DTBI_CTRL"=195, "REG_WAKEUP_DTBO_CTRL"=196, "REG_WAKEUP_TESTIOBUFTEST"=197, "REG_WAKEUP_WK_RX_TESTCTRL1"=198, "REG_WAKEUP_WK_RX_TESTCTRL2"=199, "REG_WAKEUP_SENS_SEQUENCE_CTRL"=200, "REG_WAKEUP_LNABIAS"=201, "REG_WAKEUP_DET_TH_TRIM1"=202, "REG_WAKEUP_LNABIAS_NOM1"=203, "REG_WAKEUP_RX_TSHORT_TRIM1"=204, "REG_WAKEUP_LNABIAS_NOM2"=205, "REG_WAKEUP_RX_TLONG_TRIM1"=206, "REG_WAKEUP_LNA_NEGRTRIM_NOM1"=207, "REG_WAKEUP_RX_TBURST_TRIM1"=208, "REG_WAKEUP_RX_LNA_NEGRTRIM_NOM2"=209, "REG_WAKEUP_RX_BB_G_BW_SEL1"=210, "REG_WAKEUP_WK_RX_DET_IOSTRIM1"=212, "REG_WAKEUP_WK_RX_CTRL2"=214, "REG_WAKEUP_WK_RX_RSSIVOSTRIM"=215, "REG_WAKEUP_LNANEGR_EFF"=216, "REG_WAKEUP_XOSU_FAST"=217, "REG_WAKEUP_STROSCPWIDTH1"=218, "REG_WAKEUP_STROSCPERIOD1"=220, "REG_WAKEUP_STROSCPERIOD2"=221, "REG_WAKEUP_WK_RX_LNA_NEGRTRIM1"=222, "REG_RF_TXTESTENABLE"=224, "REG_RF_TXIFTESTMODE"=225, "REG_RF_RXTESTENABLE"=226, "REG_RF_RXIFTESTCTRL1"=227, "REG_RF_RXIFTESTCTRL2"=228, "REG_RF_RXIFTESTCTRL3"=229, "REG_RF_SYNTH_TESTCTRL1"=230, "REG_RF_SYNTH_TESTCTRL2"=231, "REG_RF_SYNTH_TESTCTRL3"=232, "REG_RF_ADCTEST1"=237, "REG_RF_ADCTEST2"=238, "REG_RF_TXMIXER_IOSTRIM_LOW_IP"=240, "REG_RF_TXMIXER_IOSTRIM_LOW_IN"=241, "REG_RF_TXMIXER_ISOTRIM_LOW_QP"=242, "REG_RF_TXMIXER_IOSTRIM_LOW_QN"=243, "REG_RF_SYNTH_KPD"=244, "REG_RF_SYNTH_LOLEV"=245, "REG_RF_TXRFPWRTUNEANTSET"=246, "REG_RF_TXPD_GAIN_CTRL"=247, "REG_RF_SYNTH_STARTUP"=248, "REG_RF_TXRFANTTUNE_TXMODE"=249, "REG_RF_TXRFANTTUNE_RXMODE"=250, "REG_RF_RXRFANTTUNE_TXMODE"=251, "REG_RF_RXRFANTTUNE_RXMODE"=252, "REG_ANTMATCH1"=253, "REG_ANTMATCH2"=254, "REG_REVISION_P2"=255] ("Register")
  w36 = FALSE
  w3 = u8 0
  # "Initialize the \nregisters used\nfor testing"
  # "Disable DSC"
  # "Stop \"Wakeup toggle\""
  # "Disable Wakeup Test Registers"
  # "Enable RSSI, Wakeup LNA, Detector"
  # "Enable Wakeup Test Registers"
  n1 = flat-sequence {
    tunnel: "error in (no error)" -> [w51]
    tunnel: [w51] -> w23
    tunnel: "DetTrim" -> [w50]
    frame #0 {
      n2 = case shown="True" w50 {
        frame False {
          n3 = local write "Detector Offset Trim"(u8 32 ("Detector Theshold")) -> ()
          n4 = local write "RSSI Fine Trim"(u8 15 ("Baseband Gain")) -> ()
        }
        frame True {
        }
      }
      n5 = local write "Wakeup Signal Power, dBm"(-32.0 ("Wakeup Signal Power, dBm")) -> ()
      n6 = local write "Wakeup Signal Transmit"(FALSE ("Wakeup Signal Transmit")) -> ()
      n7 = local write "Update Radio Settings"(FALSE ("Update Radio Settings")) -> ()
      n8 = local write "Samples to Average"(u8 5 ("Samples to Average")) -> ()
      n9 = local write "LNA Frequency Trim"(u8 15 ("LNA Frequency Trim")) -> ()
      n10 = local write "Loopback Detector"(FALSE ("Loopback Detector")) -> ()
      n11 = local write "RX Antenna Tune"(u8 0 ("RX Antenna Tune")) -> ()
      n12 = local write "LNA Gain Trim"(u8 20 ("LNA Gain Trim")) -> ()
      n13 = local write "Do RSSI"(FALSE ("Do RSSI")) -> ()
    }
  }
  n14 = call "MICSD Set Register.vi"("Execute on Remote?(F)"=w19, "error in (no error)"=w23, "Data"=u8 129, "Address"=w25, "VISA Resource Name"="PRIMARY MICS Dongle Address") -> ("error out"=w18:errorcluster, "dup VISA Resource Name"=w17:refnum<visa-resource-name>)  [unwired: 5 in]
  n15 = local read "WakeupMode"() -> (w5:bool)
  n16 = call "MICSD Set Register.vi"("Execute on Remote?(F)"=w19, "error in (no error)"=w18, "Data"=u8 0, "Address"=w21, "VISA Resource Name"=w17) -> ("error out"=w15:errorcluster, "dup VISA Resource Name"=w16:refnum<visa-resource-name>)  [unwired: 5 in]
  n17 = Select(t=u8 64 ("Data"), s=w5, f=u8 73 ("Data")) -> (s? t:f=w8:u8)
  n18 = call "MICSD Get Register.vi"("Execute on Remote?(F)"=w19, "error in (no error)"=w15, "Address"=w38, "VISA Resource Name"=w16) -> ("error out"=w42:errorcluster, "Data"=w40:u8, "dup VISA Resource Name"=w44:refnum<visa-resource-name>)  [unwired: 5 in]
  n19 = Select(t=u8 1 ("Data"), s=w5, f=u8 0 ("Data")) -> (s? t:f=w4:u8)
  n20 = Or(x=w8, y=w40) -> (x .or. y?=w39:u8)
  n21 = call "MICSD Set Register.vi"("Execute on Remote?(F)"=w19, "error in (no error)"=w42, "Data"=w39, "Address"=w38, "VISA Resource Name"=w44) -> ("error out"=w41:errorcluster, "dup VISA Resource Name"=w43:refnum<visa-resource-name>)  [unwired: 5 in]
  n22 = call "MICSD Set Register.vi"("Execute on Remote?(F)"=w19, "error in (no error)"=w41, "Data"=w4, "Address"=w48, "VISA Resource Name"=w43) -> ("error out"=w45:errorcluster, "dup VISA Resource Name"=w46:refnum<visa-resource-name>)  [unwired: 5 in]
  n23 = Select(t=u8 15 ("Data"), s="DetTrim", f=u8 13 ("Data")) -> (s? t:f=w14:u8)
  n24 = call "MICSD Set Register.vi"("Execute on Remote?(F)"=w19, "error in (no error)"=w45, "Data"=w14, "Address"=w47, "VISA Resource Name"=w46) -> ("error out"=w37:errorcluster)  [unwired: 5 in, 1 out]
  n25 = while {
    shift-right: [w69] -> w28
    shift-left: w37 -> [w73]
    tunnel: "PRIMARY MICS Dongle Address" -> [w74]
    tunnel: "SECONDARY MICS Dongle Address" -> [w90]
    shift-right: [w83] -> _
    shift-left: w3 -> [w88]
    shift-right: [w82] -> _
    shift-left: w3 -> [w87]
    shift-right: [w81] -> _
    shift-left: w3 -> [w86]
    shift-right: [w80] -> _
    shift-left: w3 -> [w85]
    shift-right: [w79] -> _
    shift-left: w3 -> [w84]
    shift-right: [w78] -> _
    shift-left: 0.0 -> [w89]
    shift-right: [w75] -> _
    shift-left: w36 -> [w76]
    shift-right: [w71] -> _
    shift-left: w36 -> [w72]
    tunnel: T1 {"ConfigFlags"=0, "ImplantID"=1048576, "CompanyID"=187, "Normal_Comm"={"RF_Channel"=4, "UserData"=0, "TX_Mod"=0, "RX_Mod"=0, "RX_BlockSize"=15, "BlockPerPack"=31, "TX_BlockSize"=15}, "Emerg_Comm"={"RF_Channel"=4, "UserData"=0, "TX_Mod"=0, "RX_Mod"=0, "TX_BlockSize"=15, "BlockPerPack"=31, "RX_BlockSize"=15}, "ImplantRev"=4, "245TX_PowerCal"=0, "245TX_Power"=10, "CCA_RSSI_Thresholds"={"ch0"=2650, "ch1"=2650, "ch2"=2650, "ch3"=2650, "ch4"=2650, "ch5"=2650, "ch6"=2650, "ch7"=2650, "ch8"=2650, "ch9"=2650}} ("MICS_Config_In") -> [w70]
    tunnel: "DetTrim" -> [w65]
    shift-right: [w63] -> _
    shift-left: w3 -> [w64]
    stop <- w68 stop-if-true
    # "RSSI Gain"
    # "RF CW Change?"
    # "Radio Val Change?"
    # "Wakeup RF PWR"
    # "RSSI Fine Trim"
    # "RX Ant Tune"
    # "LNA Gain Trim"
    # "Detector Offset"
    # "LNA Freq Trim"
    n26 = Wait (ms)(milliseconds to wait=u32 15) -> ()  [unwired: 1 out]
    n27 = for {
      N: 6 -> [_]
      shift-right: [w114] -> w69
      shift-left: w73 -> [w115]
      tunnel: w90 -> [w113]
      tunnel: w74 -> [w112]
      shift-right: [w106] -> w83
      shift-left: w88 -> [w111]
      shift-right: [w105] -> w82
      shift-left: w87 -> [w110]
      shift-right: [w104] -> w81
      shift-left: w86 -> [w109]
      shift-right: [w103] -> w80
      shift-left: w85 -> [w108]
      shift-right: [w102] -> w79
      shift-left: w84 -> [w107]
      shift-right: [w100] -> w78
      shift-left: w89 -> [w101]
      tunnel: w70 -> [w95]
      shift-right: [w98] -> w75
      shift-left: w76 -> [w99]
      shift-right: [w96] -> w71
      shift-left: w72 -> [w97]
      tunnel: w65 -> [w94]
      shift-right: [w92] -> w63
      shift-left: w64 -> [w93]
      i -> [w116]
      n28 = case shown="4" w116 {
        tunnel: w115 -> [w137 w154 w260 w313 w381 w386]
        tunnel: [w137 w152 w249 w312 w381 w384] -> w114
        tunnel: w113 -> [_ _ w259 _ _ _]
        tunnel: w112 -> [_ w142 _ w310 _ w385]
        tunnel: w111 -> [w136 w151 w268 w322 w376 w391]
        tunnel: w110 -> [w134 w150 w267 w321 w373 w388]
        tunnel: w109 -> [w132 w149 w266 w320 w375 w390]
        tunnel: w108 -> [w130 w148 w265 w319 w374 w389]
        tunnel: w107 -> [w129 w147 w264 w318 w371 w387]
        tunnel: ["LNA Frequency Trim" w151 w268 w322 w376 w391] -> w106
        tunnel: ["Detector Offset Trim" w150 w267 w321 w373 w388] -> w105
        tunnel: ["LNA Gain Trim" w149 w266 w320 w375 w390] -> w104
        tunnel: ["RX Antenna Tune" w148 w265 w319 w374 w389] -> w103
        tunnel: ["RSSI Fine Trim" w147 w264 w318 w371 w387] -> w102
        tunnel: w101 -> [w119 w146 w252 w317 w378 w392]
        tunnel: [w119 w146 "Wakeup Signal Power, dBm" w317 w378 w392] -> w100
        tunnel: w99 -> [_ w144 w263 w316 w379 w393]
        tunnel: [w126 w153 w263 w316 w379 w393] -> w98
        tunnel: w97 -> [w120 w141 w262 w315 w380 w394]
        tunnel: [w120 w140 "Wakeup Signal Transmit" w315 w380 w394] -> w96
        tunnel: w95 -> [_ _ w253 _ _ _]
        tunnel: w94 -> [_ w139 _ _ _ _]
        tunnel: w93 -> [w118 w138 w248 w309 w370 w382]
        tunnel: ["RSSI Gain" w138 w248 w309 w370 w382] -> w92
        frame 0, Default {
          # "Check for Control Changes"
          n29 = Not Equal?(x=w118, y="RSSI Gain") -> ()  [unwired: 1 out]
          n30 = Not Equal?(x=w136, y="LNA Frequency Trim") -> (x != y?=w121:bool)
          n31 = Not Equal?(x=w134, y="Detector Offset Trim") -> (x != y?=w122:bool)
          n32 = Not Equal?(x=w132, y="LNA Gain Trim") -> (x != y?=w123:bool)
          n33 = Not Equal?(x=w130, y="RX Antenna Tune") -> (x != y?=w124:bool)
          n34 = Not Equal?(x=w129, y="RSSI Fine Trim") -> (x != y?=w125:bool)
          n35 = Compound Arithmetic op=OR(w121, w122, w123, w124, w125) -> (w126:bool)
        }
        frame 1 {
          # "Apply Control Changes (If Enabled)"
          n36 = And(x=w144, y="Update Radio Settings") -> (x .and. y?=w143:bool)
          n37 = case shown="True" w143 {
            tunnel: w154 -> [w156 w186]
            tunnel: w144 -> [w157 _]
            tunnel: [w157 FALSE] -> w153
            tunnel: [w156 w172] -> w152
            tunnel: w151 -> [_ w181]
            tunnel: w150 -> [_ w182]
            tunnel: w149 -> [_ w183]
            tunnel: w148 -> [_ w184]
            tunnel: w147 -> [_ w185]
            tunnel: w142 -> [_ w168]
            tunnel: w141 -> [w155 w180]
            tunnel: [w155 w180] -> w140
            tunnel: w139 -> [_ w163]
            tunnel: w138 -> [_ w158]
            frame False {
            }
            frame True {
              w167 = TRUE
              w179 = u16 86 items=["---MANUAL ENTRY---"=1000, "REG_NOREG"=0, "REG_RXBUFF_USED"=1, "REG_RXBUFF_BSIZE"=2, "REG_TXBUFF_USED"=3, "REG_TXBUFF_BSIZE"=4, "REG_TXBUFF_MAXPACKSIZE"=5, "REG_MAC_ERRCLR"=6, "REG_MAC_TRAINNUM"=7, "REG_MAC_SYNCMATCH"=8, "REG_MAC_SYNC1"=9, "REG_MAC_SYNC2"=10, "REG_MAC_SYNC3"=11, "REG_MAC_SYNC4"=12, "REG_MAC_SYNC5"=13, "REG_MAC_MAXBERR"=14, "REG_MAC_ECCORR"=15, "REG_MAC_CRCERR"=16, "REG_MAC_BLKCNT1"=17, "REG_MAC_BLKCNT2"=18, "REG_MAC_IMDTRANSID1"=19, "REG_MAC_IMDTRANSID2"=20, "REG_MAC_IMDTRANSID3"=21, "REG_MAC_COMPANYID"=22, "REG_MAC_MODUSER"=23, "REG_MAC_CHANNEL"=25, "REG_MAC_CLEARWDOG"=26, "REG_MAC_CKCORRTHRESH"=27, "REG_HK_TXADDR"=28, "REG_HK_TXDATA"=29, "REG_HK_TXREPLY"=30, "REG_HK_USERDATA"=31, "REG_HK_USERSTATUS"=32, "REG_HK_LASTADDRESS"=33, "REG_HK_MODE"=34, "REG_MAC_STATUSSEQ"=35, "REG_MAC_MAXRETRIES"=36, "REG_MAC_RESENDTIME"=37, "REG_MAC_POWERSAVETIME"=38, "REG_MAC_HEAD_DET"=39, "REG_MAC_CTRL"=41, "REG_MAC_INITCOM"=42, "REG_INTERFACE_MODE"=43, "REG_TXRXBUFF_BOTH"=44, "REG_TXRXBUFF"=45, "REG_IRQ_RAWSTATUS1"=46, "REG_IRQ_ENABLE1"=47, "REG_IRQ_ENABLESET1"=48, "REG_IRQ_ENABLECLEAR1"=49, "REG_IRQ_RAWSTATUS2"=50, "REG_IRQ_ENABLE2"=51, "REG_IRQ_ENABLESET2"=52, "REG_IRQ_ENABLECLEAR2"=53, "REG_IRQ_STATUS1"=54, "REG_IRQ_STATUS2"=55, "REG_IRQ_AUXSTATUS"=56, "REG_TXBUFF_OVERFLOW"=57, "REG_PO0"=58, "REG_P01"=59, "REG_P02"=60, "REG_P03"=61, "REG_GP0"=62, "REG_GPI"=63, "REG_WAKEUP_245IN"=64, "REG_WAKEUP_COMPANYID"=65, "REG_WAKEUP_IMDTRANSID1"=66, "REG_WAKEUP_IMDTRANSID2"=67, "REG_WAKEUP_IMDTRANSID3"=68, "REG_WAKEUP_CHANNEL"=69, "REG_WAKEUP_MODUSER"=70, "REG_WAKEUP_DEVICEMODE"=71, "REG_WAKEUP_WK_RX_CTRL1"=72, "REG_WAKEUP_STACK_ADDR"=73, "REG_WAKEUP_CTRL"=74, "REG_WAKEUP_STROSCRTRIM"=75, "REG_WAKEUP_BIASTRIM"=76, "REG_WAKEUP_ANT245TUNE"=77, "REG_WAKEUP_WK_RX_RTRIMDET"=78, "REG_WAKEUP_WK_RX_RTRIMDEMOD"=79, "REG_WAKEUP_WK_RX_RSSIGAIN"=80, "REG_WAKEUP_LNAFREQ1"=81, "REG_WAKEUP_STACK"=83, "REG_WAKUP_XOSU"=84, "REG_WAKUP_CNTDROPOUT"=85, "REG_WAKEUP_CRCCTRL"=86, "REG_WAKEUP_CRCWORD1"=87, "REG_WAKEUP_CRCWORD2"=88, "REG_WAKEUP_WK_RX_CTRIM"=89, "REG_WAKEUP_VDDATRIM"=90, "REG_WAKEUP_VDDDTRIM"=91, "REG_WAKEUP_TESTIOBUFEN"=92, "REG_WAKEUP_TESTIOCLAMP"=93, "CORE_RESET_ADDRESS"=94, "CHIP_RESET_ADDRESS"=95, "REG_RF_TXGENCTRL"=96, "REG_RF_TXIFCTRL"=97, "REG_RF_TXRF_SEL_CTRL"=98, "REG_RF_TXRFPWRDEFAULTSET"=99, "REG_RF_RSSITRIM"=100, "REG_RF_TXIFOSCTUNE"=101, "REG_RF_TXIFGAINIMB"=102, "REG_RF_TXIFLOCK"=103, "REG_RF_RXRFLNAGAINTRIM"=104, "REG_RF_RXBIASTR"=105, "REG_RF_RXGENCTRL"=106, "REG_RF_RXIFADCDECLEV"=107, "REG_RF_RXIFDETFILTERTUNE"=108, "REG_RF_RXIFFILTERTUNE"=109, "REG_RF_GENENABLES"=110, "REG_RF_SYNTH_CHANNEL"=111, "REG_TX_RAMP_RTRIM"=112, "REG_TX_RAMP_CTRIM"=113, "REG_RF_XO_TRIM"=114, "REG_RF_SYNTH_SET_TRIM"=115, "REG_RF_ADCCTRL"=116, "REG_RF_ADCOUTPUT"=117, "REG_RF_TXIFAMP"=118, "REG_RF_SYNTH_RTRIM"=119, "REG_RF_SYNTH_CTRIM"=120, "REG_RF_SYNTH_CT"=121, "REG_RF_TXMIXER_IOSTRIM_HIGH_IP"=122, "REG_RF_TXMIXER_IOSTRIM_HIGH_IN"=123, "REG_RF_TXMIXER_IOSTRIM_HIGH_QP"=124, "REG_RF_TXMIXER_IOSTRIM_HIGH_QN"=125, "REG_HX_WUADDR"=126, "REG_REVISION"=127, "REG_NOREG_TEST"=128, "REG_DTEST_RXBUFF"=129, "REG_RXBUFF_NEXT_BLOCK"=130, "REG_RXBUFF_FIRST_IN_PACK"=131, "REG_RXBUFF_FIRST_EMPTY"=132, "REG_MAC_BYPASS"=133, "REG_DTEST_TXBUFF"=134, "REG_TXBUFF_NEXT_BLOCK"=135, "REG_TXBUFF_FIRST_IN_PACK"=136, "REG_TXBUFF_FIRST_EMPTY"=137, "REG_DTEST_SEQ"=138, "REG_DTEST_CKCORR"=139, "REG_MAC_TOPSTATE"=140, "REG_DTEST_INTERFACE"=141, "REG_IFACE_TXRX_BYPASS"=142, "REG_MAC_TXRXWAIT"=143, "REG_MAC_TXRFRAMP"=144, "REG_MAC_TRAINWORD"=145, "REG_MAC_TRAINWORD2"=146, "REG_MAC_SETTINGS"=147, "REG_MAC_CALSELECT1"=148, "REG_MAC_CALSELECT2"=149, "REG_MAC_ANTMATCHSEL"=150, "REG_MAC_ANTTUNESEL1"=151, "REG_MAC_ANTTUNESEL2"=152, "REG_MAC_ANTTUNESEL3"=153, "REG_MAC_ANTTUNESTEP"=154, "REG_MAC_WUMODEBURST"=156, "REG_MAC_WUOFFSHORT"=157, "REG_MAC_WUOFFLONG"=158, "REG_MAC_CLKRECCTRL"=159, "REG_HK_MODE_P2"=162, "REG_MAC_ANTTUNERES1"=164, "REG_MAC_ANTTUNERES2"=165, "REG_INTERFACE_MODE_TEST"=171, "REG_TXRXBUFF_BOTH_P2"=172, "REG_TXRXBUFF_P2"=173, "REG_IRQ_RAWSTATUS1_P2"=174, "REG_MAC_TXIFSTATUS1"=176, "REG_MAC_TXIFSTATUS2"=177, "REG_IRQ_RAWSTATUS2_P2"=178, "REG_MAC_TXIFRAMPDELAY"=179, "REG_MAC_TXIFRAMPSLOPE"=180, "REG_MAX_TXIFRAMP"=181, "REG_IRQ_STATUS1_P2"=182, "REG_IRQ_STATUS2_P2"=183, "REG_IRQ_AUXSTATUS_P2"=184, "REG_MAC_UNLOCK"=188, "REG_MAC_TXIFFREQ"=190, "REG_WAKEUP_TESTCTRL1"=192, "REG_WAKEUP_RX_EN_CNT"=193, "REG_WAKEUP_TESTENABLES"=194, "REG_WAKEUP_DTBI_CTRL"=195, "REG_WAKEUP_DTBO_CTRL"=196, "REG_WAKEUP_TESTIOBUFTEST"=197, "REG_WAKEUP_WK_RX_TESTCTRL1"=198, "REG_WAKEUP_WK_RX_TESTCTRL2"=199, "REG_WAKEUP_SENS_SEQUENCE_CTRL"=200, "REG_WAKEUP_LNABIAS"=201, "REG_WAKEUP_DET_TH_TRIM1"=202, "REG_WAKEUP_LNABIAS_NOM1"=203, "REG_WAKEUP_RX_TSHORT_TRIM1"=204, "REG_WAKEUP_LNABIAS_NOM2"=205, "REG_WAKEUP_RX_TLONG_TRIM1"=206, "REG_WAKEUP_LNA_NEGRTRIM_NOM1"=207, "REG_WAKEUP_RX_TBURST_TRIM1"=208, "REG_WAKEUP_RX_LNA_NEGRTRIM_NOM2"=209, "REG_WAKEUP_RX_BB_G_BW_SEL1"=210, "REG_WAKEUP_WK_RX_DET_IOSTRIM1"=212, "REG_WAKEUP_WK_RX_CTRL2"=214, "REG_WAKEUP_WK_RX_RSSIVOSTRIM"=215, "REG_WAKEUP_LNANEGR_EFF"=216, "REG_WAKEUP_XOSU_FAST"=217, "REG_WAKEUP_STROSCPWIDTH1"=218, "REG_WAKEUP_STROSCPERIOD1"=220, "REG_WAKEUP_STROSCPERIOD2"=221, "REG_WAKEUP_WK_RX_LNA_NEGRTRIM1"=222, "REG_RF_TXTESTENABLE"=224, "REG_RF_TXIFTESTMODE"=225, "REG_RF_RXTESTENABLE"=226, "REG_RF_RXIFTESTCTRL1"=227, "REG_RF_RXIFTESTCTRL2"=228, "REG_RF_RXIFTESTCTRL3"=229, "REG_RF_SYNTH_TESTCTRL1"=230, "REG_RF_SYNTH_TESTCTRL2"=231, "REG_RF_SYNTH_TESTCTRL3"=232, "REG_RF_ADCTEST1"=237, "REG_RF_ADCTEST2"=238, "REG_RF_TXMIXER_IOSTRIM_LOW_IP"=240, "REG_RF_TXMIXER_IOSTRIM_LOW_IN"=241, "REG_RF_TXMIXER_ISOTRIM_LOW_QP"=242, "REG_RF_TXMIXER_IOSTRIM_LOW_QN"=243, "REG_RF_SYNTH_KPD"=244, "REG_RF_SYNTH_LOLEV"=245, "REG_RF_TXRFPWRTUNEANTSET"=246, "REG_RF_TXPD_GAIN_CTRL"=247, "REG_RF_SYNTH_STARTUP"=248, "REG_RF_TXRFANTTUNE_TXMODE"=249, "REG_RF_TXRFANTTUNE_RXMODE"=250, "REG_RF_RXRFANTTUNE_TXMODE"=251, "REG_RF_RXRFANTTUNE_RXMODE"=252, "REG_ANTMATCH1"=253, "REG_ANTMATCH2"=254, "REG_REVISION_P2"=255] ("Register")
              n38 = Select(t=6, s=w163, f=2) -> (s? t:f=w170:i32)
              n39 = Select(t=0, s=w163, f=4) -> (s? t:f=w164:i32)
              n40 = for {
                N: w170 -> [_]
                tunnel: w168 -> [w200]
                shift-right: [w199] -> w161
                shift-left: w186 -> [w201]
                tunnel: w185 -> [w198]
                tunnel: w184 -> [w197]
                tunnel: w183 -> [w196]
                tunnel: w182 -> [w195]
                tunnel: w181 -> [w194]
                tunnel: w167 -> [w193]
                tunnel: w164 -> [w190]
                tunnel: u32 50 ("milliseconds to wait") -> [w189]
                tunnel: w158 -> [w188]
                i -> [w191]
                n41 = Add(x=w190, y=w191) -> (x+y=w192:i32)
                n42 = Wait (ms)(milliseconds to wait=w189) -> ()  [unwired: 1 out]
                n43 = case shown="5" w192 {
                  tunnel: w201 -> [w207 w215 w223 w227 w239 w247]
                  tunnel: w200 -> [w203 w209 w216 w229 w233 w241]
                  tunnel: [w206 w214 w222 w231 w238 w246] -> w199
                  tunnel: w198 -> [_ _ _ w224 _ _]
                  tunnel: w197 -> [_ _ w221 _ _ _]
                  tunnel: w196 -> [w202 _ _ _ _ _]
                  tunnel: w195 -> [_ _ _ _ w232 _]
                  tunnel: w194 -> [_ w208 _ _ _ _]
                  tunnel: w193 -> [w204 w210 w217 w228 w234 w242]
                  tunnel: w188 -> [_ _ _ _ _ w240]
                  frame 0, Default {
                    w205 = u16 222 items=["---MANUAL ENTRY---"=1000, "REG_NOREG"=0, "REG_RXBUFF_USED"=1, "REG_RXBUFF_BSIZE"=2, "REG_TXBUFF_USED"=3, "REG_TXBUFF_BSIZE"=4, "REG_TXBUFF_MAXPACKSIZE"=5, "REG_MAC_ERRCLR"=6, "REG_MAC_TRAINNUM"=7, "REG_MAC_SYNCMATCH"=8, "REG_MAC_SYNC1"=9, "REG_MAC_SYNC2"=10, "REG_MAC_SYNC3"=11, "REG_MAC_SYNC4"=12, "REG_MAC_SYNC5"=13, "REG_MAC_MAXBERR"=14, "REG_MAC_ECCORR"=15, "REG_MAC_CRCERR"=16, "REG_MAC_BLKCNT1"=17, "REG_MAC_BLKCNT2"=18, "REG_MAC_IMDTRANSID1"=19, "REG_MAC_IMDTRANSID2"=20, "REG_MAC_IMDTRANSID3"=21, "REG_MAC_COMPANYID"=22, "REG_MAC_MODUSER"=23, "REG_MAC_CHANNEL"=25, "REG_MAC_CLEARWDOG"=26, "REG_MAC_CKCORRTHRESH"=27, "REG_HK_TXADDR"=28, "REG_HK_TXDATA"=29, "REG_HK_TXREPLY"=30, "REG_HK_USERDATA"=31, "REG_HK_USERSTATUS"=32, "REG_HK_LASTADDRESS"=33, "REG_HK_MODE"=34, "REG_MAC_STATUSSEQ"=35, "REG_MAC_MAXRETRIES"=36, "REG_MAC_RESENDTIME"=37, "REG_MAC_POWERSAVETIME"=38, "REG_MAC_HEAD_DET"=39, "REG_MAC_CTRL"=41, "REG_MAC_INITCOM"=42, "REG_INTERFACE_MODE"=43, "REG_TXRXBUFF_BOTH"=44, "REG_TXRXBUFF"=45, "REG_IRQ_RAWSTATUS1"=46, "REG_IRQ_ENABLE1"=47, "REG_IRQ_ENABLESET1"=48, "REG_IRQ_ENABLECLEAR1"=49, "REG_IRQ_RAWSTATUS2"=50, "REG_IRQ_ENABLE2"=51, "REG_IRQ_ENABLESET2"=52, "REG_IRQ_ENABLECLEAR2"=53, "REG_IRQ_STATUS1"=54, "REG_IRQ_STATUS2"=55, "REG_IRQ_AUXSTATUS"=56, "REG_TXBUFF_OVERFLOW"=57, "REG_PO0"=58, "REG_P01"=59, "REG_P02"=60, "REG_P03"=61, "REG_GP0"=62, "REG_GPI"=63, "REG_WAKEUP_245IN"=64, "REG_WAKEUP_COMPANYID"=65, "REG_WAKEUP_IMDTRANSID1"=66, "REG_WAKEUP_IMDTRANSID2"=67, "REG_WAKEUP_IMDTRANSID3"=68, "REG_WAKEUP_CHANNEL"=69, "REG_WAKEUP_MODUSER"=70, "REG_WAKEUP_DEVICEMODE"=71, "REG_WAKEUP_WK_RX_CTRL1"=72, "REG_WAKEUP_STACK_ADDR"=73, "REG_WAKEUP_CTRL"=74, "REG_WAKEUP_STROSCRTRIM"=75, "REG_WAKEUP_BIASTRIM"=76, "REG_WAKEUP_ANT245TUNE"=77, "REG_WAKEUP_WK_RX_RTRIMDET"=78, "REG_WAKEUP_WK_RX_RTRIMDEMOD"=79, "REG_WAKEUP_WK_RX_RSSIGAIN"=80, "REG_WAKEUP_LNAFREQ1"=81, "REG_WAKEUP_STACK"=83, "REG_WAKUP_XOSU"=84, "REG_WAKUP_CNTDROPOUT"=85, "REG_WAKEUP_CRCCTRL"=86, "REG_WAKEUP_CRCWORD1"=87, "REG_WAKEUP_CRCWORD2"=88, "REG_WAKEUP_WK_RX_CTRIM"=89, "REG_WAKEUP_VDDATRIM"=90, "REG_WAKEUP_VDDDTRIM"=91, "REG_WAKEUP_TESTIOBUFEN"=92, "REG_WAKEUP_TESTIOCLAMP"=93, "CORE_RESET_ADDRESS"=94, "CHIP_RESET_ADDRESS"=95, "REG_RF_TXGENCTRL"=96, "REG_RF_TXIFCTRL"=97, "REG_RF_TXRF_SEL_CTRL"=98, "REG_RF_TXRFPWRDEFAULTSET"=99, "REG_RF_RSSITRIM"=100, "REG_RF_TXIFOSCTUNE"=101, "REG_RF_TXIFGAINIMB"=102, "REG_RF_TXIFLOCK"=103, "REG_RF_RXRFLNAGAINTRIM"=104, "REG_RF_RXBIASTR"=105, "REG_RF_RXGENCTRL"=106, "REG_RF_RXIFADCDECLEV"=107, "REG_RF_RXIFDETFILTERTUNE"=108, "REG_RF_RXIFFILTERTUNE"=109, "REG_RF_GENENABLES"=110, "REG_RF_SYNTH_CHANNEL"=111, "REG_TX_RAMP_RTRIM"=112, "REG_TX_RAMP_CTRIM"=113, "REG_RF_XO_TRIM"=114, "REG_RF_SYNTH_SET_TRIM"=115, "REG_RF_ADCCTRL"=116, "REG_RF_ADCOUTPUT"=117, "REG_RF_TXIFAMP"=118, "REG_RF_SYNTH_RTRIM"=119, "REG_RF_SYNTH_CTRIM"=120, "REG_RF_SYNTH_CT"=121, "REG_RF_TXMIXER_IOSTRIM_HIGH_IP"=122, "REG_RF_TXMIXER_IOSTRIM_HIGH_IN"=123, "REG_RF_TXMIXER_IOSTRIM_HIGH_QP"=124, "REG_RF_TXMIXER_IOSTRIM_HIGH_QN"=125, "REG_HX_WUADDR"=126, "REG_REVISION"=127, "REG_NOREG_TEST"=128, "REG_DTEST_RXBUFF"=129, "REG_RXBUFF_NEXT_BLOCK"=130, "REG_RXBUFF_FIRST_IN_PACK"=131, "REG_RXBUFF_FIRST_EMPTY"=132, "REG_MAC_BYPASS"=133, "REG_DTEST_TXBUFF"=134, "REG_TXBUFF_NEXT_BLOCK"=135, "REG_TXBUFF_FIRST_IN_PACK"=136, "REG_TXBUFF_FIRST_EMPTY"=137, "REG_DTEST_SEQ"=138, "REG_DTEST_CKCORR"=139, "REG_MAC_TOPSTATE"=140, "REG_DTEST_INTERFACE"=141, "REG_IFACE_TXRX_BYPASS"=142, "REG_MAC_TXRXWAIT"=143, "REG_MAC_TXRFRAMP"=144, "REG_MAC_TRAINWORD"=145, "REG_MAC_TRAINWORD2"=146, "REG_MAC_SETTINGS"=147, "REG_MAC_CALSELECT1"=148, "REG_MAC_CALSELECT2"=149, "REG_MAC_ANTMATCHSEL"=150, "REG_MAC_ANTTUNESEL1"=151, "REG_MAC_ANTTUNESEL2"=152, "REG_MAC_ANTTUNESEL3"=153, "REG_MAC_ANTTUNESTEP"=154, "REG_MAC_WUMODEBURST"=156, "REG_MAC_WUOFFSHORT"=157, "REG_MAC_WUOFFLONG"=158, "REG_MAC_CLKRECCTRL"=159, "REG_HK_MODE_P2"=162, "REG_MAC_ANTTUNERES1"=164, "REG_MAC_ANTTUNERES2"=165, "REG_INTERFACE_MODE_TEST"=171, "REG_TXRXBUFF_BOTH_P2"=172, "REG_TXRXBUFF_P2"=173, "REG_IRQ_RAWSTATUS1_P2"=174, "REG_MAC_TXIFSTATUS1"=176, "REG_MAC_TXIFSTATUS2"=177, "REG_IRQ_RAWSTATUS2_P2"=178, "REG_MAC_TXIFRAMPDELAY"=179, "REG_MAC_TXIFRAMPSLOPE"=180, "REG_MAX_TXIFRAMP"=181, "REG_IRQ_STATUS1_P2"=182, "REG_IRQ_STATUS2_P2"=183, "REG_IRQ_AUXSTATUS_P2"=184, "REG_MAC_UNLOCK"=188, "REG_MAC_TXIFFREQ"=190, "REG_WAKEUP_TESTCTRL1"=192, "REG_WAKEUP_RX_EN_CNT"=193, "REG_WAKEUP_TESTENABLES"=194, "REG_WAKEUP_DTBI_CTRL"=195, "REG_WAKEUP_DTBO_CTRL"=196, "REG_WAKEUP_TESTIOBUFTEST"=197, "REG_WAKEUP_WK_RX_TESTCTRL1"=198, "REG_WAKEUP_WK_RX_TESTCTRL2"=199, "REG_WAKEUP_SENS_SEQUENCE_CTRL"=200, "REG_WAKEUP_LNABIAS"=201, "REG_WAKEUP_DET_TH_TRIM1"=202, "REG_WAKEUP_LNABIAS_NOM1"=203, "REG_WAKEUP_RX_TSHORT_TRIM1"=204, "REG_WAKEUP_LNABIAS_NOM2"=205, "REG_WAKEUP_RX_TLONG_TRIM1"=206, "REG_WAKEUP_LNA_NEGRTRIM_NOM1"=207, "REG_WAKEUP_RX_TBURST_TRIM1"=208, "REG_WAKEUP_RX_LNA_NEGRTRIM_NOM2"=209, "REG_WAKEUP_RX_BB_G_BW_SEL1"=210, "REG_WAKEUP_WK_RX_DET_IOSTRIM1"=212, "REG_WAKEUP_WK_RX_CTRL2"=214, "REG_WAKEUP_WK_RX_RSSIVOSTRIM"=215, "REG_WAKEUP_LNANEGR_EFF"=216, "REG_WAKEUP_XOSU_FAST"=217, "REG_WAKEUP_STROSCPWIDTH1"=218, "REG_WAKEUP_STROSCPERIOD1"=220, "REG_WAKEUP_STROSCPERIOD2"=221, "REG_WAKEUP_WK_RX_LNA_NEGRTRIM1"=222, "REG_RF_TXTESTENABLE"=224, "REG_RF_TXIFTESTMODE"=225, "REG_RF_RXTESTENABLE"=226, "REG_RF_RXIFTESTCTRL1"=227, "REG_RF_RXIFTESTCTRL2"=228, "REG_RF_RXIFTESTCTRL3"=229, "REG_RF_SYNTH_TESTCTRL1"=230, "REG_RF_SYNTH_TESTCTRL2"=231, "REG_RF_SYNTH_TESTCTRL3"=232, "REG_RF_ADCTEST1"=237, "REG_RF_ADCTEST2"=238, "REG_RF_TXMIXER_IOSTRIM_LOW_IP"=240, "REG_RF_TXMIXER_IOSTRIM_LOW_IN"=241, "REG_RF_TXMIXER_ISOTRIM_LOW_QP"=242, "REG_RF_TXMIXER_IOSTRIM_LOW_QN"=243, "REG_RF_SYNTH_KPD"=244, "REG_RF_SYNTH_LOLEV"=245, "REG_RF_TXRFPWRTUNEANTSET"=246, "REG_RF_TXPD_GAIN_CTRL"=247, "REG_RF_SYNTH_STARTUP"=248, "REG_RF_TXRFANTTUNE_TXMODE"=249, "REG_RF_TXRFANTTUNE_RXMODE"=250, "REG_RF_RXRFANTTUNE_TXMODE"=251, "REG_RF_RXRFANTTUNE_RXMODE"=252, "REG_ANTMATCH1"=253, "REG_ANTMATCH2"=254, "REG_REVISION_P2"=255] ("Register")
                    # "Apply LNA Gain (NEGRTRIM) value"
                    # "Address"
                    n44 = call "MICSD Set Register.vi"("Execute on Remote?(F)"=w204, "error in (no error)"=w207, "Data"=w202, "Address"=w205, "VISA Resource Name"=w203) -> ("error out"=w206:errorcluster)  [unwired: 5 in, 1 out]
                  }
                  frame 1 {
                    w213 = u16 81 items=["---MANUAL ENTRY---"=1000, "REG_NOREG"=0, "REG_RXBUFF_USED"=1, "REG_RXBUFF_BSIZE"=2, "REG_TXBUFF_USED"=3, "REG_TXBUFF_BSIZE"=4, "REG_TXBUFF_MAXPACKSIZE"=5, "REG_MAC_ERRCLR"=6, "REG_MAC_TRAINNUM"=7, "REG_MAC_SYNCMATCH"=8, "REG_MAC_SYNC1"=9, "REG_MAC_SYNC2"=10, "REG_MAC_SYNC3"=11, "REG_MAC_SYNC4"=12, "REG_MAC_SYNC5"=13, "REG_MAC_MAXBERR"=14, "REG_MAC_ECCORR"=15, "REG_MAC_CRCERR"=16, "REG_MAC_BLKCNT1"=17, "REG_MAC_BLKCNT2"=18, "REG_MAC_IMDTRANSID1"=19, "REG_MAC_IMDTRANSID2"=20, "REG_MAC_IMDTRANSID3"=21, "REG_MAC_COMPANYID"=22, "REG_MAC_MODUSER"=23, "REG_MAC_CHANNEL"=25, "REG_MAC_CLEARWDOG"=26, "REG_MAC_CKCORRTHRESH"=27, "REG_HK_TXADDR"=28, "REG_HK_TXDATA"=29, "REG_HK_TXREPLY"=30, "REG_HK_USERDATA"=31, "REG_HK_USERSTATUS"=32, "REG_HK_LASTADDRESS"=33, "REG_HK_MODE"=34, "REG_MAC_STATUSSEQ"=35, "REG_MAC_MAXRETRIES"=36, "REG_MAC_RESENDTIME"=37, "REG_MAC_POWERSAVETIME"=38, "REG_MAC_HEAD_DET"=39, "REG_MAC_CTRL"=41, "REG_MAC_INITCOM"=42, "REG_INTERFACE_MODE"=43, "REG_TXRXBUFF_BOTH"=44, "REG_TXRXBUFF"=45, "REG_IRQ_RAWSTATUS1"=46, "REG_IRQ_ENABLE1"=47, "REG_IRQ_ENABLESET1"=48, "REG_IRQ_ENABLECLEAR1"=49, "REG_IRQ_RAWSTATUS2"=50, "REG_IRQ_ENABLE2"=51, "REG_IRQ_ENABLESET2"=52, "REG_IRQ_ENABLECLEAR2"=53, "REG_IRQ_STATUS1"=54, "REG_IRQ_STATUS2"=55, "REG_IRQ_AUXSTATUS"=56, "REG_TXBUFF_OVERFLOW"=57, "REG_PO0"=58, "REG_P01"=59, "REG_P02"=60, "REG_P03"=61, "REG_GP0"=62, "REG_GPI"=63, "REG_WAKEUP_245IN"=64, "REG_WAKEUP_COMPANYID"=65, "REG_WAKEUP_IMDTRANSID1"=66, "REG_WAKEUP_IMDTRANSID2"=67, "REG_WAKEUP_IMDTRANSID3"=68, "REG_WAKEUP_CHANNEL"=69, "REG_WAKEUP_MODUSER"=70, "REG_WAKEUP_DEVICEMODE"=71, "REG_WAKEUP_WK_RX_CTRL1"=72, "REG_WAKEUP_STACK_ADDR"=73, "REG_WAKEUP_CTRL"=74, "REG_WAKEUP_STROSCRTRIM"=75, "REG_WAKEUP_BIASTRIM"=76, "REG_WAKEUP_ANT245TUNE"=77, "REG_WAKEUP_WK_RX_RTRIMDET"=78, "REG_WAKEUP_WK_RX_RTRIMDEMOD"=79, "REG_WAKEUP_WK_RX_RSSIGAIN"=80, "REG_WAKEUP_LNAFREQ1"=81, "REG_WAKEUP_STACK"=83, "REG_WAKUP_XOSU"=84, "REG_WAKUP_CNTDROPOUT"=85, "REG_WAKEUP_CRCCTRL"=86, "REG_WAKEUP_CRCWORD1"=87, "REG_WAKEUP_CRCWORD2"=88, "REG_WAKEUP_WK_RX_CTRIM"=89, "REG_WAKEUP_VDDATRIM"=90, "REG_WAKEUP_VDDDTRIM"=91, "REG_WAKEUP_TESTIOBUFEN"=92, "REG_WAKEUP_TESTIOCLAMP"=93, "CORE_RESET_ADDRESS"=94, "CHIP_RESET_ADDRESS"=95, "REG_RF_TXGENCTRL"=96, "REG_RF_TXIFCTRL"=97, "REG_RF_TXRF_SEL_CTRL"=98, "REG_RF_TXRFPWRDEFAULTSET"=99, "REG_RF_RSSITRIM"=100, "REG_RF_TXIFOSCTUNE"=101, "REG_RF_TXIFGAINIMB"=102, "REG_RF_TXIFLOCK"=103, "REG_RF_RXRFLNAGAINTRIM"=104, "REG_RF_RXBIASTR"=105, "REG_RF_RXGENCTRL"=106, "REG_RF_RXIFADCDECLEV"=107, "REG_RF_RXIFDETFILTERTUNE"=108, "REG_RF_RXIFFILTERTUNE"=109, "REG_RF_GENENABLES"=110, "REG_RF_SYNTH_CHANNEL"=111, "REG_TX_RAMP_RTRIM"=112, "REG_TX_RAMP_CTRIM"=113, "REG_RF_XO_TRIM"=114, "REG_RF_SYNTH_SET_TRIM"=115, "REG_RF_ADCCTRL"=116, "REG_RF_ADCOUTPUT"=117, "REG_RF_TXIFAMP"=118, "REG_RF_SYNTH_RTRIM"=119, "REG_RF_SYNTH_CTRIM"=120, "REG_RF_SYNTH_CT"=121, "REG_RF_TXMIXER_IOSTRIM_HIGH_IP"=122, "REG_RF_TXMIXER_IOSTRIM_HIGH_IN"=123, "REG_RF_TXMIXER_IOSTRIM_HIGH_QP"=124, "REG_RF_TXMIXER_IOSTRIM_HIGH_QN"=125, "REG_HX_WUADDR"=126, "REG_REVISION"=127, "REG_NOREG_TEST"=128, "REG_DTEST_RXBUFF"=129, "REG_RXBUFF_NEXT_BLOCK"=130, "REG_RXBUFF_FIRST_IN_PACK"=131, "REG_RXBUFF_FIRST_EMPTY"=132, "REG_MAC_BYPASS"=133, "REG_DTEST_TXBUFF"=134, "REG_TXBUFF_NEXT_BLOCK"=135, "REG_TXBUFF_FIRST_IN_PACK"=136, "REG_TXBUFF_FIRST_EMPTY"=137, "REG_DTEST_SEQ"=138, "REG_DTEST_CKCORR"=139, "REG_MAC_TOPSTATE"=140, "REG_DTEST_INTERFACE"=141, "REG_IFACE_TXRX_BYPASS"=142, "REG_MAC_TXRXWAIT"=143, "REG_MAC_TXRFRAMP"=144, "REG_MAC_TRAINWORD"=145, "REG_MAC_TRAINWORD2"=146, "REG_MAC_SETTINGS"=147, "REG_MAC_CALSELECT1"=148, "REG_MAC_CALSELECT2"=149, "REG_MAC_ANTMATCHSEL"=150, "REG_MAC_ANTTUNESEL1"=151, "REG_MAC_ANTTUNESEL2"=152, "REG_MAC_ANTTUNESEL3"=153, "REG_MAC_ANTTUNESTEP"=154, "REG_MAC_WUMODEBURST"=156, "REG_MAC_WUOFFSHORT"=157, "REG_MAC_WUOFFLONG"=158, "REG_MAC_CLKRECCTRL"=159, "REG_HK_MODE_P2"=162, "REG_MAC_ANTTUNERES1"=164, "REG_MAC_ANTTUNERES2"=165, "REG_INTERFACE_MODE_TEST"=171, "REG_TXRXBUFF_BOTH_P2"=172, "REG_TXRXBUFF_P2"=173, "REG_IRQ_RAWSTATUS1_P2"=174, "REG_MAC_TXIFSTATUS1"=176, "REG_MAC_TXIFSTATUS2"=177, "REG_IRQ_RAWSTATUS2_P2"=178, "REG_MAC_TXIFRAMPDELAY"=179, "REG_MAC_TXIFRAMPSLOPE"=180, "REG_MAX_TXIFRAMP"=181, "REG_IRQ_STATUS1_P2"=182, "REG_IRQ_STATUS2_P2"=183, "REG_IRQ_AUXSTATUS_P2"=184, "REG_MAC_UNLOCK"=188, "REG_MAC_TXIFFREQ"=190, "REG_WAKEUP_TESTCTRL1"=192, "REG_WAKEUP_RX_EN_CNT"=193, "REG_WAKEUP_TESTENABLES"=194, "REG_WAKEUP_DTBI_CTRL"=195, "REG_WAKEUP_DTBO_CTRL"=196, "REG_WAKEUP_TESTIOBUFTEST"=197, "REG_WAKEUP_WK_RX_TESTCTRL1"=198, "REG_WAKEUP_WK_RX_TESTCTRL2"=199, "REG_WAKEUP_SENS_SEQUENCE_CTRL"=200, "REG_WAKEUP_LNABIAS"=201, "REG_WAKEUP_DET_TH_TRIM1"=202, "REG_WAKEUP_LNABIAS_NOM1"=203, "REG_WAKEUP_RX_TSHORT_TRIM1"=204, "REG_WAKEUP_LNABIAS_NOM2"=205, "REG_WAKEUP_RX_TLONG_TRIM1"=206, "REG_WAKEUP_LNA_NEGRTRIM_NOM1"=207, "REG_WAKEUP_RX_TBURST_TRIM1"=208, "REG_WAKEUP_RX_LNA_NEGRTRIM_NOM2"=209, "REG_WAKEUP_RX_BB_G_BW_SEL1"=210, "REG_WAKEUP_WK_RX_DET_IOSTRIM1"=212, "REG_WAKEUP_WK_RX_CTRL2"=214, "REG_WAKEUP_WK_RX_RSSIVOSTRIM"=215, "REG_WAKEUP_LNANEGR_EFF"=216, "REG_WAKEUP_XOSU_FAST"=217, "REG_WAKEUP_STROSCPWIDTH1"=218, "REG_WAKEUP_STROSCPERIOD1"=220, "REG_WAKEUP_STROSCPERIOD2"=221, "REG_WAKEUP_WK_RX_LNA_NEGRTRIM1"=222, "REG_RF_TXTESTENABLE"=224, "REG_RF_TXIFTESTMODE"=225, "REG_RF_RXTESTENABLE"=226, "REG_RF_RXIFTESTCTRL1"=227, "REG_RF_RXIFTESTCTRL2"=228, "REG_RF_RXIFTESTCTRL3"=229, "REG_RF_SYNTH_TESTCTRL1"=230, "REG_RF_SYNTH_TESTCTRL2"=231, "REG_RF_SYNTH_TESTCTRL3"=232, "REG_RF_ADCTEST1"=237, "REG_RF_ADCTEST2"=238, "REG_RF_TXMIXER_IOSTRIM_LOW_IP"=240, "REG_RF_TXMIXER_IOSTRIM_LOW_IN"=241, "REG_RF_TXMIXER_ISOTRIM_LOW_QP"=242, "REG_RF_TXMIXER_IOSTRIM_LOW_QN"=243, "REG_RF_SYNTH_KPD"=244, "REG_RF_SYNTH_LOLEV"=245, "REG_RF_TXRFPWRTUNEANTSET"=246, "REG_RF_TXPD_GAIN_CTRL"=247, "REG_RF_SYNTH_STARTUP"=248, "REG_RF_TXRFANTTUNE_TXMODE"=249, "REG_RF_TXRFANTTUNE_RXMODE"=250, "REG_RF_RXRFANTTUNE_TXMODE"=251, "REG_RF_RXRFANTTUNE_RXMODE"=252, "REG_ANTMATCH1"=253, "REG_ANTMATCH2"=254, "REG_REVISION_P2"=255] ("Register")
                    # "Apply LNA Frequency Trim value"
                    # "Address"
                    # "Bitmask"
                    n45 = And(x=w208, y=u8 31 ("Data")) -> (x .and. y?=w212:u8)
                    n46 = call "MICSD Set Register.vi"("Execute on Remote?(F)"=w210, "error in (no error)"=w215, "Data"=w212, "Address"=w213, "VISA Resource Name"=w209) -> ("error out"=w214:errorcluster)  [unwired: 5 in, 1 out]
                  }
                  frame 2 {
                    w220 = u16 77 items=["---MANUAL ENTRY---"=1000, "REG_NOREG"=0, "REG_RXBUFF_USED"=1, "REG_RXBUFF_BSIZE"=2, "REG_TXBUFF_USED"=3, "REG_TXBUFF_BSIZE"=4, "REG_TXBUFF_MAXPACKSIZE"=5, "REG_MAC_ERRCLR"=6, "REG_MAC_TRAINNUM"=7, "REG_MAC_SYNCMATCH"=8, "REG_MAC_SYNC1"=9, "REG_MAC_SYNC2"=10, "REG_MAC_SYNC3"=11, "REG_MAC_SYNC4"=12, "REG_MAC_SYNC5"=13, "REG_MAC_MAXBERR"=14, "REG_MAC_ECCORR"=15, "REG_MAC_CRCERR"=16, "REG_MAC_BLKCNT1"=17, "REG_MAC_BLKCNT2"=18, "REG_MAC_IMDTRANSID1"=19, "REG_MAC_IMDTRANSID2"=20, "REG_MAC_IMDTRANSID3"=21, "REG_MAC_COMPANYID"=22, "REG_MAC_MODUSER"=23, "REG_MAC_CHANNEL"=25, "REG_MAC_CLEARWDOG"=26, "REG_MAC_CKCORRTHRESH"=27, "REG_HK_TXADDR"=28, "REG_HK_TXDATA"=29, "REG_HK_TXREPLY"=30, "REG_HK_USERDATA"=31, "REG_HK_USERSTATUS"=32, "REG_HK_LASTADDRESS"=33, "REG_HK_MODE"=34, "REG_MAC_STATUSSEQ"=35, "REG_MAC_MAXRETRIES"=36, "REG_MAC_RESENDTIME"=37, "REG_MAC_POWERSAVETIME"=38, "REG_MAC_HEAD_DET"=39, "REG_MAC_CTRL"=41, "REG_MAC_INITCOM"=42, "REG_INTERFACE_MODE"=43, "REG_TXRXBUFF_BOTH"=44, "REG_TXRXBUFF"=45, "REG_IRQ_RAWSTATUS1"=46, "REG_IRQ_ENABLE1"=47, "REG_IRQ_ENABLESET1"=48, "REG_IRQ_ENABLECLEAR1"=49, "REG_IRQ_RAWSTATUS2"=50, "REG_IRQ_ENABLE2"=51, "REG_IRQ_ENABLESET2"=52, "REG_IRQ_ENABLECLEAR2"=53, "REG_IRQ_STATUS1"=54, "REG_IRQ_STATUS2"=55, "REG_IRQ_AUXSTATUS"=56, "REG_TXBUFF_OVERFLOW"=57, "REG_PO0"=58, "REG_P01"=59, "REG_P02"=60, "REG_P03"=61, "REG_GP0"=62, "REG_GPI"=63, "REG_WAKEUP_245IN"=64, "REG_WAKEUP_COMPANYID"=65, "REG_WAKEUP_IMDTRANSID1"=66, "REG_WAKEUP_IMDTRANSID2"=67, "REG_WAKEUP_IMDTRANSID3"=68, "REG_WAKEUP_CHANNEL"=69, "REG_WAKEUP_MODUSER"=70, "REG_WAKEUP_DEVICEMODE"=71, "REG_WAKEUP_WK_RX_CTRL1"=72, "REG_WAKEUP_STACK_ADDR"=73, "REG_WAKEUP_CTRL"=74, "REG_WAKEUP_STROSCRTRIM"=75, "REG_WAKEUP_BIASTRIM"=76, "REG_WAKEUP_ANT245TUNE"=77, "REG_WAKEUP_WK_RX_RTRIMDET"=78, "REG_WAKEUP_WK_RX_RTRIMDEMOD"=79, "REG_WAKEUP_WK_RX_RSSIGAIN"=80, "REG_WAKEUP_LNAFREQ1"=81, "REG_WAKEUP_STACK"=83, "REG_WAKUP_XOSU"=84, "REG_WAKUP_CNTDROPOUT"=85, "REG_WAKEUP_CRCCTRL"=86, "REG_WAKEUP_CRCWORD1"=87, "REG_WAKEUP_CRCWORD2"=88, "REG_WAKEUP_WK_RX_CTRIM"=89, "REG_WAKEUP_VDDATRIM"=90, "REG_WAKEUP_VDDDTRIM"=91, "REG_WAKEUP_TESTIOBUFEN"=92, "REG_WAKEUP_TESTIOCLAMP"=93, "CORE_RESET_ADDRESS"=94, "CHIP_RESET_ADDRESS"=95, "REG_RF_TXGENCTRL"=96, "REG_RF_TXIFCTRL"=97, "REG_RF_TXRF_SEL_CTRL"=98, "REG_RF_TXRFPWRDEFAULTSET"=99, "REG_RF_RSSITRIM"=100, "REG_RF_TXIFOSCTUNE"=101, "REG_RF_TXIFGAINIMB"=102, "REG_RF_TXIFLOCK"=103, "REG_RF_RXRFLNAGAINTRIM"=104, "REG_RF_RXBIASTR"=105, "REG_RF_RXGENCTRL"=106, "REG_RF_RXIFADCDECLEV"=107, "REG_RF_RXIFDETFILTERTUNE"=108, "REG_RF_RXIFFILTERTUNE"=109, "REG_RF_GENENABLES"=110, "REG_RF_SYNTH_CHANNEL"=111, "REG_TX_RAMP_RTRIM"=112, "REG_TX_RAMP_CTRIM"=113, "REG_RF_XO_TRIM"=114, "REG_RF_SYNTH_SET_TRIM"=115, "REG_RF_ADCCTRL"=116, "REG_RF_ADCOUTPUT"=117, "REG_RF_TXIFAMP"=118, "REG_RF_SYNTH_RTRIM"=119, "REG_RF_SYNTH_CTRIM"=120, "REG_RF_SYNTH_CT"=121, "REG_RF_TXMIXER_IOSTRIM_HIGH_IP"=122, "REG_RF_TXMIXER_IOSTRIM_HIGH_IN"=123, "REG_RF_TXMIXER_IOSTRIM_HIGH_QP"=124, "REG_RF_TXMIXER_IOSTRIM_HIGH_QN"=125, "REG_HX_WUADDR"=126, "REG_REVISION"=127, "REG_NOREG_TEST"=128, "REG_DTEST_RXBUFF"=129, "REG_RXBUFF_NEXT_BLOCK"=130, "REG_RXBUFF_FIRST_IN_PACK"=131, "REG_RXBUFF_FIRST_EMPTY"=132, "REG_MAC_BYPASS"=133, "REG_DTEST_TXBUFF"=134, "REG_TXBUFF_NEXT_BLOCK"=135, "REG_TXBUFF_FIRST_IN_PACK"=136, "REG_TXBUFF_FIRST_EMPTY"=137, "REG_DTEST_SEQ"=138, "REG_DTEST_CKCORR"=139, "REG_MAC_TOPSTATE"=140, "REG_DTEST_INTERFACE"=141, "REG_IFACE_TXRX_BYPASS"=142, "REG_MAC_TXRXWAIT"=143, "REG_MAC_TXRFRAMP"=144, "REG_MAC_TRAINWORD"=145, "REG_MAC_TRAINWORD2"=146, "REG_MAC_SETTINGS"=147, "REG_MAC_CALSELECT1"=148, "REG_MAC_CALSELECT2"=149, "REG_MAC_ANTMATCHSEL"=150, "REG_MAC_ANTTUNESEL1"=151, "REG_MAC_ANTTUNESEL2"=152, "REG_MAC_ANTTUNESEL3"=153, "REG_MAC_ANTTUNESTEP"=154, "REG_MAC_WUMODEBURST"=156, "REG_MAC_WUOFFSHORT"=157, "REG_MAC_WUOFFLONG"=158, "REG_MAC_CLKRECCTRL"=159, "REG_HK_MODE_P2"=162, "REG_MAC_ANTTUNERES1"=164, "REG_MAC_ANTTUNERES2"=165, "REG_INTERFACE_MODE_TEST"=171, "REG_TXRXBUFF_BOTH_P2"=172, "REG_TXRXBUFF_P2"=173, "REG_IRQ_RAWSTATUS1_P2"=174, "REG_MAC_TXIFSTATUS1"=176, "REG_MAC_TXIFSTATUS2"=177, "REG_IRQ_RAWSTATUS2_P2"=178, "REG_MAC_TXIFRAMPDELAY"=179, "REG_MAC_TXIFRAMPSLOPE"=180, "REG_MAX_TXIFRAMP"=181, "REG_IRQ_STATUS1_P2"=182, "REG_IRQ_STATUS2_P2"=183, "REG_IRQ_AUXSTATUS_P2"=184, "REG_MAC_UNLOCK"=188, "REG_MAC_TXIFFREQ"=190, "REG_WAKEUP_TESTCTRL1"=192, "REG_WAKEUP_RX_EN_CNT"=193, "REG_WAKEUP_TESTENABLES"=194, "REG_WAKEUP_DTBI_CTRL"=195, "REG_WAKEUP_DTBO_CTRL"=196, "REG_WAKEUP_TESTIOBUFTEST"=197, "REG_WAKEUP_WK_RX_TESTCTRL1"=198, "REG_WAKEUP_WK_RX_TESTCTRL2"=199, "REG_WAKEUP_SENS_SEQUENCE_CTRL"=200, "REG_WAKEUP_LNABIAS"=201, "REG_WAKEUP_DET_TH_TRIM1"=202, "REG_WAKEUP_LNABIAS_NOM1"=203, "REG_WAKEUP_RX_TSHORT_TRIM1"=204, "REG_WAKEUP_LNABIAS_NOM2"=205, "REG_WAKEUP_RX_TLONG_TRIM1"=206, "REG_WAKEUP_LNA_NEGRTRIM_NOM1"=207, "REG_WAKEUP_RX_TBURST_TRIM1"=208, "REG_WAKEUP_RX_LNA_NEGRTRIM_NOM2"=209, "REG_WAKEUP_RX_BB_G_BW_SEL1"=210, "REG_WAKEUP_WK_RX_DET_IOSTRIM1"=212, "REG_WAKEUP_WK_RX_CTRL2"=214, "REG_WAKEUP_WK_RX_RSSIVOSTRIM"=215, "REG_WAKEUP_LNANEGR_EFF"=216, "REG_WAKEUP_XOSU_FAST"=217, "REG_WAKEUP_STROSCPWIDTH1"=218, "REG_WAKEUP_STROSCPERIOD1"=220, "REG_WAKEUP_STROSCPERIOD2"=221, "REG_WAKEUP_WK_RX_LNA_NEGRTRIM1"=222, "REG_RF_TXTESTENABLE"=224, "REG_RF_TXIFTESTMODE"=225, "REG_RF_RXTESTENABLE"=226, "REG_RF_RXIFTESTCTRL1"=227, "REG_RF_RXIFTESTCTRL2"=228, "REG_RF_RXIFTESTCTRL3"=229, "REG_RF_SYNTH_TESTCTRL1"=230, "REG_RF_SYNTH_TESTCTRL2"=231, "REG_RF_SYNTH_TESTCTRL3"=232, "REG_RF_ADCTEST1"=237, "REG_RF_ADCTEST2"=238, "REG_RF_TXMIXER_IOSTRIM_LOW_IP"=240, "REG_RF_TXMIXER_IOSTRIM_LOW_IN"=241, "REG_RF_TXMIXER_ISOTRIM_LOW_QP"=242, "REG_RF_TXMIXER_IOSTRIM_LOW_QN"=243, "REG_RF_SYNTH_KPD"=244, "REG_RF_SYNTH_LOLEV"=245, "REG_RF_TXRFPWRTUNEANTSET"=246, "REG_RF_TXPD_GAIN_CTRL"=247, "REG_RF_SYNTH_STARTUP"=248, "REG_RF_TXRFANTTUNE_TXMODE"=249, "REG_RF_TXRFANTTUNE_RXMODE"=250, "REG_RF_RXRFANTTUNE_TXMODE"=251, "REG_RF_RXRFANTTUNE_RXMODE"=252, "REG_ANTMATCH1"=253, "REG_ANTMATCH2"=254, "REG_REVISION_P2"=255] ("Register")
                    # "Apply 2.45 Antenna Tune value"
                    # "Address"
                    # "Bitmask"
                    n47 = And(x=w221, y=u8 15 ("Data")) -> (x .and. y?=w219:u8)
                    n48 = call "MICSD Set Register.vi"("Execute on Remote?(F)"=w217, "error in (no error)"=w223, "Data"=w219, "Address"=w220, "VISA Resource Name"=w216) -> ("error out"=w222:errorcluster)  [unwired: 5 in, 1 out]
                  }
                  frame 3 {
                    w226 = u16 215 items=["---MANUAL ENTRY---"=1000, "REG_NOREG"=0, "REG_RXBUFF_USED"=1, "REG_RXBUFF_BSIZE"=2, "REG_TXBUFF_USED"=3, "REG_TXBUFF_BSIZE"=4, "REG_TXBUFF_MAXPACKSIZE"=5, "REG_MAC_ERRCLR"=6, "REG_MAC_TRAINNUM"=7, "REG_MAC_SYNCMATCH"=8, "REG_MAC_SYNC1"=9, "REG_MAC_SYNC2"=10, "REG_MAC_SYNC3"=11, "REG_MAC_SYNC4"=12, "REG_MAC_SYNC5"=13, "REG_MAC_MAXBERR"=14, "REG_MAC_ECCORR"=15, "REG_MAC_CRCERR"=16, "REG_MAC_BLKCNT1"=17, "REG_MAC_BLKCNT2"=18, "REG_MAC_IMDTRANSID1"=19, "REG_MAC_IMDTRANSID2"=20, "REG_MAC_IMDTRANSID3"=21, "REG_MAC_COMPANYID"=22, "REG_MAC_MODUSER"=23, "REG_MAC_CHANNEL"=25, "REG_MAC_CLEARWDOG"=26, "REG_MAC_CKCORRTHRESH"=27, "REG_HK_TXADDR"=28, "REG_HK_TXDATA"=29, "REG_HK_TXREPLY"=30, "REG_HK_USERDATA"=31, "REG_HK_USERSTATUS"=32, "REG_HK_LASTADDRESS"=33, "REG_HK_MODE"=34, "REG_MAC_STATUSSEQ"=35, "REG_MAC_MAXRETRIES"=36, "REG_MAC_RESENDTIME"=37, "REG_MAC_POWERSAVETIME"=38, "REG_MAC_HEAD_DET"=39, "REG_MAC_CTRL"=41, "REG_MAC_INITCOM"=42, "REG_INTERFACE_MODE"=43, "REG_TXRXBUFF_BOTH"=44, "REG_TXRXBUFF"=45, "REG_IRQ_RAWSTATUS1"=46, "REG_IRQ_ENABLE1"=47, "REG_IRQ_ENABLESET1"=48, "REG_IRQ_ENABLECLEAR1"=49, "REG_IRQ_RAWSTATUS2"=50, "REG_IRQ_ENABLE2"=51, "REG_IRQ_ENABLESET2"=52, "REG_IRQ_ENABLECLEAR2"=53, "REG_IRQ_STATUS1"=54, "REG_IRQ_STATUS2"=55, "REG_IRQ_AUXSTATUS"=56, "REG_TXBUFF_OVERFLOW"=57, "REG_PO0"=58, "REG_P01"=59, "REG_P02"=60, "REG_P03"=61, "REG_GP0"=62, "REG_GPI"=63, "REG_WAKEUP_245IN"=64, "REG_WAKEUP_COMPANYID"=65, "REG_WAKEUP_IMDTRANSID1"=66, "REG_WAKEUP_IMDTRANSID2"=67, "REG_WAKEUP_IMDTRANSID3"=68, "REG_WAKEUP_CHANNEL"=69, "REG_WAKEUP_MODUSER"=70, "REG_WAKEUP_DEVICEMODE"=71, "REG_WAKEUP_WK_RX_CTRL1"=72, "REG_WAKEUP_STACK_ADDR"=73, "REG_WAKEUP_CTRL"=74, "REG_WAKEUP_STROSCRTRIM"=75, "REG_WAKEUP_BIASTRIM"=76, "REG_WAKEUP_ANT245TUNE"=77, "REG_WAKEUP_WK_RX_RTRIMDET"=78, "REG_WAKEUP_WK_RX_RTRIMDEMOD"=79, "REG_WAKEUP_WK_RX_RSSIGAIN"=80, "REG_WAKEUP_LNAFREQ1"=81, "REG_WAKEUP_STACK"=83, "REG_WAKUP_XOSU"=84, "REG_WAKUP_CNTDROPOUT"=85, "REG_WAKEUP_CRCCTRL"=86, "REG_WAKEUP_CRCWORD1"=87, "REG_WAKEUP_CRCWORD2"=88, "REG_WAKEUP_WK_RX_CTRIM"=89, "REG_WAKEUP_VDDATRIM"=90, "REG_WAKEUP_VDDDTRIM"=91, "REG_WAKEUP_TESTIOBUFEN"=92, "REG_WAKEUP_TESTIOCLAMP"=93, "CORE_RESET_ADDRESS"=94, "CHIP_RESET_ADDRESS"=95, "REG_RF_TXGENCTRL"=96, "REG_RF_TXIFCTRL"=97, "REG_RF_TXRF_SEL_CTRL"=98, "REG_RF_TXRFPWRDEFAULTSET"=99, "REG_RF_RSSITRIM"=100, "REG_RF_TXIFOSCTUNE"=101, "REG_RF_TXIFGAINIMB"=102, "REG_RF_TXIFLOCK"=103, "REG_RF_RXRFLNAGAINTRIM"=104, "REG_RF_RXBIASTR"=105, "REG_RF_RXGENCTRL"=106, "REG_RF_RXIFADCDECLEV"=107, "REG_RF_RXIFDETFILTERTUNE"=108, "REG_RF_RXIFFILTERTUNE"=109, "REG_RF_GENENABLES"=110, "REG_RF_SYNTH_CHANNEL"=111, "REG_TX_RAMP_RTRIM"=112, "REG_TX_RAMP_CTRIM"=113, "REG_RF_XO_TRIM"=114, "REG_RF_SYNTH_SET_TRIM"=115, "REG_RF_ADCCTRL"=116, "REG_RF_ADCOUTPUT"=117, "REG_RF_TXIFAMP"=118, "REG_RF_SYNTH_RTRIM"=119, "REG_RF_SYNTH_CTRIM"=120, "REG_RF_SYNTH_CT"=121, "REG_RF_TXMIXER_IOSTRIM_HIGH_IP"=122, "REG_RF_TXMIXER_IOSTRIM_HIGH_IN"=123, "REG_RF_TXMIXER_IOSTRIM_HIGH_QP"=124, "REG_RF_TXMIXER_IOSTRIM_HIGH_QN"=125, "REG_HX_WUADDR"=126, "REG_REVISION"=127, "REG_NOREG_TEST"=128, "REG_DTEST_RXBUFF"=129, "REG_RXBUFF_NEXT_BLOCK"=130, "REG_RXBUFF_FIRST_IN_PACK"=131, "REG_RXBUFF_FIRST_EMPTY"=132, "REG_MAC_BYPASS"=133, "REG_DTEST_TXBUFF"=134, "REG_TXBUFF_NEXT_BLOCK"=135, "REG_TXBUFF_FIRST_IN_PACK"=136, "REG_TXBUFF_FIRST_EMPTY"=137, "REG_DTEST_SEQ"=138, "REG_DTEST_CKCORR"=139, "REG_MAC_TOPSTATE"=140, "REG_DTEST_INTERFACE"=141, "REG_IFACE_TXRX_BYPASS"=142, "REG_MAC_TXRXWAIT"=143, "REG_MAC_TXRFRAMP"=144, "REG_MAC_TRAINWORD"=145, "REG_MAC_TRAINWORD2"=146, "REG_MAC_SETTINGS"=147, "REG_MAC_CALSELECT1"=148, "REG_MAC_CALSELECT2"=149, "REG_MAC_ANTMATCHSEL"=150, "REG_MAC_ANTTUNESEL1"=151, "REG_MAC_ANTTUNESEL2"=152, "REG_MAC_ANTTUNESEL3"=153, "REG_MAC_ANTTUNESTEP"=154, "REG_MAC_WUMODEBURST"=156, "REG_MAC_WUOFFSHORT"=157, "REG_MAC_WUOFFLONG"=158, "REG_MAC_CLKRECCTRL"=159, "REG_HK_MODE_P2"=162, "REG_MAC_ANTTUNERES1"=164, "REG_MAC_ANTTUNERES2"=165, "REG_INTERFACE_MODE_TEST"=171, "REG_TXRXBUFF_BOTH_P2"=172, "REG_TXRXBUFF_P2"=173, "REG_IRQ_RAWSTATUS1_P2"=174, "REG_MAC_TXIFSTATUS1"=176, "REG_MAC_TXIFSTATUS2"=177, "REG_IRQ_RAWSTATUS2_P2"=178, "REG_MAC_TXIFRAMPDELAY"=179, "REG_MAC_TXIFRAMPSLOPE"=180, "REG_MAX_TXIFRAMP"=181, "REG_IRQ_STATUS1_P2"=182, "REG_IRQ_STATUS2_P2"=183, "REG_IRQ_AUXSTATUS_P2"=184, "REG_MAC_UNLOCK"=188, "REG_MAC_TXIFFREQ"=190, "REG_WAKEUP_TESTCTRL1"=192, "REG_WAKEUP_RX_EN_CNT"=193, "REG_WAKEUP_TESTENABLES"=194, "REG_WAKEUP_DTBI_CTRL"=195, "REG_WAKEUP_DTBO_CTRL"=196, "REG_WAKEUP_TESTIOBUFTEST"=197, "REG_WAKEUP_WK_RX_TESTCTRL1"=198, "REG_WAKEUP_WK_RX_TESTCTRL2"=199, "REG_WAKEUP_SENS_SEQUENCE_CTRL"=200, "REG_WAKEUP_LNABIAS"=201, "REG_WAKEUP_DET_TH_TRIM1"=202, "REG_WAKEUP_LNABIAS_NOM1"=203, "REG_WAKEUP_RX_TSHORT_TRIM1"=204, "REG_WAKEUP_LNABIAS_NOM2"=205, "REG_WAKEUP_RX_TLONG_TRIM1"=206, "REG_WAKEUP_LNA_NEGRTRIM_NOM1"=207, "REG_WAKEUP_RX_TBURST_TRIM1"=208, "REG_WAKEUP_RX_LNA_NEGRTRIM_NOM2"=209, "REG_WAKEUP_RX_BB_G_BW_SEL1"=210, "REG_WAKEUP_WK_RX_DET_IOSTRIM1"=212, "REG_WAKEUP_WK_RX_CTRL2"=214, "REG_WAKEUP_WK_RX_RSSIVOSTRIM"=215, "REG_WAKEUP_LNANEGR_EFF"=216, "REG_WAKEUP_XOSU_FAST"=217, "REG_WAKEUP_STROSCPWIDTH1"=218, "REG_WAKEUP_STROSCPERIOD1"=220, "REG_WAKEUP_STROSCPERIOD2"=221, "REG_WAKEUP_WK_RX_LNA_NEGRTRIM1"=222, "REG_RF_TXTESTENABLE"=224, "REG_RF_TXIFTESTMODE"=225, "REG_RF_RXTESTENABLE"=226, "REG_RF_RXIFTESTCTRL1"=227, "REG_RF_RXIFTESTCTRL2"=228, "REG_RF_RXIFTESTCTRL3"=229, "REG_RF_SYNTH_TESTCTRL1"=230, "REG_RF_SYNTH_TESTCTRL2"=231, "REG_RF_SYNTH_TESTCTRL3"=232, "REG_RF_ADCTEST1"=237, "REG_RF_ADCTEST2"=238, "REG_RF_TXMIXER_IOSTRIM_LOW_IP"=240, "REG_RF_TXMIXER_IOSTRIM_LOW_IN"=241, "REG_RF_TXMIXER_ISOTRIM_LOW_QP"=242, "REG_RF_TXMIXER_IOSTRIM_LOW_QN"=243, "REG_RF_SYNTH_KPD"=244, "REG_RF_SYNTH_LOLEV"=245, "REG_RF_TXRFPWRTUNEANTSET"=246, "REG_RF_TXPD_GAIN_CTRL"=247, "REG_RF_SYNTH_STARTUP"=248, "REG_RF_TXRFANTTUNE_TXMODE"=249, "REG_RF_TXRFANTTUNE_RXMODE"=250, "REG_RF_RXRFANTTUNE_TXMODE"=251, "REG_RF_RXRFANTTUNE_RXMODE"=252, "REG_ANTMATCH1"=253, "REG_ANTMATCH2"=254, "REG_REVISION_P2"=255] ("Register")
                    # "Shift \"Baseband Gain\" value left by two bits, apply to BW_SEL1 register with 0x1C Bitmask"
                    # "Address"
                    # "Bitmask"
                    n49 = And(x=w224, y=u8 31 ("Data")) -> (x .and. y?=w225:u8)
                    n50 = call "MICSD Set Register.vi"("Execute on Remote?(F)"=w228, "error in (no error)"=w227, "Data"=w225, "Address"=w226, "VISA Resource Name"=w229) -> ("error out"=w231:errorcluster)  [unwired: 5 in, 1 out]
                  }
                  frame 4 {
                    w237 = u16 212 items=["---MANUAL ENTRY---"=1000, "REG_NOREG"=0, "REG_RXBUFF_USED"=1, "REG_RXBUFF_BSIZE"=2, "REG_TXBUFF_USED"=3, "REG_TXBUFF_BSIZE"=4, "REG_TXBUFF_MAXPACKSIZE"=5, "REG_MAC_ERRCLR"=6, "REG_MAC_TRAINNUM"=7, "REG_MAC_SYNCMATCH"=8, "REG_MAC_SYNC1"=9, "REG_MAC_SYNC2"=10, "REG_MAC_SYNC3"=11, "REG_MAC_SYNC4"=12, "REG_MAC_SYNC5"=13, "REG_MAC_MAXBERR"=14, "REG_MAC_ECCORR"=15, "REG_MAC_CRCERR"=16, "REG_MAC_BLKCNT1"=17, "REG_MAC_BLKCNT2"=18, "REG_MAC_IMDTRANSID1"=19, "REG_MAC_IMDTRANSID2"=20, "REG_MAC_IMDTRANSID3"=21, "REG_MAC_COMPANYID"=22, "REG_MAC_MODUSER"=23, "REG_MAC_CHANNEL"=25, "REG_MAC_CLEARWDOG"=26, "REG_MAC_CKCORRTHRESH"=27, "REG_HK_TXADDR"=28, "REG_HK_TXDATA"=29, "REG_HK_TXREPLY"=30, "REG_HK_USERDATA"=31, "REG_HK_USERSTATUS"=32, "REG_HK_LASTADDRESS"=33, "REG_HK_MODE"=34, "REG_MAC_STATUSSEQ"=35, "REG_MAC_MAXRETRIES"=36, "REG_MAC_RESENDTIME"=37, "REG_MAC_POWERSAVETIME"=38, "REG_MAC_HEAD_DET"=39, "REG_MAC_CTRL"=41, "REG_MAC_INITCOM"=42, "REG_INTERFACE_MODE"=43, "REG_TXRXBUFF_BOTH"=44, "REG_TXRXBUFF"=45, "REG_IRQ_RAWSTATUS1"=46, "REG_IRQ_ENABLE1"=47, "REG_IRQ_ENABLESET1"=48, "REG_IRQ_ENABLECLEAR1"=49, "REG_IRQ_RAWSTATUS2"=50, "REG_IRQ_ENABLE2"=51, "REG_IRQ_ENABLESET2"=52, "REG_IRQ_ENABLECLEAR2"=53, "REG_IRQ_STATUS1"=54, "REG_IRQ_STATUS2"=55, "REG_IRQ_AUXSTATUS"=56, "REG_TXBUFF_OVERFLOW"=57, "REG_PO0"=58, "REG_P01"=59, "REG_P02"=60, "REG_P03"=61, "REG_GP0"=62, "REG_GPI"=63, "REG_WAKEUP_245IN"=64, "REG_WAKEUP_COMPANYID"=65, "REG_WAKEUP_IMDTRANSID1"=66, "REG_WAKEUP_IMDTRANSID2"=67, "REG_WAKEUP_IMDTRANSID3"=68, "REG_WAKEUP_CHANNEL"=69, "REG_WAKEUP_MODUSER"=70, "REG_WAKEUP_DEVICEMODE"=71, "REG_WAKEUP_WK_RX_CTRL1"=72, "REG_WAKEUP_STACK_ADDR"=73, "REG_WAKEUP_CTRL"=74, "REG_WAKEUP_STROSCRTRIM"=75, "REG_WAKEUP_BIASTRIM"=76, "REG_WAKEUP_ANT245TUNE"=77, "REG_WAKEUP_WK_RX_RTRIMDET"=78, "REG_WAKEUP_WK_RX_RTRIMDEMOD"=79, "REG_WAKEUP_WK_RX_RSSIGAIN"=80, "REG_WAKEUP_LNAFREQ1"=81, "REG_WAKEUP_STACK"=83, "REG_WAKUP_XOSU"=84, "REG_WAKUP_CNTDROPOUT"=85, "REG_WAKEUP_CRCCTRL"=86, "REG_WAKEUP_CRCWORD1"=87, "REG_WAKEUP_CRCWORD2"=88, "REG_WAKEUP_WK_RX_CTRIM"=89, "REG_WAKEUP_VDDATRIM"=90, "REG_WAKEUP_VDDDTRIM"=91, "REG_WAKEUP_TESTIOBUFEN"=92, "REG_WAKEUP_TESTIOCLAMP"=93, "CORE_RESET_ADDRESS"=94, "CHIP_RESET_ADDRESS"=95, "REG_RF_TXGENCTRL"=96, "REG_RF_TXIFCTRL"=97, "REG_RF_TXRF_SEL_CTRL"=98, "REG_RF_TXRFPWRDEFAULTSET"=99, "REG_RF_RSSITRIM"=100, "REG_RF_TXIFOSCTUNE"=101, "REG_RF_TXIFGAINIMB"=102, "REG_RF_TXIFLOCK"=103, "REG_RF_RXRFLNAGAINTRIM"=104, "REG_RF_RXBIASTR"=105, "REG_RF_RXGENCTRL"=106, "REG_RF_RXIFADCDECLEV"=107, "REG_RF_RXIFDETFILTERTUNE"=108, "REG_RF_RXIFFILTERTUNE"=109, "REG_RF_GENENABLES"=110, "REG_RF_SYNTH_CHANNEL"=111, "REG_TX_RAMP_RTRIM"=112, "REG_TX_RAMP_CTRIM"=113, "REG_RF_XO_TRIM"=114, "REG_RF_SYNTH_SET_TRIM"=115, "REG_RF_ADCCTRL"=116, "REG_RF_ADCOUTPUT"=117, "REG_RF_TXIFAMP"=118, "REG_RF_SYNTH_RTRIM"=119, "REG_RF_SYNTH_CTRIM"=120, "REG_RF_SYNTH_CT"=121, "REG_RF_TXMIXER_IOSTRIM_HIGH_IP"=122, "REG_RF_TXMIXER_IOSTRIM_HIGH_IN"=123, "REG_RF_TXMIXER_IOSTRIM_HIGH_QP"=124, "REG_RF_TXMIXER_IOSTRIM_HIGH_QN"=125, "REG_HX_WUADDR"=126, "REG_REVISION"=127, "REG_NOREG_TEST"=128, "REG_DTEST_RXBUFF"=129, "REG_RXBUFF_NEXT_BLOCK"=130, "REG_RXBUFF_FIRST_IN_PACK"=131, "REG_RXBUFF_FIRST_EMPTY"=132, "REG_MAC_BYPASS"=133, "REG_DTEST_TXBUFF"=134, "REG_TXBUFF_NEXT_BLOCK"=135, "REG_TXBUFF_FIRST_IN_PACK"=136, "REG_TXBUFF_FIRST_EMPTY"=137, "REG_DTEST_SEQ"=138, "REG_DTEST_CKCORR"=139, "REG_MAC_TOPSTATE"=140, "REG_DTEST_INTERFACE"=141, "REG_IFACE_TXRX_BYPASS"=142, "REG_MAC_TXRXWAIT"=143, "REG_MAC_TXRFRAMP"=144, "REG_MAC_TRAINWORD"=145, "REG_MAC_TRAINWORD2"=146, "REG_MAC_SETTINGS"=147, "REG_MAC_CALSELECT1"=148, "REG_MAC_CALSELECT2"=149, "REG_MAC_ANTMATCHSEL"=150, "REG_MAC_ANTTUNESEL1"=151, "REG_MAC_ANTTUNESEL2"=152, "REG_MAC_ANTTUNESEL3"=153, "REG_MAC_ANTTUNESTEP"=154, "REG_MAC_WUMODEBURST"=156, "REG_MAC_WUOFFSHORT"=157, "REG_MAC_WUOFFLONG"=158, "REG_MAC_CLKRECCTRL"=159, "REG_HK_MODE_P2"=162, "REG_MAC_ANTTUNERES1"=164, "REG_MAC_ANTTUNERES2"=165, "REG_INTERFACE_MODE_TEST"=171, "REG_TXRXBUFF_BOTH_P2"=172, "REG_TXRXBUFF_P2"=173, "REG_IRQ_RAWSTATUS1_P2"=174, "REG_MAC_TXIFSTATUS1"=176, "REG_MAC_TXIFSTATUS2"=177, "REG_IRQ_RAWSTATUS2_P2"=178, "REG_MAC_TXIFRAMPDELAY"=179, "REG_MAC_TXIFRAMPSLOPE"=180, "REG_MAX_TXIFRAMP"=181, "REG_IRQ_STATUS1_P2"=182, "REG_IRQ_STATUS2_P2"=183, "REG_IRQ_AUXSTATUS_P2"=184, "REG_MAC_UNLOCK"=188, "REG_MAC_TXIFFREQ"=190, "REG_WAKEUP_TESTCTRL1"=192, "REG_WAKEUP_RX_EN_CNT"=193, "REG_WAKEUP_TESTENABLES"=194, "REG_WAKEUP_DTBI_CTRL"=195, "REG_WAKEUP_DTBO_CTRL"=196, "REG_WAKEUP_TESTIOBUFTEST"=197, "REG_WAKEUP_WK_RX_TESTCTRL1"=198, "REG_WAKEUP_WK_RX_TESTCTRL2"=199, "REG_WAKEUP_SENS_SEQUENCE_CTRL"=200, "REG_WAKEUP_LNABIAS"=201, "REG_WAKEUP_DET_TH_TRIM1"=202, "REG_WAKEUP_LNABIAS_NOM1"=203, "REG_WAKEUP_RX_TSHORT_TRIM1"=204, "REG_WAKEUP_LNABIAS_NOM2"=205, "REG_WAKEUP_RX_TLONG_TRIM1"=206, "REG_WAKEUP_LNA_NEGRTRIM_NOM1"=207, "REG_WAKEUP_RX_TBURST_TRIM1"=208, "REG_WAKEUP_RX_LNA_NEGRTRIM_NOM2"=209, "REG_WAKEUP_RX_BB_G_BW_SEL1"=210, "REG_WAKEUP_WK_RX_DET_IOSTRIM1"=212, "REG_WAKEUP_WK_RX_CTRL2"=214, "REG_WAKEUP_WK_RX_RSSIVOSTRIM"=215, "REG_WAKEUP_LNANEGR_EFF"=216, "REG_WAKEUP_XOSU_FAST"=217, "REG_WAKEUP_STROSCPWIDTH1"=218, "REG_WAKEUP_STROSCPERIOD1"=220, "REG_WAKEUP_STROSCPERIOD2"=221, "REG_WAKEUP_WK_RX_LNA_NEGRTRIM1"=222, "REG_RF_TXTESTENABLE"=224, "REG_RF_TXIFTESTMODE"=225, "REG_RF_RXTESTENABLE"=226, "REG_RF_RXIFTESTCTRL1"=227, "REG_RF_RXIFTESTCTRL2"=228, "REG_RF_RXIFTESTCTRL3"=229, "REG_RF_SYNTH_TESTCTRL1"=230, "REG_RF_SYNTH_TESTCTRL2"=231, "REG_RF_SYNTH_TESTCTRL3"=232, "REG_RF_ADCTEST1"=237, "REG_RF_ADCTEST2"=238, "REG_RF_TXMIXER_IOSTRIM_LOW_IP"=240, "REG_RF_TXMIXER_IOSTRIM_LOW_IN"=241, "REG_RF_TXMIXER_ISOTRIM_LOW_QP"=242, "REG_RF_TXMIXER_IOSTRIM_LOW_QN"=243, "REG_RF_SYNTH_KPD"=244, "REG_RF_SYNTH_LOLEV"=245, "REG_RF_TXRFPWRTUNEANTSET"=246, "REG_RF_TXPD_GAIN_CTRL"=247, "REG_RF_SYNTH_STARTUP"=248, "REG_RF_TXRFANTTUNE_TXMODE"=249, "REG_RF_TXRFANTTUNE_RXMODE"=250, "REG_RF_RXRFANTTUNE_TXMODE"=251, "REG_RF_RXRFANTTUNE_RXMODE"=252, "REG_ANTMATCH1"=253, "REG_ANTMATCH2"=254, "REG_REVISION_P2"=255] ("Register")
                    # "Apply Detector Trim Value"
                    # "Address"
                    # "Bitmask"
                    n51 = And(x=w232, y=u8 63 ("Data")) -> (x .and. y?=w236:u8)
                    n52 = call "MICSD Set Register.vi"("Execute on Remote?(F)"=w234, "error in (no error)"=w239, "Data"=w236, "Address"=w237, "VISA Resource Name"=w233) -> ("error out"=w238:errorcluster)  [unwired: 5 in, 1 out]
                  }
                  frame 5 {
                    w245 = u16 80 items=["---MANUAL ENTRY---"=1000, "REG_NOREG"=0, "REG_RXBUFF_USED"=1, "REG_RXBUFF_BSIZE"=2, "REG_TXBUFF_USED"=3, "REG_TXBUFF_BSIZE"=4, "REG_TXBUFF_MAXPACKSIZE"=5, "REG_MAC_ERRCLR"=6, "REG_MAC_TRAINNUM"=7, "REG_MAC_SYNCMATCH"=8, "REG_MAC_SYNC1"=9, "REG_MAC_SYNC2"=10, "REG_MAC_SYNC3"=11, "REG_MAC_SYNC4"=12, "REG_MAC_SYNC5"=13, "REG_MAC_MAXBERR"=14, "REG_MAC_ECCORR"=15, "REG_MAC_CRCERR"=16, "REG_MAC_BLKCNT1"=17, "REG_MAC_BLKCNT2"=18, "REG_MAC_IMDTRANSID1"=19, "REG_MAC_IMDTRANSID2"=20, "REG_MAC_IMDTRANSID3"=21, "REG_MAC_COMPANYID"=22, "REG_MAC_MODUSER"=23, "REG_MAC_CHANNEL"=25, "REG_MAC_CLEARWDOG"=26, "REG_MAC_CKCORRTHRESH"=27, "REG_HK_TXADDR"=28, "REG_HK_TXDATA"=29, "REG_HK_TXREPLY"=30, "REG_HK_USERDATA"=31, "REG_HK_USERSTATUS"=32, "REG_HK_LASTADDRESS"=33, "REG_HK_MODE"=34, "REG_MAC_STATUSSEQ"=35, "REG_MAC_MAXRETRIES"=36, "REG_MAC_RESENDTIME"=37, "REG_MAC_POWERSAVETIME"=38, "REG_MAC_HEAD_DET"=39, "REG_MAC_CTRL"=41, "REG_MAC_INITCOM"=42, "REG_INTERFACE_MODE"=43, "REG_TXRXBUFF_BOTH"=44, "REG_TXRXBUFF"=45, "REG_IRQ_RAWSTATUS1"=46, "REG_IRQ_ENABLE1"=47, "REG_IRQ_ENABLESET1"=48, "REG_IRQ_ENABLECLEAR1"=49, "REG_IRQ_RAWSTATUS2"=50, "REG_IRQ_ENABLE2"=51, "REG_IRQ_ENABLESET2"=52, "REG_IRQ_ENABLECLEAR2"=53, "REG_IRQ_STATUS1"=54, "REG_IRQ_STATUS2"=55, "REG_IRQ_AUXSTATUS"=56, "REG_TXBUFF_OVERFLOW"=57, "REG_PO0"=58, "REG_P01"=59, "REG_P02"=60, "REG_P03"=61, "REG_GP0"=62, "REG_GPI"=63, "REG_WAKEUP_245IN"=64, "REG_WAKEUP_COMPANYID"=65, "REG_WAKEUP_IMDTRANSID1"=66, "REG_WAKEUP_IMDTRANSID2"=67, "REG_WAKEUP_IMDTRANSID3"=68, "REG_WAKEUP_CHANNEL"=69, "REG_WAKEUP_MODUSER"=70, "REG_WAKEUP_DEVICEMODE"=71, "REG_WAKEUP_WK_RX_CTRL1"=72, "REG_WAKEUP_STACK_ADDR"=73, "REG_WAKEUP_CTRL"=74, "REG_WAKEUP_STROSCRTRIM"=75, "REG_WAKEUP_BIASTRIM"=76, "REG_WAKEUP_ANT245TUNE"=77, "REG_WAKEUP_WK_RX_RTRIMDET"=78, "REG_WAKEUP_WK_RX_RTRIMDEMOD"=79, "REG_WAKEUP_WK_RX_RSSIGAIN"=80, "REG_WAKEUP_LNAFREQ1"=81, "REG_WAKEUP_STACK"=83, "REG_WAKUP_XOSU"=84, "REG_WAKUP_CNTDROPOUT"=85, "REG_WAKEUP_CRCCTRL"=86, "REG_WAKEUP_CRCWORD1"=87, "REG_WAKEUP_CRCWORD2"=88, "REG_WAKEUP_WK_RX_CTRIM"=89, "REG_WAKEUP_VDDATRIM"=90, "REG_WAKEUP_VDDDTRIM"=91, "REG_WAKEUP_TESTIOBUFEN"=92, "REG_WAKEUP_TESTIOCLAMP"=93, "CORE_RESET_ADDRESS"=94, "CHIP_RESET_ADDRESS"=95, "REG_RF_TXGENCTRL"=96, "REG_RF_TXIFCTRL"=97, "REG_RF_TXRF_SEL_CTRL"=98, "REG_RF_TXRFPWRDEFAULTSET"=99, "REG_RF_RSSITRIM"=100, "REG_RF_TXIFOSCTUNE"=101, "REG_RF_TXIFGAINIMB"=102, "REG_RF_TXIFLOCK"=103, "REG_RF_RXRFLNAGAINTRIM"=104, "REG_RF_RXBIASTR"=105, "REG_RF_RXGENCTRL"=106, "REG_RF_RXIFADCDECLEV"=107, "REG_RF_RXIFDETFILTERTUNE"=108, "REG_RF_RXIFFILTERTUNE"=109, "REG_RF_GENENABLES"=110, "REG_RF_SYNTH_CHANNEL"=111, "REG_TX_RAMP_RTRIM"=112, "REG_TX_RAMP_CTRIM"=113, "REG_RF_XO_TRIM"=114, "REG_RF_SYNTH_SET_TRIM"=115, "REG_RF_ADCCTRL"=116, "REG_RF_ADCOUTPUT"=117, "REG_RF_TXIFAMP"=118, "REG_RF_SYNTH_RTRIM"=119, "REG_RF_SYNTH_CTRIM"=120, "REG_RF_SYNTH_CT"=121, "REG_RF_TXMIXER_IOSTRIM_HIGH_IP"=122, "REG_RF_TXMIXER_IOSTRIM_HIGH_IN"=123, "REG_RF_TXMIXER_IOSTRIM_HIGH_QP"=124, "REG_RF_TXMIXER_IOSTRIM_HIGH_QN"=125, "REG_HX_WUADDR"=126, "REG_REVISION"=127, "REG_NOREG_TEST"=128, "REG_DTEST_RXBUFF"=129, "REG_RXBUFF_NEXT_BLOCK"=130, "REG_RXBUFF_FIRST_IN_PACK"=131, "REG_RXBUFF_FIRST_EMPTY"=132, "REG_MAC_BYPASS"=133, "REG_DTEST_TXBUFF"=134, "REG_TXBUFF_NEXT_BLOCK"=135, "REG_TXBUFF_FIRST_IN_PACK"=136, "REG_TXBUFF_FIRST_EMPTY"=137, "REG_DTEST_SEQ"=138, "REG_DTEST_CKCORR"=139, "REG_MAC_TOPSTATE"=140, "REG_DTEST_INTERFACE"=141, "REG_IFACE_TXRX_BYPASS"=142, "REG_MAC_TXRXWAIT"=143, "REG_MAC_TXRFRAMP"=144, "REG_MAC_TRAINWORD"=145, "REG_MAC_TRAINWORD2"=146, "REG_MAC_SETTINGS"=147, "REG_MAC_CALSELECT1"=148, "REG_MAC_CALSELECT2"=149, "REG_MAC_ANTMATCHSEL"=150, "REG_MAC_ANTTUNESEL1"=151, "REG_MAC_ANTTUNESEL2"=152, "REG_MAC_ANTTUNESEL3"=153, "REG_MAC_ANTTUNESTEP"=154, "REG_MAC_WUMODEBURST"=156, "REG_MAC_WUOFFSHORT"=157, "REG_MAC_WUOFFLONG"=158, "REG_MAC_CLKRECCTRL"=159, "REG_HK_MODE_P2"=162, "REG_MAC_ANTTUNERES1"=164, "REG_MAC_ANTTUNERES2"=165, "REG_INTERFACE_MODE_TEST"=171, "REG_TXRXBUFF_BOTH_P2"=172, "REG_TXRXBUFF_P2"=173, "REG_IRQ_RAWSTATUS1_P2"=174, "REG_MAC_TXIFSTATUS1"=176, "REG_MAC_TXIFSTATUS2"=177, "REG_IRQ_RAWSTATUS2_P2"=178, "REG_MAC_TXIFRAMPDELAY"=179, "REG_MAC_TXIFRAMPSLOPE"=180, "REG_MAX_TXIFRAMP"=181, "REG_IRQ_STATUS1_P2"=182, "REG_IRQ_STATUS2_P2"=183, "REG_IRQ_AUXSTATUS_P2"=184, "REG_MAC_UNLOCK"=188, "REG_MAC_TXIFFREQ"=190, "REG_WAKEUP_TESTCTRL1"=192, "REG_WAKEUP_RX_EN_CNT"=193, "REG_WAKEUP_TESTENABLES"=194, "REG_WAKEUP_DTBI_CTRL"=195, "REG_WAKEUP_DTBO_CTRL"=196, "REG_WAKEUP_TESTIOBUFTEST"=197, "REG_WAKEUP_WK_RX_TESTCTRL1"=198, "REG_WAKEUP_WK_RX_TESTCTRL2"=199, "REG_WAKEUP_SENS_SEQUENCE_CTRL"=200, "REG_WAKEUP_LNABIAS"=201, "REG_WAKEUP_DET_TH_TRIM1"=202, "REG_WAKEUP_LNABIAS_NOM1"=203, "REG_WAKEUP_RX_TSHORT_TRIM1"=204, "REG_WAKEUP_LNABIAS_NOM2"=205, "REG_WAKEUP_RX_TLONG_TRIM1"=206, "REG_WAKEUP_LNA_NEGRTRIM_NOM1"=207, "REG_WAKEUP_RX_TBURST_TRIM1"=208, "REG_WAKEUP_RX_LNA_NEGRTRIM_NOM2"=209, "REG_WAKEUP_RX_BB_G_BW_SEL1"=210, "REG_WAKEUP_WK_RX_DET_IOSTRIM1"=212, "REG_WAKEUP_WK_RX_CTRL2"=214, "REG_WAKEUP_WK_RX_RSSIVOSTRIM"=215, "REG_WAKEUP_LNANEGR_EFF"=216, "REG_WAKEUP_XOSU_FAST"=217, "REG_WAKEUP_STROSCPWIDTH1"=218, "REG_WAKEUP_STROSCPERIOD1"=220, "REG_WAKEUP_STROSCPERIOD2"=221, "REG_WAKEUP_WK_RX_LNA_NEGRTRIM1"=222, "REG_RF_TXTESTENABLE"=224, "REG_RF_TXIFTESTMODE"=225, "REG_RF_RXTESTENABLE"=226, "REG_RF_RXIFTESTCTRL1"=227, "REG_RF_RXIFTESTCTRL2"=228, "REG_RF_RXIFTESTCTRL3"=229, "REG_RF_SYNTH_TESTCTRL1"=230, "REG_RF_SYNTH_TESTCTRL2"=231, "REG_RF_SYNTH_TESTCTRL3"=232, "REG_RF_ADCTEST1"=237, "REG_RF_ADCTEST2"=238, "REG_RF_TXMIXER_IOSTRIM_LOW_IP"=240, "REG_RF_TXMIXER_IOSTRIM_LOW_IN"=241, "REG_RF_TXMIXER_ISOTRIM_LOW_QP"=242, "REG_RF_TXMIXER_IOSTRIM_LOW_QN"=243, "REG_RF_SYNTH_KPD"=244, "REG_RF_SYNTH_LOLEV"=245, "REG_RF_TXRFPWRTUNEANTSET"=246, "REG_RF_TXPD_GAIN_CTRL"=247, "REG_RF_SYNTH_STARTUP"=248, "REG_RF_TXRFANTTUNE_TXMODE"=249, "REG_RF_TXRFANTTUNE_RXMODE"=250, "REG_RF_RXRFANTTUNE_TXMODE"=251, "REG_RF_RXRFANTTUNE_RXMODE"=252, "REG_ANTMATCH1"=253, "REG_ANTMATCH2"=254, "REG_REVISION_P2"=255] ("Register")
                    # "Apply RSSI Gain Value"
                    # "Address"
                    # "Bitmask"
                    n53 = And(x=w240, y=u8 3 ("Data")) -> (x .and. y?=w244:u16)
                    n54 = call "MICSD Set Register.vi"("Execute on Remote?(F)"=w242, "error in (no error)"=w247, "Data"=w244, "Address"=w245, "VISA Resource Name"=w241) -> ("error out"=w246:errorcluster)  [unwired: 5 in, 1 out]
                  }
                }
              }
              n55 = call "Simple Wait.vi"("mS"=u32 50, "error in"=w161) -> ("error out"=w162:errorcluster)  [unwired: 12 in, 1 out]
              n56 = call "MICSD Set Register.vi"("Execute on Remote?(F)"=w167, "error in (no error)"=w162, "Data"=u8 1, "Address"=w179, "VISA Resource Name"=w168) -> ("error out"=w176:errorcluster, "dup VISA Resource Name"=w173:refnum<visa-resource-name>)  [unwired: 5 in]
              n57 = call "Simple Wait.vi"("mS"=u32 50, "error in"=w176) -> ("error out"=w174:errorcluster)  [unwired: 12 in, 1 out]
              n58 = call "MICSD Set Register.vi"("Execute on Remote?(F)"=w167, "error in (no error)"=w174, "Data"=u8 0, "VISA Resource Name"=w173) -> ("error out"=w172:errorcluster)  [unwired: 6 in, 1 out]
            }
          }
        }
        frame 2 {
          # "Update the CW RF Source Settings"
          n59 = Not Equal?(x="Wakeup Signal Transmit", y=w262) -> (x != y?=w261:bool)
          n60 = case shown="True" w261 {
            tunnel: w260 -> [w280 w287]
            tunnel: w259 -> [w278 w286]
            tunnel: [w280 w284] -> w256
            tunnel: "Wakeup Signal Transmit" -> [_ w285]
            tunnel: w253 -> [_ w283]
            tunnel: w252 -> [w279 _]
            tunnel: [w279 42.0 ("Wakeup Signal Power, dBm")] -> w251
            tunnel: [w278 w281] -> w250
            frame False {
              # "No change to 2.45GHz CW Carrier status, carry on"
            }
            frame True {
              n61 = case shown="False" w285 {
                tunnel: w287 -> [w290 w297]
                tunnel: w286 -> [w288 w293]
                tunnel: [w289 w298] -> w284
                tunnel: w283 -> [_ w295]
                tunnel: [w288 w291] -> w281
                frame False {
                  # "Force Attenuator Update after Reset"
                  # "Disable 2.45GHz CW Carrier"
                  n62 = call "MICSD Abort.vi"("error in (no error)"=w290, "VISA Resource Name"=w288) -> ("error out"=w289:errorcluster)  [unwired: 8 in, 1 out]
                }
                frame True {
                  # "Force Attenuator Update"
                  # "Enable 2.45GHz CW Carrier at 10dBm"
                  n63 = call "MICSD Config.vi"("error in (no error)"=w297, "Function"=enum16{"Write Config", "Read Config"}."Write Config", "MICS_Config_In"=w295, "VISA Resource Name"=w293) -> ("error out"=w296:errorcluster)  [unwired: 5 in, 2 out]
                  n64 = case shown="False" "WakeupMode" {
                    tunnel: [w300 w308] -> w298
                    tunnel: w296 -> [w301 w305]
                    tunnel: w293 -> [w299 w304]
                    tunnel: [w299 w304] -> w291
                    frame False {
                      n65 = call "MICSD Search for Implant.vi"("VISA Resource Name"=w299, "Enable Watchdog?(T)"=FALSE, "error in (no error)"=w301, "Mode"=T2."Start Search") -> ("error out"=w300:errorcluster)  [unwired: 8 in, 3 out]
                    }
                    frame True {
                      w306 = TRUE  # TX Mode (Off)
                      n66 = call "MICSD CW Carrier.vi"("error in (no error)"=w305, "TX Mode (Off)"=w306, "Frequency Range"=enum16{"2.45GHz", "400MHz"}."2.45GHz", "VISA Resource Name"=w304) -> ("error out"=w308:errorcluster)  [unwired: 6 in, 1 out]
                    }
                  }
                }
              }
            }
          }
          n67 = Not Equal?(x="Wakeup Signal Power, dBm", y=w251) -> (x != y?=w258:bool)
          n68 = And(x="Wakeup Signal Transmit", y=w258) -> (x .and. y?=w255:bool)
          n69 = case shown="True" w255 {
            tunnel: w256 -> [w269 w276]
            tunnel: "Wakeup Signal Power, dBm" -> [_ w277]
            tunnel: w250 -> [_ w270]
            tunnel: [w269 w275] -> w249
            frame False {
              # "No update to RF Attenuator value"
            }
            frame True {
              # "RF Attenuator value needs to be updated, do it."
              n70 = Absolute Value(x=w277) -> (abs(x)=w274:dbl)
              n71 = Multiply(x=4.0, y=w274) -> (x*y=w273:dbl)
              n72 = To Unsigned Byte Integer(number=w273) -> (unsigned 8bit integer=w271:u8)
              n73 = call "MICSD Set Attenuator.vi"("error in (no error)"=w276, "Attenuation"=w271, "VISA Resource Name"=w270) -> ("error out"=w275:errorcluster)  [unwired: 7 in, 1 out]
            }
          }
        }
        frame 3 {
          n74 = case shown="True" "Do RSSI" {
            tunnel: w313 -> [w324 w328]
            tunnel: [w324 w331] -> w312
            tunnel: [u8 0 w326] -> w311
            tunnel: w310 -> [_ w330]
            frame False {
              # "RSSI Measurement not enabled"
            }
            frame True {
              # "Perform 2.45GHz RX RSSI Measurement"
              n75 = for {
                N: "Samples to Average" -> [_]
                tunnel: w330 -> [w355]
                tunnel: TRUE -> [w345]
                tunnel: [w348] -> w332 mode=indexing
                shift-right: [w343] -> w331
                shift-left: w328 -> [w354]
                w350 = u16 117 items=["---MANUAL ENTRY---"=1000, "REG_NOREG"=0, "REG_RXBUFF_USED"=1, "REG_RXBUFF_BSIZE"=2, "REG_TXBUFF_USED"=3, "REG_TXBUFF_BSIZE"=4, "REG_TXBUFF_MAXPACKSIZE"=5, "REG_MAC_ERRCLR"=6, "REG_MAC_TRAINNUM"=7, "REG_MAC_SYNCMATCH"=8, "REG_MAC_SYNC1"=9, "REG_MAC_SYNC2"=10, "REG_MAC_SYNC3"=11, "REG_MAC_SYNC4"=12, "REG_MAC_SYNC5"=13, "REG_MAC_MAXBERR"=14, "REG_MAC_ECCORR"=15, "REG_MAC_CRCERR"=16, "REG_MAC_BLKCNT1"=17, "REG_MAC_BLKCNT2"=18, "REG_MAC_IMDTRANSID1"=19, "REG_MAC_IMDTRANSID2"=20, "REG_MAC_IMDTRANSID3"=21, "REG_MAC_COMPANYID"=22, "REG_MAC_MODUSER"=23, "REG_MAC_CHANNEL"=25, "REG_MAC_CLEARWDOG"=26, "REG_MAC_CKCORRTHRESH"=27, "REG_HK_TXADDR"=28, "REG_HK_TXDATA"=29, "REG_HK_TXREPLY"=30, "REG_HK_USERDATA"=31, "REG_HK_USERSTATUS"=32, "REG_HK_LASTADDRESS"=33, "REG_HK_MODE"=34, "REG_MAC_STATUSSEQ"=35, "REG_MAC_MAXRETRIES"=36, "REG_MAC_RESENDTIME"=37, "REG_MAC_POWERSAVETIME"=38, "REG_MAC_HEAD_DET"=39, "REG_MAC_CTRL"=41, "REG_MAC_INITCOM"=42, "REG_INTERFACE_MODE"=43, "REG_TXRXBUFF_BOTH"=44, "REG_TXRXBUFF"=45, "REG_IRQ_RAWSTATUS1"=46, "REG_IRQ_ENABLE1"=47, "REG_IRQ_ENABLESET1"=48, "REG_IRQ_ENABLECLEAR1"=49, "REG_IRQ_RAWSTATUS2"=50, "REG_IRQ_ENABLE2"=51, "REG_IRQ_ENABLESET2"=52, "REG_IRQ_ENABLECLEAR2"=53, "REG_IRQ_STATUS1"=54, "REG_IRQ_STATUS2"=55, "REG_IRQ_AUXSTATUS"=56, "REG_TXBUFF_OVERFLOW"=57, "REG_PO0"=58, "REG_P01"=59, "REG_P02"=60, "REG_P03"=61, "REG_GP0"=62, "REG_GPI"=63, "REG_WAKEUP_245IN"=64, "REG_WAKEUP_COMPANYID"=65, "REG_WAKEUP_IMDTRANSID1"=66, "REG_WAKEUP_IMDTRANSID2"=67, "REG_WAKEUP_IMDTRANSID3"=68, "REG_WAKEUP_CHANNEL"=69, "REG_WAKEUP_MODUSER"=70, "REG_WAKEUP_DEVICEMODE"=71, "REG_WAKEUP_WK_RX_CTRL1"=72, "REG_WAKEUP_STACK_ADDR"=73, "REG_WAKEUP_CTRL"=74, "REG_WAKEUP_STROSCRTRIM"=75, "REG_WAKEUP_BIASTRIM"=76, "REG_WAKEUP_ANT245TUNE"=77, "REG_WAKEUP_WK_RX_RTRIMDET"=78, "REG_WAKEUP_WK_RX_RTRIMDEMOD"=79, "REG_WAKEUP_WK_RX_RSSIGAIN"=80, "REG_WAKEUP_LNAFREQ1"=81, "REG_WAKEUP_STACK"=83, "REG_WAKUP_XOSU"=84, "REG_WAKUP_CNTDROPOUT"=85, "REG_WAKEUP_CRCCTRL"=86, "REG_WAKEUP_CRCWORD1"=87, "REG_WAKEUP_CRCWORD2"=88, "REG_WAKEUP_WK_RX_CTRIM"=89, "REG_WAKEUP_VDDATRIM"=90, "REG_WAKEUP_VDDDTRIM"=91, "REG_WAKEUP_TESTIOBUFEN"=92, "REG_WAKEUP_TESTIOCLAMP"=93, "CORE_RESET_ADDRESS"=94, "CHIP_RESET_ADDRESS"=95, "REG_RF_TXGENCTRL"=96, "REG_RF_TXIFCTRL"=97, "REG_RF_TXRF_SEL_CTRL"=98, "REG_RF_TXRFPWRDEFAULTSET"=99, "REG_RF_RSSITRIM"=100, "REG_RF_TXIFOSCTUNE"=101, "REG_RF_TXIFGAINIMB"=102, "REG_RF_TXIFLOCK"=103, "REG_RF_RXRFLNAGAINTRIM"=104, "REG_RF_RXBIASTR"=105, "REG_RF_RXGENCTRL"=106, "REG_RF_RXIFADCDECLEV"=107, "REG_RF_RXIFDETFILTERTUNE"=108, "REG_RF_RXIFFILTERTUNE"=109, "REG_RF_GENENABLES"=110, "REG_RF_SYNTH_CHANNEL"=111, "REG_TX_RAMP_RTRIM"=112, "REG_TX_RAMP_CTRIM"=113, "REG_RF_XO_TRIM"=114, "REG_RF_SYNTH_SET_TRIM"=115, "REG_RF_ADCCTRL"=116, "REG_RF_ADCOUTPUT"=117, "REG_RF_TXIFAMP"=118, "REG_RF_SYNTH_RTRIM"=119, "REG_RF_SYNTH_CTRIM"=120, "REG_RF_SYNTH_CT"=121, "REG_RF_TXMIXER_IOSTRIM_HIGH_IP"=122, "REG_RF_TXMIXER_IOSTRIM_HIGH_IN"=123, "REG_RF_TXMIXER_IOSTRIM_HIGH_QP"=124, "REG_RF_TXMIXER_IOSTRIM_HIGH_QN"=125, "REG_HX_WUADDR"=126, "REG_REVISION"=127, "REG_NOREG_TEST"=128, "REG_DTEST_RXBUFF"=129, "REG_RXBUFF_NEXT_BLOCK"=130, "REG_RXBUFF_FIRST_IN_PACK"=131, "REG_RXBUFF_FIRST_EMPTY"=132, "REG_MAC_BYPASS"=133, "REG_DTEST_TXBUFF"=134, "REG_TXBUFF_NEXT_BLOCK"=135, "REG_TXBUFF_FIRST_IN_PACK"=136, "REG_TXBUFF_FIRST_EMPTY"=137, "REG_DTEST_SEQ"=138, "REG_DTEST_CKCORR"=139, "REG_MAC_TOPSTATE"=140, "REG_DTEST_INTERFACE"=141, "REG_IFACE_TXRX_BYPASS"=142, "REG_MAC_TXRXWAIT"=143, "REG_MAC_TXRFRAMP"=144, "REG_MAC_TRAINWORD"=145, "REG_MAC_TRAINWORD2"=146, "REG_MAC_SETTINGS"=147, "REG_MAC_CALSELECT1"=148, "REG_MAC_CALSELECT2"=149, "REG_MAC_ANTMATCHSEL"=150, "REG_MAC_ANTTUNESEL1"=151, "REG_MAC_ANTTUNESEL2"=152, "REG_MAC_ANTTUNESEL3"=153, "REG_MAC_ANTTUNESTEP"=154, "REG_MAC_WUMODEBURST"=156, "REG_MAC_WUOFFSHORT"=157, "REG_MAC_WUOFFLONG"=158, "REG_MAC_CLKRECCTRL"=159, "REG_HK_MODE_P2"=162, "REG_MAC_ANTTUNERES1"=164, "REG_MAC_ANTTUNERES2"=165, "REG_INTERFACE_MODE_TEST"=171, "REG_TXRXBUFF_BOTH_P2"=172, "REG_TXRXBUFF_P2"=173, "REG_IRQ_RAWSTATUS1_P2"=174, "REG_MAC_TXIFSTATUS1"=176, "REG_MAC_TXIFSTATUS2"=177, "REG_IRQ_RAWSTATUS2_P2"=178, "REG_MAC_TXIFRAMPDELAY"=179, "REG_MAC_TXIFRAMPSLOPE"=180, "REG_MAX_TXIFRAMP"=181, "REG_IRQ_STATUS1_P2"=182, "REG_IRQ_STATUS2_P2"=183, "REG_IRQ_AUXSTATUS_P2"=184, "REG_MAC_UNLOCK"=188, "REG_MAC_TXIFFREQ"=190, "REG_WAKEUP_TESTCTRL1"=192, "REG_WAKEUP_RX_EN_CNT"=193, "REG_WAKEUP_TESTENABLES"=194, "REG_WAKEUP_DTBI_CTRL"=195, "REG_WAKEUP_DTBO_CTRL"=196, "REG_WAKEUP_TESTIOBUFTEST"=197, "REG_WAKEUP_WK_RX_TESTCTRL1"=198, "REG_WAKEUP_WK_RX_TESTCTRL2"=199, "REG_WAKEUP_SENS_SEQUENCE_CTRL"=200, "REG_WAKEUP_LNABIAS"=201, "REG_WAKEUP_DET_TH_TRIM1"=202, "REG_WAKEUP_LNABIAS_NOM1"=203, "REG_WAKEUP_RX_TSHORT_TRIM1"=204, "REG_WAKEUP_LNABIAS_NOM2"=205, "REG_WAKEUP_RX_TLONG_TRIM1"=206, "REG_WAKEUP_LNA_NEGRTRIM_NOM1"=207, "REG_WAKEUP_RX_TBURST_TRIM1"=208, "REG_WAKEUP_RX_LNA_NEGRTRIM_NOM2"=209, "REG_WAKEUP_RX_BB_G_BW_SEL1"=210, "REG_WAKEUP_WK_RX_DET_IOSTRIM1"=212, "REG_WAKEUP_WK_RX_CTRL2"=214, "REG_WAKEUP_WK_RX_RSSIVOSTRIM"=215, "REG_WAKEUP_LNANEGR_EFF"=216, "REG_WAKEUP_XOSU_FAST"=217, "REG_WAKEUP_STROSCPWIDTH1"=218, "REG_WAKEUP_STROSCPERIOD1"=220, "REG_WAKEUP_STROSCPERIOD2"=221, "REG_WAKEUP_WK_RX_LNA_NEGRTRIM1"=222, "REG_RF_TXTESTENABLE"=224, "REG_RF_TXIFTESTMODE"=225, "REG_RF_RXTESTENABLE"=226, "REG_RF_RXIFTESTCTRL1"=227, "REG_RF_RXIFTESTCTRL2"=228, "REG_RF_RXIFTESTCTRL3"=229, "REG_RF_SYNTH_TESTCTRL1"=230, "REG_RF_SYNTH_TESTCTRL2"=231, "REG_RF_SYNTH_TESTCTRL3"=232, "REG_RF_ADCTEST1"=237, "REG_RF_ADCTEST2"=238, "REG_RF_TXMIXER_IOSTRIM_LOW_IP"=240, "REG_RF_TXMIXER_IOSTRIM_LOW_IN"=241, "REG_RF_TXMIXER_ISOTRIM_LOW_QP"=242, "REG_RF_TXMIXER_IOSTRIM_LOW_QN"=243, "REG_RF_SYNTH_KPD"=244, "REG_RF_SYNTH_LOLEV"=245, "REG_RF_TXRFPWRTUNEANTSET"=246, "REG_RF_TXPD_GAIN_CTRL"=247, "REG_RF_SYNTH_STARTUP"=248, "REG_RF_TXRFANTTUNE_TXMODE"=249, "REG_RF_TXRFANTTUNE_RXMODE"=250, "REG_RF_RXRFANTTUNE_TXMODE"=251, "REG_RF_RXRFANTTUNE_RXMODE"=252, "REG_ANTMATCH1"=253, "REG_ANTMATCH2"=254, "REG_REVISION_P2"=255] ("Register")
                w352 = u16 116 items=["---MANUAL ENTRY---"=1000, "REG_NOREG"=0, "REG_RXBUFF_USED"=1, "REG_RXBUFF_BSIZE"=2, "REG_TXBUFF_USED"=3, "REG_TXBUFF_BSIZE"=4, "REG_TXBUFF_MAXPACKSIZE"=5, "REG_MAC_ERRCLR"=6, "REG_MAC_TRAINNUM"=7, "REG_MAC_SYNCMATCH"=8, "REG_MAC_SYNC1"=9, "REG_MAC_SYNC2"=10, "REG_MAC_SYNC3"=11, "REG_MAC_SYNC4"=12, "REG_MAC_SYNC5"=13, "REG_MAC_MAXBERR"=14, "REG_MAC_ECCORR"=15, "REG_MAC_CRCERR"=16, "REG_MAC_BLKCNT1"=17, "REG_MAC_BLKCNT2"=18, "REG_MAC_IMDTRANSID1"=19, "REG_MAC_IMDTRANSID2"=20, "REG_MAC_IMDTRANSID3"=21, "REG_MAC_COMPANYID"=22, "REG_MAC_MODUSER"=23, "REG_MAC_CHANNEL"=25, "REG_MAC_CLEARWDOG"=26, "REG_MAC_CKCORRTHRESH"=27, "REG_HK_TXADDR"=28, "REG_HK_TXDATA"=29, "REG_HK_TXREPLY"=30, "REG_HK_USERDATA"=31, "REG_HK_USERSTATUS"=32, "REG_HK_LASTADDRESS"=33, "REG_HK_MODE"=34, "REG_MAC_STATUSSEQ"=35, "REG_MAC_MAXRETRIES"=36, "REG_MAC_RESENDTIME"=37, "REG_MAC_POWERSAVETIME"=38, "REG_MAC_HEAD_DET"=39, "REG_MAC_CTRL"=41, "REG_MAC_INITCOM"=42, "REG_INTERFACE_MODE"=43, "REG_TXRXBUFF_BOTH"=44, "REG_TXRXBUFF"=45, "REG_IRQ_RAWSTATUS1"=46, "REG_IRQ_ENABLE1"=47, "REG_IRQ_ENABLESET1"=48, "REG_IRQ_ENABLECLEAR1"=49, "REG_IRQ_RAWSTATUS2"=50, "REG_IRQ_ENABLE2"=51, "REG_IRQ_ENABLESET2"=52, "REG_IRQ_ENABLECLEAR2"=53, "REG_IRQ_STATUS1"=54, "REG_IRQ_STATUS2"=55, "REG_IRQ_AUXSTATUS"=56, "REG_TXBUFF_OVERFLOW"=57, "REG_PO0"=58, "REG_P01"=59, "REG_P02"=60, "REG_P03"=61, "REG_GP0"=62, "REG_GPI"=63, "REG_WAKEUP_245IN"=64, "REG_WAKEUP_COMPANYID"=65, "REG_WAKEUP_IMDTRANSID1"=66, "REG_WAKEUP_IMDTRANSID2"=67, "REG_WAKEUP_IMDTRANSID3"=68, "REG_WAKEUP_CHANNEL"=69, "REG_WAKEUP_MODUSER"=70, "REG_WAKEUP_DEVICEMODE"=71, "REG_WAKEUP_WK_RX_CTRL1"=72, "REG_WAKEUP_STACK_ADDR"=73, "REG_WAKEUP_CTRL"=74, "REG_WAKEUP_STROSCRTRIM"=75, "REG_WAKEUP_BIASTRIM"=76, "REG_WAKEUP_ANT245TUNE"=77, "REG_WAKEUP_WK_RX_RTRIMDET"=78, "REG_WAKEUP_WK_RX_RTRIMDEMOD"=79, "REG_WAKEUP_WK_RX_RSSIGAIN"=80, "REG_WAKEUP_LNAFREQ1"=81, "REG_WAKEUP_STACK"=83, "REG_WAKUP_XOSU"=84, "REG_WAKUP_CNTDROPOUT"=85, "REG_WAKEUP_CRCCTRL"=86, "REG_WAKEUP_CRCWORD1"=87, "REG_WAKEUP_CRCWORD2"=88, "REG_WAKEUP_WK_RX_CTRIM"=89, "REG_WAKEUP_VDDATRIM"=90, "REG_WAKEUP_VDDDTRIM"=91, "REG_WAKEUP_TESTIOBUFEN"=92, "REG_WAKEUP_TESTIOCLAMP"=93, "CORE_RESET_ADDRESS"=94, "CHIP_RESET_ADDRESS"=95, "REG_RF_TXGENCTRL"=96, "REG_RF_TXIFCTRL"=97, "REG_RF_TXRF_SEL_CTRL"=98, "REG_RF_TXRFPWRDEFAULTSET"=99, "REG_RF_RSSITRIM"=100, "REG_RF_TXIFOSCTUNE"=101, "REG_RF_TXIFGAINIMB"=102, "REG_RF_TXIFLOCK"=103, "REG_RF_RXRFLNAGAINTRIM"=104, "REG_RF_RXBIASTR"=105, "REG_RF_RXGENCTRL"=106, "REG_RF_RXIFADCDECLEV"=107, "REG_RF_RXIFDETFILTERTUNE"=108, "REG_RF_RXIFFILTERTUNE"=109, "REG_RF_GENENABLES"=110, "REG_RF_SYNTH_CHANNEL"=111, "REG_TX_RAMP_RTRIM"=112, "REG_TX_RAMP_CTRIM"=113, "REG_RF_XO_TRIM"=114, "REG_RF_SYNTH_SET_TRIM"=115, "REG_RF_ADCCTRL"=116, "REG_RF_ADCOUTPUT"=117, "REG_RF_TXIFAMP"=118, "REG_RF_SYNTH_RTRIM"=119, "REG_RF_SYNTH_CTRIM"=120, "REG_RF_SYNTH_CT"=121, "REG_RF_TXMIXER_IOSTRIM_HIGH_IP"=122, "REG_RF_TXMIXER_IOSTRIM_HIGH_IN"=123, "REG_RF_TXMIXER_IOSTRIM_HIGH_QP"=124, "REG_RF_TXMIXER_IOSTRIM_HIGH_QN"=125, "REG_HX_WUADDR"=126, "REG_REVISION"=127, "REG_NOREG_TEST"=128, "REG_DTEST_RXBUFF"=129, "REG_RXBUFF_NEXT_BLOCK"=130, "REG_RXBUFF_FIRST_IN_PACK"=131, "REG_RXBUFF_FIRST_EMPTY"=132, "REG_MAC_BYPASS"=133, "REG_DTEST_TXBUFF"=134, "REG_TXBUFF_NEXT_BLOCK"=135, "REG_TXBUFF_FIRST_IN_PACK"=136, "REG_TXBUFF_FIRST_EMPTY"=137, "REG_DTEST_SEQ"=138, "REG_DTEST_CKCORR"=139, "REG_MAC_TOPSTATE"=140, "REG_DTEST_INTERFACE"=141, "REG_IFACE_TXRX_BYPASS"=142, "REG_MAC_TXRXWAIT"=143, "REG_MAC_TXRFRAMP"=144, "REG_MAC_TRAINWORD"=145, "REG_MAC_TRAINWORD2"=146, "REG_MAC_SETTINGS"=147, "REG_MAC_CALSELECT1"=148, "REG_MAC_CALSELECT2"=149, "REG_MAC_ANTMATCHSEL"=150, "REG_MAC_ANTTUNESEL1"=151, "REG_MAC_ANTTUNESEL2"=152, "REG_MAC_ANTTUNESEL3"=153, "REG_MAC_ANTTUNESTEP"=154, "REG_MAC_WUMODEBURST"=156, "REG_MAC_WUOFFSHORT"=157, "REG_MAC_WUOFFLONG"=158, "REG_MAC_CLKRECCTRL"=159, "REG_HK_MODE_P2"=162, "REG_MAC_ANTTUNERES1"=164, "REG_MAC_ANTTUNERES2"=165, "REG_INTERFACE_MODE_TEST"=171, "REG_TXRXBUFF_BOTH_P2"=172, "REG_TXRXBUFF_P2"=173, "REG_IRQ_RAWSTATUS1_P2"=174, "REG_MAC_TXIFSTATUS1"=176, "REG_MAC_TXIFSTATUS2"=177, "REG_IRQ_RAWSTATUS2_P2"=178, "REG_MAC_TXIFRAMPDELAY"=179, "REG_MAC_TXIFRAMPSLOPE"=180, "REG_MAX_TXIFRAMP"=181, "REG_IRQ_STATUS1_P2"=182, "REG_IRQ_STATUS2_P2"=183, "REG_IRQ_AUXSTATUS_P2"=184, "REG_MAC_UNLOCK"=188, "REG_MAC_TXIFFREQ"=190, "REG_WAKEUP_TESTCTRL1"=192, "REG_WAKEUP_RX_EN_CNT"=193, "REG_WAKEUP_TESTENABLES"=194, "REG_WAKEUP_DTBI_CTRL"=195, "REG_WAKEUP_DTBO_CTRL"=196, "REG_WAKEUP_TESTIOBUFTEST"=197, "REG_WAKEUP_WK_RX_TESTCTRL1"=198, "REG_WAKEUP_WK_RX_TESTCTRL2"=199, "REG_WAKEUP_SENS_SEQUENCE_CTRL"=200, "REG_WAKEUP_LNABIAS"=201, "REG_WAKEUP_DET_TH_TRIM1"=202, "REG_WAKEUP_LNABIAS_NOM1"=203, "REG_WAKEUP_RX_TSHORT_TRIM1"=204, "REG_WAKEUP_LNABIAS_NOM2"=205, "REG_WAKEUP_RX_TLONG_TRIM1"=206, "REG_WAKEUP_LNA_NEGRTRIM_NOM1"=207, "REG_WAKEUP_RX_TBURST_TRIM1"=208, "REG_WAKEUP_RX_LNA_NEGRTRIM_NOM2"=209, "REG_WAKEUP_RX_BB_G_BW_SEL1"=210, "REG_WAKEUP_WK_RX_DET_IOSTRIM1"=212, "REG_WAKEUP_WK_RX_CTRL2"=214, "REG_WAKEUP_WK_RX_RSSIVOSTRIM"=215, "REG_WAKEUP_LNANEGR_EFF"=216, "REG_WAKEUP_XOSU_FAST"=217, "REG_WAKEUP_STROSCPWIDTH1"=218, "REG_WAKEUP_STROSCPERIOD1"=220, "REG_WAKEUP_STROSCPERIOD2"=221, "REG_WAKEUP_WK_RX_LNA_NEGRTRIM1"=222, "REG_RF_TXTESTENABLE"=224, "REG_RF_TXIFTESTMODE"=225, "REG_RF_RXTESTENABLE"=226, "REG_RF_RXIFTESTCTRL1"=227, "REG_RF_RXIFTESTCTRL2"=228, "REG_RF_RXIFTESTCTRL3"=229, "REG_RF_SYNTH_TESTCTRL1"=230, "REG_RF_SYNTH_TESTCTRL2"=231, "REG_RF_SYNTH_TESTCTRL3"=232, "REG_RF_ADCTEST1"=237, "REG_RF_ADCTEST2"=238, "REG_RF_TXMIXER_IOSTRIM_LOW_IP"=240, "REG_RF_TXMIXER_IOSTRIM_LOW_IN"=241, "REG_RF_TXMIXER_ISOTRIM_LOW_QP"=242, "REG_RF_TXMIXER_IOSTRIM_LOW_QN"=243, "REG_RF_SYNTH_KPD"=244, "REG_RF_SYNTH_LOLEV"=245, "REG_RF_TXRFPWRTUNEANTSET"=246, "REG_RF_TXPD_GAIN_CTRL"=247, "REG_RF_SYNTH_STARTUP"=248, "REG_RF_TXRFANTTUNE_TXMODE"=249, "REG_RF_TXRFANTTUNE_RXMODE"=250, "REG_RF_RXRFANTTUNE_TXMODE"=251, "REG_RF_RXRFANTTUNE_RXMODE"=252, "REG_ANTMATCH1"=253, "REG_ANTMATCH2"=254, "REG_REVISION_P2"=255] ("Register")
                n76 = call "MICSD Set Register.vi"("Execute on Remote?(F)"=w345, "error in (no error)"=w354, "Data"=u8 29, "Address"=w352, "VISA Resource Name"=w355) -> ("error out"=w356:errorcluster, "dup VISA Resource Name"=w357:refnum<visa-resource-name>)  [unwired: 5 in]
                n77 = call "MICSD Set Register.vi"("Execute on Remote?(F)"=w345, "error in (no error)"=w356, "Data"=u8 31, "Address"=w352, "VISA Resource Name"=w357) -> ("error out"=w344:errorcluster, "dup VISA Resource Name"=w351:refnum<visa-resource-name>)  [unwired: 5 in]
                n78 = call "Simple Wait.vi"("mS"=u32 5, "error in"=w344) -> ("error out"=w342:errorcluster)  [unwired: 12 in, 1 out]
                n79 = while {
                  tunnel: w351 -> [w369]
                  tunnel: w350 -> [w368]
                  tunnel: [w364] -> w349
                  tunnel: w345 -> [w367]
                  tunnel: [w366] -> w343
                  tunnel: w342 -> [w365]
                  i -> [w361]
                  stop <- w362 stop-if-true
                  w360 = u8 31 ("y")
                  n80 = call "MICSD Get Register.vi"("Execute on Remote?(F)"=w367, "error in (no error)"=w365, "Address"=w368, "VISA Resource Name"=w369) -> ("error out"=w366:errorcluster, "Data"=w364:u8)  [unwired: 5 in, 1 out]
                  n81 = Greater?(x=w361, y=w360) -> (0:w359:bool)
                  n82 = Greater?(x=w364, y=w360) -> (0:w363:bool)
                  n83 = Or(x=w359, y=w363) -> (x .or. y?=w362:bool)
                }
                n84 = To Long Integer(number=w349) -> (32bit integer=w346:i32)
                n85 = Subtract(x=w346, y=32) -> (x-y=w348:i32)
              }
              n86 = local read "WakeupMode"() -> (w325:bool)
              n87 = case shown="False" w325 {
                tunnel: w332 -> [w335 w340]
                tunnel: "Samples to Average" -> [_ w338]
                tunnel: [w334 w336] -> w326
                frame False {
                  n88 = call "RSSI Peak Averaging.vi"("Reject Ratio, % (75)"="Reject Ratio, %", "Raw RSSI Data"=w335) -> ("Averaged Peak RSSI"=w334:u8)  [unwired: 9 in]
                }
                frame True {
                  n89 = Add Array Elements(numeric array=w340) -> (sum=w339:i32)
                  n90 = Quotient & Remainder(x=w339, y=w338) -> (floor(x/y)=w337:i32)  [unwired: 1 out]
                  n91 = To Unsigned Byte Integer(number=w337) -> (unsigned 8bit integer=w336:u8)
                }
              }
            }
          }
          "RSSI Reading" <- w311
        }
        frame 4 {
          n92 = Format Into String(format string="Address=0x0051 {LNA Freq Trim}\r\nData=0x%02x\r\nAddress=0x00DE {LNA Gain Trim}\r\nData=0x%02x\r\nAddress=0x004D {2.45 Antenna Tune}\r\nData=0x%02x\r\nAddress=0x00D7 {RSSI Fine Trim}\r\nData=0x%02x\r\nAddress 0x00D4 {Detector Offset Trim}\r\nData=0x%02x", w376, w375, w374, w371, w373) -> (resulting string=→"Trim Settings":string)  [unwired: 2 in, 1 out]
        }
        frame 5 {
          n93 = case shown="True" "Loopback Detector" {
            tunnel: w386 -> [w395 w404]
            tunnel: w385 -> [_ w399]
            tunnel: [w395 w402] -> w384
            frame False {
            }
            frame True {
              w398 = TRUE
              (unwired) u8 0 ("Data")
              w401 = u16 85 items=["---MANUAL ENTRY---"=1000, "REG_NOREG"=0, "REG_RXBUFF_USED"=1, "REG_RXBUFF_BSIZE"=2, "REG_TXBUFF_USED"=3, "REG_TXBUFF_BSIZE"=4, "REG_TXBUFF_MAXPACKSIZE"=5, "REG_MAC_ERRCLR"=6, "REG_MAC_TRAINNUM"=7, "REG_MAC_SYNCMATCH"=8, "REG_MAC_SYNC1"=9, "REG_MAC_SYNC2"=10, "REG_MAC_SYNC3"=11, "REG_MAC_SYNC4"=12, "REG_MAC_SYNC5"=13, "REG_MAC_MAXBERR"=14, "REG_MAC_ECCORR"=15, "REG_MAC_CRCERR"=16, "REG_MAC_BLKCNT1"=17, "REG_MAC_BLKCNT2"=18, "REG_MAC_IMDTRANSID1"=19, "REG_MAC_IMDTRANSID2"=20, "REG_MAC_IMDTRANSID3"=21, "REG_MAC_COMPANYID"=22, "REG_MAC_MODUSER"=23, "REG_MAC_CHANNEL"=25, "REG_MAC_CLEARWDOG"=26, "REG_MAC_CKCORRTHRESH"=27, "REG_HK_TXADDR"=28, "REG_HK_TXDATA"=29, "REG_HK_TXREPLY"=30, "REG_HK_USERDATA"=31, "REG_HK_USERSTATUS"=32, "REG_HK_LASTADDRESS"=33, "REG_HK_MODE"=34, "REG_MAC_STATUSSEQ"=35, "REG_MAC_MAXRETRIES"=36, "REG_MAC_RESENDTIME"=37, "REG_MAC_POWERSAVETIME"=38, "REG_MAC_HEAD_DET"=39, "REG_MAC_CTRL"=41, "REG_MAC_INITCOM"=42, "REG_INTERFACE_MODE"=43, "REG_TXRXBUFF_BOTH"=44, "REG_TXRXBUFF"=45, "REG_IRQ_RAWSTATUS1"=46, "REG_IRQ_ENABLE1"=47, "REG_IRQ_ENABLESET1"=48, "REG_IRQ_ENABLECLEAR1"=49, "REG_IRQ_RAWSTATUS2"=50, "REG_IRQ_ENABLE2"=51, "REG_IRQ_ENABLESET2"=52, "REG_IRQ_ENABLECLEAR2"=53, "REG_IRQ_STATUS1"=54, "REG_IRQ_STATUS2"=55, "REG_IRQ_AUXSTATUS"=56, "REG_TXBUFF_OVERFLOW"=57, "REG_PO0"=58, "REG_P01"=59, "REG_P02"=60, "REG_P03"=61, "REG_GP0"=62, "REG_GPI"=63, "REG_WAKEUP_245IN"=64, "REG_WAKEUP_COMPANYID"=65, "REG_WAKEUP_IMDTRANSID1"=66, "REG_WAKEUP_IMDTRANSID2"=67, "REG_WAKEUP_IMDTRANSID3"=68, "REG_WAKEUP_CHANNEL"=69, "REG_WAKEUP_MODUSER"=70, "REG_WAKEUP_DEVICEMODE"=71, "REG_WAKEUP_WK_RX_CTRL1"=72, "REG_WAKEUP_STACK_ADDR"=73, "REG_WAKEUP_CTRL"=74, "REG_WAKEUP_STROSCRTRIM"=75, "REG_WAKEUP_BIASTRIM"=76, "REG_WAKEUP_ANT245TUNE"=77, "REG_WAKEUP_WK_RX_RTRIMDET"=78, "REG_WAKEUP_WK_RX_RTRIMDEMOD"=79, "REG_WAKEUP_WK_RX_RSSIGAIN"=80, "REG_WAKEUP_LNAFREQ1"=81, "REG_WAKEUP_STACK"=83, "REG_WAKUP_XOSU"=84, "REG_WAKUP_CNTDROPOUT"=85, "REG_WAKEUP_CRCCTRL"=86, "REG_WAKEUP_CRCWORD1"=87, "REG_WAKEUP_CRCWORD2"=88, "REG_WAKEUP_WK_RX_CTRIM"=89, "REG_WAKEUP_VDDATRIM"=90, "REG_WAKEUP_VDDDTRIM"=91, "REG_WAKEUP_TESTIOBUFEN"=92, "REG_WAKEUP_TESTIOCLAMP"=93, "CORE_RESET_ADDRESS"=94, "CHIP_RESET_ADDRESS"=95, "REG_RF_TXGENCTRL"=96, "REG_RF_TXIFCTRL"=97, "REG_RF_TXRF_SEL_CTRL"=98, "REG_RF_TXRFPWRDEFAULTSET"=99, "REG_RF_RSSITRIM"=100, "REG_RF_TXIFOSCTUNE"=101, "REG_RF_TXIFGAINIMB"=102, "REG_RF_TXIFLOCK"=103, "REG_RF_RXRFLNAGAINTRIM"=104, "REG_RF_RXBIASTR"=105, "REG_RF_RXGENCTRL"=106, "REG_RF_RXIFADCDECLEV"=107, "REG_RF_RXIFDETFILTERTUNE"=108, "REG_RF_RXIFFILTERTUNE"=109, "REG_RF_GENENABLES"=110, "REG_RF_SYNTH_CHANNEL"=111, "REG_TX_RAMP_RTRIM"=112, "REG_TX_RAMP_CTRIM"=113, "REG_RF_XO_TRIM"=114, "REG_RF_SYNTH_SET_TRIM"=115, "REG_RF_ADCCTRL"=116, "REG_RF_ADCOUTPUT"=117, "REG_RF_TXIFAMP"=118, "REG_RF_SYNTH_RTRIM"=119, "REG_RF_SYNTH_CTRIM"=120, "REG_RF_SYNTH_CT"=121, "REG_RF_TXMIXER_IOSTRIM_HIGH_IP"=122, "REG_RF_TXMIXER_IOSTRIM_HIGH_IN"=123, "REG_RF_TXMIXER_IOSTRIM_HIGH_QP"=124, "REG_RF_TXMIXER_IOSTRIM_HIGH_QN"=125, "REG_HX_WUADDR"=126, "REG_REVISION"=127, "REG_NOREG_TEST"=128, "REG_DTEST_RXBUFF"=129, "REG_RXBUFF_NEXT_BLOCK"=130, "REG_RXBUFF_FIRST_IN_PACK"=131, "REG_RXBUFF_FIRST_EMPTY"=132, "REG_MAC_BYPASS"=133, "REG_DTEST_TXBUFF"=134, "REG_TXBUFF_NEXT_BLOCK"=135, "REG_TXBUFF_FIRST_IN_PACK"=136, "REG_TXBUFF_FIRST_EMPTY"=137, "REG_DTEST_SEQ"=138, "REG_DTEST_CKCORR"=139, "REG_MAC_TOPSTATE"=140, "REG_DTEST_INTERFACE"=141, "REG_IFACE_TXRX_BYPASS"=142, "REG_MAC_TXRXWAIT"=143, "REG_MAC_TXRFRAMP"=144, "REG_MAC_TRAINWORD"=145, "REG_MAC_TRAINWORD2"=146, "REG_MAC_SETTINGS"=147, "REG_MAC_CALSELECT1"=148, "REG_MAC_CALSELECT2"=149, "REG_MAC_ANTMATCHSEL"=150, "REG_MAC_ANTTUNESEL1"=151, "REG_MAC_ANTTUNESEL2"=152, "REG_MAC_ANTTUNESEL3"=153, "REG_MAC_ANTTUNESTEP"=154, "REG_MAC_WUMODEBURST"=156, "REG_MAC_WUOFFSHORT"=157, "REG_MAC_WUOFFLONG"=158, "REG_MAC_CLKRECCTRL"=159, "REG_HK_MODE_P2"=162, "REG_MAC_ANTTUNERES1"=164, "REG_MAC_ANTTUNERES2"=165, "REG_INTERFACE_MODE_TEST"=171, "REG_TXRXBUFF_BOTH_P2"=172, "REG_TXRXBUFF_P2"=173, "REG_IRQ_RAWSTATUS1_P2"=174, "REG_MAC_TXIFSTATUS1"=176, "REG_MAC_TXIFSTATUS2"=177, "REG_IRQ_RAWSTATUS2_P2"=178, "REG_MAC_TXIFRAMPDELAY"=179, "REG_MAC_TXIFRAMPSLOPE"=180, "REG_MAX_TXIFRAMP"=181, "REG_IRQ_STATUS1_P2"=182, "REG_IRQ_STATUS2_P2"=183, "REG_IRQ_AUXSTATUS_P2"=184, "REG_MAC_UNLOCK"=188, "REG_MAC_TXIFFREQ"=190, "REG_WAKEUP_TESTCTRL1"=192, "REG_WAKEUP_RX_EN_CNT"=193, "REG_WAKEUP_TESTENABLES"=194, "REG_WAKEUP_DTBI_CTRL"=195, "REG_WAKEUP_DTBO_CTRL"=196, "REG_WAKEUP_TESTIOBUFTEST"=197, "REG_WAKEUP_WK_RX_TESTCTRL1"=198, "REG_WAKEUP_WK_RX_TESTCTRL2"=199, "REG_WAKEUP_SENS_SEQUENCE_CTRL"=200, "REG_WAKEUP_LNABIAS"=201, "REG_WAKEUP_DET_TH_TRIM1"=202, "REG_WAKEUP_LNABIAS_NOM1"=203, "REG_WAKEUP_RX_TSHORT_TRIM1"=204, "REG_WAKEUP_LNABIAS_NOM2"=205, "REG_WAKEUP_RX_TLONG_TRIM1"=206, "REG_WAKEUP_LNA_NEGRTRIM_NOM1"=207, "REG_WAKEUP_RX_TBURST_TRIM1"=208, "REG_WAKEUP_RX_LNA_NEGRTRIM_NOM2"=209, "REG_WAKEUP_RX_BB_G_BW_SEL1"=210, "REG_WAKEUP_WK_RX_DET_IOSTRIM1"=212, "REG_WAKEUP_WK_RX_CTRL2"=214, "REG_WAKEUP_WK_RX_RSSIVOSTRIM"=215, "REG_WAKEUP_LNANEGR_EFF"=216, "REG_WAKEUP_XOSU_FAST"=217, "REG_WAKEUP_STROSCPWIDTH1"=218, "REG_WAKEUP_STROSCPERIOD1"=220, "REG_WAKEUP_STROSCPERIOD2"=221, "REG_WAKEUP_WK_RX_LNA_NEGRTRIM1"=222, "REG_RF_TXTESTENABLE"=224, "REG_RF_TXIFTESTMODE"=225, "REG_RF_RXTESTENABLE"=226, "REG_RF_RXIFTESTCTRL1"=227, "REG_RF_RXIFTESTCTRL2"=228, "REG_RF_RXIFTESTCTRL3"=229, "REG_RF_SYNTH_TESTCTRL1"=230, "REG_RF_SYNTH_TESTCTRL2"=231, "REG_RF_SYNTH_TESTCTRL3"=232, "REG_RF_ADCTEST1"=237, "REG_RF_ADCTEST2"=238, "REG_RF_TXMIXER_IOSTRIM_LOW_IP"=240, "REG_RF_TXMIXER_IOSTRIM_LOW_IN"=241, "REG_RF_TXMIXER_ISOTRIM_LOW_QP"=242, "REG_RF_TXMIXER_IOSTRIM_LOW_QN"=243, "REG_RF_SYNTH_KPD"=244, "REG_RF_SYNTH_LOLEV"=245, "REG_RF_TXRFPWRTUNEANTSET"=246, "REG_RF_TXPD_GAIN_CTRL"=247, "REG_RF_SYNTH_STARTUP"=248, "REG_RF_TXRFANTTUNE_TXMODE"=249, "REG_RF_TXRFANTTUNE_RXMODE"=250, "REG_RF_RXRFANTTUNE_TXMODE"=251, "REG_RF_RXRFANTTUNE_RXMODE"=252, "REG_ANTMATCH1"=253, "REG_ANTMATCH2"=254, "REG_REVISION_P2"=255] ("Register")
              w400 = u16 64 items=["---MANUAL ENTRY---"=1000, "REG_NOREG"=0, "REG_RXBUFF_USED"=1, "REG_RXBUFF_BSIZE"=2, "REG_TXBUFF_USED"=3, "REG_TXBUFF_BSIZE"=4, "REG_TXBUFF_MAXPACKSIZE"=5, "REG_MAC_ERRCLR"=6, "REG_MAC_TRAINNUM"=7, "REG_MAC_SYNCMATCH"=8, "REG_MAC_SYNC1"=9, "REG_MAC_SYNC2"=10, "REG_MAC_SYNC3"=11, "REG_MAC_SYNC4"=12, "REG_MAC_SYNC5"=13, "REG_MAC_MAXBERR"=14, "REG_MAC_ECCORR"=15, "REG_MAC_CRCERR"=16, "REG_MAC_BLKCNT1"=17, "REG_MAC_BLKCNT2"=18, "REG_MAC_IMDTRANSID1"=19, "REG_MAC_IMDTRANSID2"=20, "REG_MAC_IMDTRANSID3"=21, "REG_MAC_COMPANYID"=22, "REG_MAC_MODUSER"=23, "REG_MAC_CHANNEL"=25, "REG_MAC_CLEARWDOG"=26, "REG_MAC_CKCORRTHRESH"=27, "REG_HK_TXADDR"=28, "REG_HK_TXDATA"=29, "REG_HK_TXREPLY"=30, "REG_HK_USERDATA"=31, "REG_HK_USERSTATUS"=32, "REG_HK_LASTADDRESS"=33, "REG_HK_MODE"=34, "REG_MAC_STATUSSEQ"=35, "REG_MAC_MAXRETRIES"=36, "REG_MAC_RESENDTIME"=37, "REG_MAC_POWERSAVETIME"=38, "REG_MAC_HEAD_DET"=39, "REG_MAC_CTRL"=41, "REG_MAC_INITCOM"=42, "REG_INTERFACE_MODE"=43, "REG_TXRXBUFF_BOTH"=44, "REG_TXRXBUFF"=45, "REG_IRQ_RAWSTATUS1"=46, "REG_IRQ_ENABLE1"=47, "REG_IRQ_ENABLESET1"=48, "REG_IRQ_ENABLECLEAR1"=49, "REG_IRQ_RAWSTATUS2"=50, "REG_IRQ_ENABLE2"=51, "REG_IRQ_ENABLESET2"=52, "REG_IRQ_ENABLECLEAR2"=53, "REG_IRQ_STATUS1"=54, "REG_IRQ_STATUS2"=55, "REG_IRQ_AUXSTATUS"=56, "REG_TXBUFF_OVERFLOW"=57, "REG_PO0"=58, "REG_P01"=59, "REG_P02"=60, "REG_P03"=61, "REG_GP0"=62, "REG_GPI"=63, "REG_WAKEUP_245IN"=64, "REG_WAKEUP_COMPANYID"=65, "REG_WAKEUP_IMDTRANSID1"=66, "REG_WAKEUP_IMDTRANSID2"=67, "REG_WAKEUP_IMDTRANSID3"=68, "REG_WAKEUP_CHANNEL"=69, "REG_WAKEUP_MODUSER"=70, "REG_WAKEUP_DEVICEMODE"=71, "REG_WAKEUP_WK_RX_CTRL1"=72, "REG_WAKEUP_STACK_ADDR"=73, "REG_WAKEUP_CTRL"=74, "REG_WAKEUP_STROSCRTRIM"=75, "REG_WAKEUP_BIASTRIM"=76, "REG_WAKEUP_ANT245TUNE"=77, "REG_WAKEUP_WK_RX_RTRIMDET"=78, "REG_WAKEUP_WK_RX_RTRIMDEMOD"=79, "REG_WAKEUP_WK_RX_RSSIGAIN"=80, "REG_WAKEUP_LNAFREQ1"=81, "REG_WAKEUP_STACK"=83, "REG_WAKUP_XOSU"=84, "REG_WAKUP_CNTDROPOUT"=85, "REG_WAKEUP_CRCCTRL"=86, "REG_WAKEUP_CRCWORD1"=87, "REG_WAKEUP_CRCWORD2"=88, "REG_WAKEUP_WK_RX_CTRIM"=89, "REG_WAKEUP_VDDATRIM"=90, "REG_WAKEUP_VDDDTRIM"=91, "REG_WAKEUP_TESTIOBUFEN"=92, "REG_WAKEUP_TESTIOCLAMP"=93, "CORE_RESET_ADDRESS"=94, "CHIP_RESET_ADDRESS"=95, "REG_RF_TXGENCTRL"=96, "REG_RF_TXIFCTRL"=97, "REG_RF_TXRF_SEL_CTRL"=98, "REG_RF_TXRFPWRDEFAULTSET"=99, "REG_RF_RSSITRIM"=100, "REG_RF_TXIFOSCTUNE"=101, "REG_RF_TXIFGAINIMB"=102, "REG_RF_TXIFLOCK"=103, "REG_RF_RXRFLNAGAINTRIM"=104, "REG_RF_RXBIASTR"=105, "REG_RF_RXGENCTRL"=106, "REG_RF_RXIFADCDECLEV"=107, "REG_RF_RXIFDETFILTERTUNE"=108, "REG_RF_RXIFFILTERTUNE"=109, "REG_RF_GENENABLES"=110, "REG_RF_SYNTH_CHANNEL"=111, "REG_TX_RAMP_RTRIM"=112, "REG_TX_RAMP_CTRIM"=113, "REG_RF_XO_TRIM"=114, "REG_RF_SYNTH_SET_TRIM"=115, "REG_RF_ADCCTRL"=116, "REG_RF_ADCOUTPUT"=117, "REG_RF_TXIFAMP"=118, "REG_RF_SYNTH_RTRIM"=119, "REG_RF_SYNTH_CTRIM"=120, "REG_RF_SYNTH_CT"=121, "REG_RF_TXMIXER_IOSTRIM_HIGH_IP"=122, "REG_RF_TXMIXER_IOSTRIM_HIGH_IN"=123, "REG_RF_TXMIXER_IOSTRIM_HIGH_QP"=124, "REG_RF_TXMIXER_IOSTRIM_HIGH_QN"=125, "REG_HX_WUADDR"=126, "REG_REVISION"=127, "REG_NOREG_TEST"=128, "REG_DTEST_RXBUFF"=129, "REG_RXBUFF_NEXT_BLOCK"=130, "REG_RXBUFF_FIRST_IN_PACK"=131, "REG_RXBUFF_FIRST_EMPTY"=132, "REG_MAC_BYPASS"=133, "REG_DTEST_TXBUFF"=134, "REG_TXBUFF_NEXT_BLOCK"=135, "REG_TXBUFF_FIRST_IN_PACK"=136, "REG_TXBUFF_FIRST_EMPTY"=137, "REG_DTEST_SEQ"=138, "REG_DTEST_CKCORR"=139, "REG_MAC_TOPSTATE"=140, "REG_DTEST_INTERFACE"=141, "REG_IFACE_TXRX_BYPASS"=142, "REG_MAC_TXRXWAIT"=143, "REG_MAC_TXRFRAMP"=144, "REG_MAC_TRAINWORD"=145, "REG_MAC_TRAINWORD2"=146, "REG_MAC_SETTINGS"=147, "REG_MAC_CALSELECT1"=148, "REG_MAC_CALSELECT2"=149, "REG_MAC_ANTMATCHSEL"=150, "REG_MAC_ANTTUNESEL1"=151, "REG_MAC_ANTTUNESEL2"=152, "REG_MAC_ANTTUNESEL3"=153, "REG_MAC_ANTTUNESTEP"=154, "REG_MAC_WUMODEBURST"=156, "REG_MAC_WUOFFSHORT"=157, "REG_MAC_WUOFFLONG"=158, "REG_MAC_CLKRECCTRL"=159, "REG_HK_MODE_P2"=162, "REG_MAC_ANTTUNERES1"=164, "REG_MAC_ANTTUNERES2"=165, "REG_INTERFACE_MODE_TEST"=171, "REG_TXRXBUFF_BOTH_P2"=172, "REG_TXRXBUFF_P2"=173, "REG_IRQ_RAWSTATUS1_P2"=174, "REG_MAC_TXIFSTATUS1"=176, "REG_MAC_TXIFSTATUS2"=177, "REG_IRQ_RAWSTATUS2_P2"=178, "REG_MAC_TXIFRAMPDELAY"=179, "REG_MAC_TXIFRAMPSLOPE"=180, "REG_MAX_TXIFRAMP"=181, "REG_IRQ_STATUS1_P2"=182, "REG_IRQ_STATUS2_P2"=183, "REG_IRQ_AUXSTATUS_P2"=184, "REG_MAC_UNLOCK"=188, "REG_MAC_TXIFFREQ"=190, "REG_WAKEUP_TESTCTRL1"=192, "REG_WAKEUP_RX_EN_CNT"=193, "REG_WAKEUP_TESTENABLES"=194, "REG_WAKEUP_DTBI_CTRL"=195, "REG_WAKEUP_DTBO_CTRL"=196, "REG_WAKEUP_TESTIOBUFTEST"=197, "REG_WAKEUP_WK_RX_TESTCTRL1"=198, "REG_WAKEUP_WK_RX_TESTCTRL2"=199, "REG_WAKEUP_SENS_SEQUENCE_CTRL"=200, "REG_WAKEUP_LNABIAS"=201, "REG_WAKEUP_DET_TH_TRIM1"=202, "REG_WAKEUP_LNABIAS_NOM1"=203, "REG_WAKEUP_RX_TSHORT_TRIM1"=204, "REG_WAKEUP_LNABIAS_NOM2"=205, "REG_WAKEUP_RX_TLONG_TRIM1"=206, "REG_WAKEUP_LNA_NEGRTRIM_NOM1"=207, "REG_WAKEUP_RX_TBURST_TRIM1"=208, "REG_WAKEUP_RX_LNA_NEGRTRIM_NOM2"=209, "REG_WAKEUP_RX_BB_G_BW_SEL1"=210, "REG_WAKEUP_WK_RX_DET_IOSTRIM1"=212, "REG_WAKEUP_WK_RX_CTRL2"=214, "REG_WAKEUP_WK_RX_RSSIVOSTRIM"=215, "REG_WAKEUP_LNANEGR_EFF"=216, "REG_WAKEUP_XOSU_FAST"=217, "REG_WAKEUP_STROSCPWIDTH1"=218, "REG_WAKEUP_STROSCPERIOD1"=220, "REG_WAKEUP_STROSCPERIOD2"=221, "REG_WAKEUP_WK_RX_LNA_NEGRTRIM1"=222, "REG_RF_TXTESTENABLE"=224, "REG_RF_TXIFTESTMODE"=225, "REG_RF_RXTESTENABLE"=226, "REG_RF_RXIFTESTCTRL1"=227, "REG_RF_RXIFTESTCTRL2"=228, "REG_RF_RXIFTESTCTRL3"=229, "REG_RF_SYNTH_TESTCTRL1"=230, "REG_RF_SYNTH_TESTCTRL2"=231, "REG_RF_SYNTH_TESTCTRL3"=232, "REG_RF_ADCTEST1"=237, "REG_RF_ADCTEST2"=238, "REG_RF_TXMIXER_IOSTRIM_LOW_IP"=240, "REG_RF_TXMIXER_IOSTRIM_LOW_IN"=241, "REG_RF_TXMIXER_ISOTRIM_LOW_QP"=242, "REG_RF_TXMIXER_IOSTRIM_LOW_QN"=243, "REG_RF_SYNTH_KPD"=244, "REG_RF_SYNTH_LOLEV"=245, "REG_RF_TXRFPWRTUNEANTSET"=246, "REG_RF_TXPD_GAIN_CTRL"=247, "REG_RF_SYNTH_STARTUP"=248, "REG_RF_TXRFANTTUNE_TXMODE"=249, "REG_RF_TXRFANTTUNE_RXMODE"=250, "REG_RF_RXRFANTTUNE_TXMODE"=251, "REG_RF_RXRFANTTUNE_RXMODE"=252, "REG_ANTMATCH1"=253, "REG_ANTMATCH2"=254, "REG_REVISION_P2"=255] ("Register")
              n94 = call "MICSD Get Register.vi"("Execute on Remote?(F)"=w398, "error in (no error)"=w404, "Address"=w400, "VISA Resource Name"=w399) -> ("error out"=w403:errorcluster, "Data"=→"Loopback Data":u8)  [unwired: 5 in, 1 out]
              n95 = call "MICSD Get Register.vi"("Execute on Remote?(F)"=w398, "error in (no error)"=w403, "Address"=w401, "VISA Resource Name"=w399) -> ("error out"=w402:errorcluster, "Data"=→"Retries":u8)  [unwired: 5 in, 1 out]
            }
          }
        }
      }
    }
    n96 = Unbundle By Name(w69) -> ("status"=w66:bool)
    n97 = Or(x=w66, y="Done") -> (x .or. y?=w68:bool)
  }
  n98 = call "MICSD Get Register.vi"("Execute on Remote?(F)"=w27, "error in (no error)"=w28, "Address"=w29, "VISA Resource Name"="PRIMARY MICS Dongle Address") -> ("error out"=w33:errorcluster, "Data"=w32:u8, "dup VISA Resource Name"=w34:refnum<visa-resource-name>)  [unwired: 5 in]
  n99 = And(x=u8 191 ("Data"), y=w32) -> (x .and. y?=w31:u8)
  n100 = call "MICSD Set Register.vi"("Execute on Remote?(F)"=w27, "error in (no error)"=w33, "Data"=w31, "Address"=w29, "VISA Resource Name"=w34) -> ("error out"=→"error out":errorcluster)  [unwired: 5 in, 1 out]
